vi "Omniax_mDrive_XYZR_2016.vi"() -> ()   [LabVIEW 2014]
uses:
  <vilib>/Utility/file.llb/Read From Spreadsheet File (I64).vi
  <vilib>/Utility/file.llb/Read From Spreadsheet File (string).vi
  <vilib>/Instr/_visa.llb/VISA Configure Serial Port (Instr).vi
  <vilib>/Utility/file.llb/Write To Spreadsheet File (I64).vi
  <vilib>/Utility/file.llb/Write To Spreadsheet File (string).vi
panel:
  in  "Submit":bool
  in  "ELOG":string
  out "Z max step":i32
  in  "V5 position 15360000":i32
  out "R Velocity MVdeg/sec":dbl format="%.3f"
  out "R Position MV deg":dbl
  out "Z Velocity MV mm/sec":dbl format="%.3f"
  out "Z Position MV mm":dbl
  out "Y Velocity MV mm/sec":dbl format="%.3f"
  out "Y Position MV mm":dbl
  out "X Velocity MV mm/sec":dbl format="%.3f"
  out "X Position MV mm":dbl
  out "Presets":i32[][](array[numeric])
  in  "stop":bool
  in  "Tab Control 3":enum32{"Status", "Reset"}(tab)
  out "Y in Range":bool
  out "Y Scan":bool
  out "Y in Motion":bool
  out "Y Backlash corr":bool
  out "X  in Range":bool
  out "X Scan":bool
  out "X  in Motion":bool
  out "X Backlash corr":bool
  out "Z in Range":bool
  out "Z Scan":bool
  out "Z in Motion":bool
  out "Z Backlash corr":bool
  out "R in Range":bool
  out "R Scan":bool
  out "R in Motion":bool
  out "R Backlash corr":bool
  out "X Ready":bool
  out "Y Ready":bool
  out "Z Ready":bool
  out "R Ready":bool
  in  "Reset Y Position mm":dbl
  out "Reset Y Motor Steps":i32
  in  "Reset X Position mm":dbl
  out "Reset X Motor Steps":i32
  in  "Reset Z Position mm":dbl
  out "Reset Z Motor Steps":i32
  in  "Reset R Position deg":dbl
  out "Reset R Motor Steps":i32
  in  "Reset":bool
  in  "Tab Control 2":enum32{"mm", "step"}(tab)
  in  "X Scan Length SP mm":dbl
  in  "X Scan Velocity SP mm/sec":dbl
  in  "X Scan set":bool
  in  "Y Scan Length SP mm":dbl
  in  "Y Scan Velocity SP mm/sec":dbl
  in  "Y Scan set":bool
  in  "Z Scan Length SP mm":dbl
  in  "Z Scan Velocity SP mm/sec":dbl
  in  "Z Scan set":bool
  in  "R Scan Length SP deg":dbl
  in  "R Scan Velocity SP deg/sec":dbl
  in  "R Scan set":bool
  in  "X Scan Velocity SP steps/sec":i32=1 min=1 max=102400 step=1
  in  "X Scan Length SP steps":i32 min=-2816000 max=1792000 step=100
  out "X Scan length MV mm":dbl
  out "X Scan velocity MV mm/sec":dbl format="%#_6f"
  in  "Y Scan Velocity SP steps/sec":i32=1 min=1 max=102400 step=1
  in  "Y Scan Length SP steps":i32 min=-1930240 max=2677760 step=100
  out "Y Scan length MV mm":dbl
  out "Y Scan velocity MV mm/sec":dbl format="%#_6f"
  in  "Z Scan Velocity SP steps/sec":i32=1 min=1 max=102400 step=1
  in  "Z Scan Length SP steps":i32 min=-91980800 max=10419200 step=100
  out "Z Scan length MV mm":dbl
  out "Z Scan velocity MV mm/sec":dbl format="%#_6f"
  in  "R Scan Velocity SP steps/sec":i32=1 min=1 max=102400 step=1
  in  "R Scan Length SP steps":i32 min=-1501867 max=10786133 step=100
  out "R Scan length MV deg":dbl
  out "R Scan velocity MV deg/sec":dbl format="%#_6f"
  out "atan Y/Z":dbl
  in  "Tab Control":enum32{"mm", "preset", "step"}(tab)
  in  "X Position SP mm":dbl
  in  "X Velocity SP mm/sec":dbl
  in  "X Move Set":bool
  in  "Y Move Set":bool
  in  "Y Position SP mm":dbl
  in  "Y Velocity SP mm/sec":dbl
  in  "Z Position SP mm":dbl
  in  "Z Velocity SP mm/sec":dbl
  in  "Z Move Set":bool
  in  "R Position SP deg":dbl
  in  "R Velocity SP deg/sec":dbl
  in  "R Move Set":bool
  in  "Add Button":bool
  in  "String":string
  in  "Delete Button":bool
  in  "Preset positions":i32(ring) items=["ZERO", "Default", "CDOSE", "QMS", "test", "test2", "test3", "yag position", "Sample Long Edge  ", "SPUTTER POS"]
  in  "Set Button":bool
  in  "X Velocity SP step/sec":i32 min=1 max=128000
  in  "Y Velocity SP step/sec":i32 min=1 max=128000
  in  "Z Velocity SP step/sec":i32 min=1 max=204800
  in  "R Velocity SP step/sec":i32 min=1 max=10000
  in  "Y Step SP":i32=-20000 min=-2304000 max=2304000 step=500
  in  "X Step SP":i32=-20000 min=-2304000 max=2304000 step=500
  in  "Z Step SP":i32=-20000 min=0 max=102400000 step=500
  in  "R Step SP":i32=-20000 min=-6144000 max=6144000 step=500
  out "X Step PV":i32 max=2000
  out "Y Step PV":i32 max=2000
  out "Z Step PV":i32 max=2000
  out "R Step PV":i32 max=2000
  in  "Clear ZY":bool
  out "ZY Graph":cluster{"Y":dbl[], "Y":dbl[]}[](graph)
  out "ZR Graph":cluster{"Y":dbl[], "Y":dbl[]}[](graph)
  out "XY Graph":cluster{"Y":dbl[], "Y":dbl[]}[](graph)
  out "X Scan Duration":dbl
  out "Y Scan Duration":dbl
  out "Z Scan Duration":dbl
  out "R Scan Duration":dbl
  out "R Backlash steps/sec":i32
  out "R Backlash":i32
  out "R Holding Current %":i32
  out "R Run Current %":i32
  out "R offset deg":dbl
  out "R deg/rev":dbl
  out "R steps/rev":u32
  out "R velocity PV step/sec":i32
  out "R MINPOS":i32=-94296
  out "R MAXPOS":i32=-34296
  out "R COM PORT":refnum<visa-resource-name>="COM5"
  in  "R Scan OK":bool
  in  "R Go":bool
  out "R Position deg PV":dbl
  out "Z COM PORT":refnum<visa-resource-name>="COM5"
  out "Z Backlash steps/sec":i32
  out "Z Backlash":i32
  out "Z Holding Current %":i32
  out "Z Run Current %":i32
  out "Z offset mm":dbl
  out "Z mm/rev":dbl
  out "Z steps/rev":u32
  out "Z  velocity PV step/sec":i32
  out "Z MINPOS":i32=-94296
  out "Z MAXPOS":i32=-34296
  in  "Z Scan OK":bool
  in  "Z Go":bool
  out "Z Position mm PV":dbl
  out "X Position mm PV":dbl
  out "X velocity PV step/sec":i32
  in  "X Scan OK":bool
  in  "X Go":bool
  out "X Backlash steps/sec":i32
  out "X Backlash":i32
  out "X Holding Current %":i32
  out "X Run Current %":i32
  out "X offset mm":dbl
  out "X mm/rev":dbl
  out "X steps/rev":u32
  out "X MAXPOS":i32=-34296
  out "X MINPOS":i32=-94296
  out "X COM PORT":refnum<visa-resource-name>="COM5"
  out "Y Backlash steps/sec":i32
  out "Y Backlash":i32
  out "Y Holding Current %":i32
  out "Y Run Current %":i32
  in  "Scan Cancel":bool
  out "Y Position mm PV":dbl
  out "Y offset mm":dbl
  out "Y mm/rev":dbl
  out "Y steps/rev":u32
  out "Y velocity PV step/sec":i32
  in  "Y Scan OK":bool
  in  "Scan Go":bool
  in  "Stop":bool
  in  "Y Go":bool
  out "Y MINPOS":i32=-94296
  out "Y MAXPOS":i32=-34296
  out "Y COM PORT":refnum<visa-resource-name>="COM5"
  # "12-15"
  # "Current position"
  # "Goto position"
  # "MX"
  # "MY"
  # "V5"
  # "MZ"
  # "MR"
  # "L"
  # "M"
  # "B"
  # "S"
  # "R"
  # "Preset position"
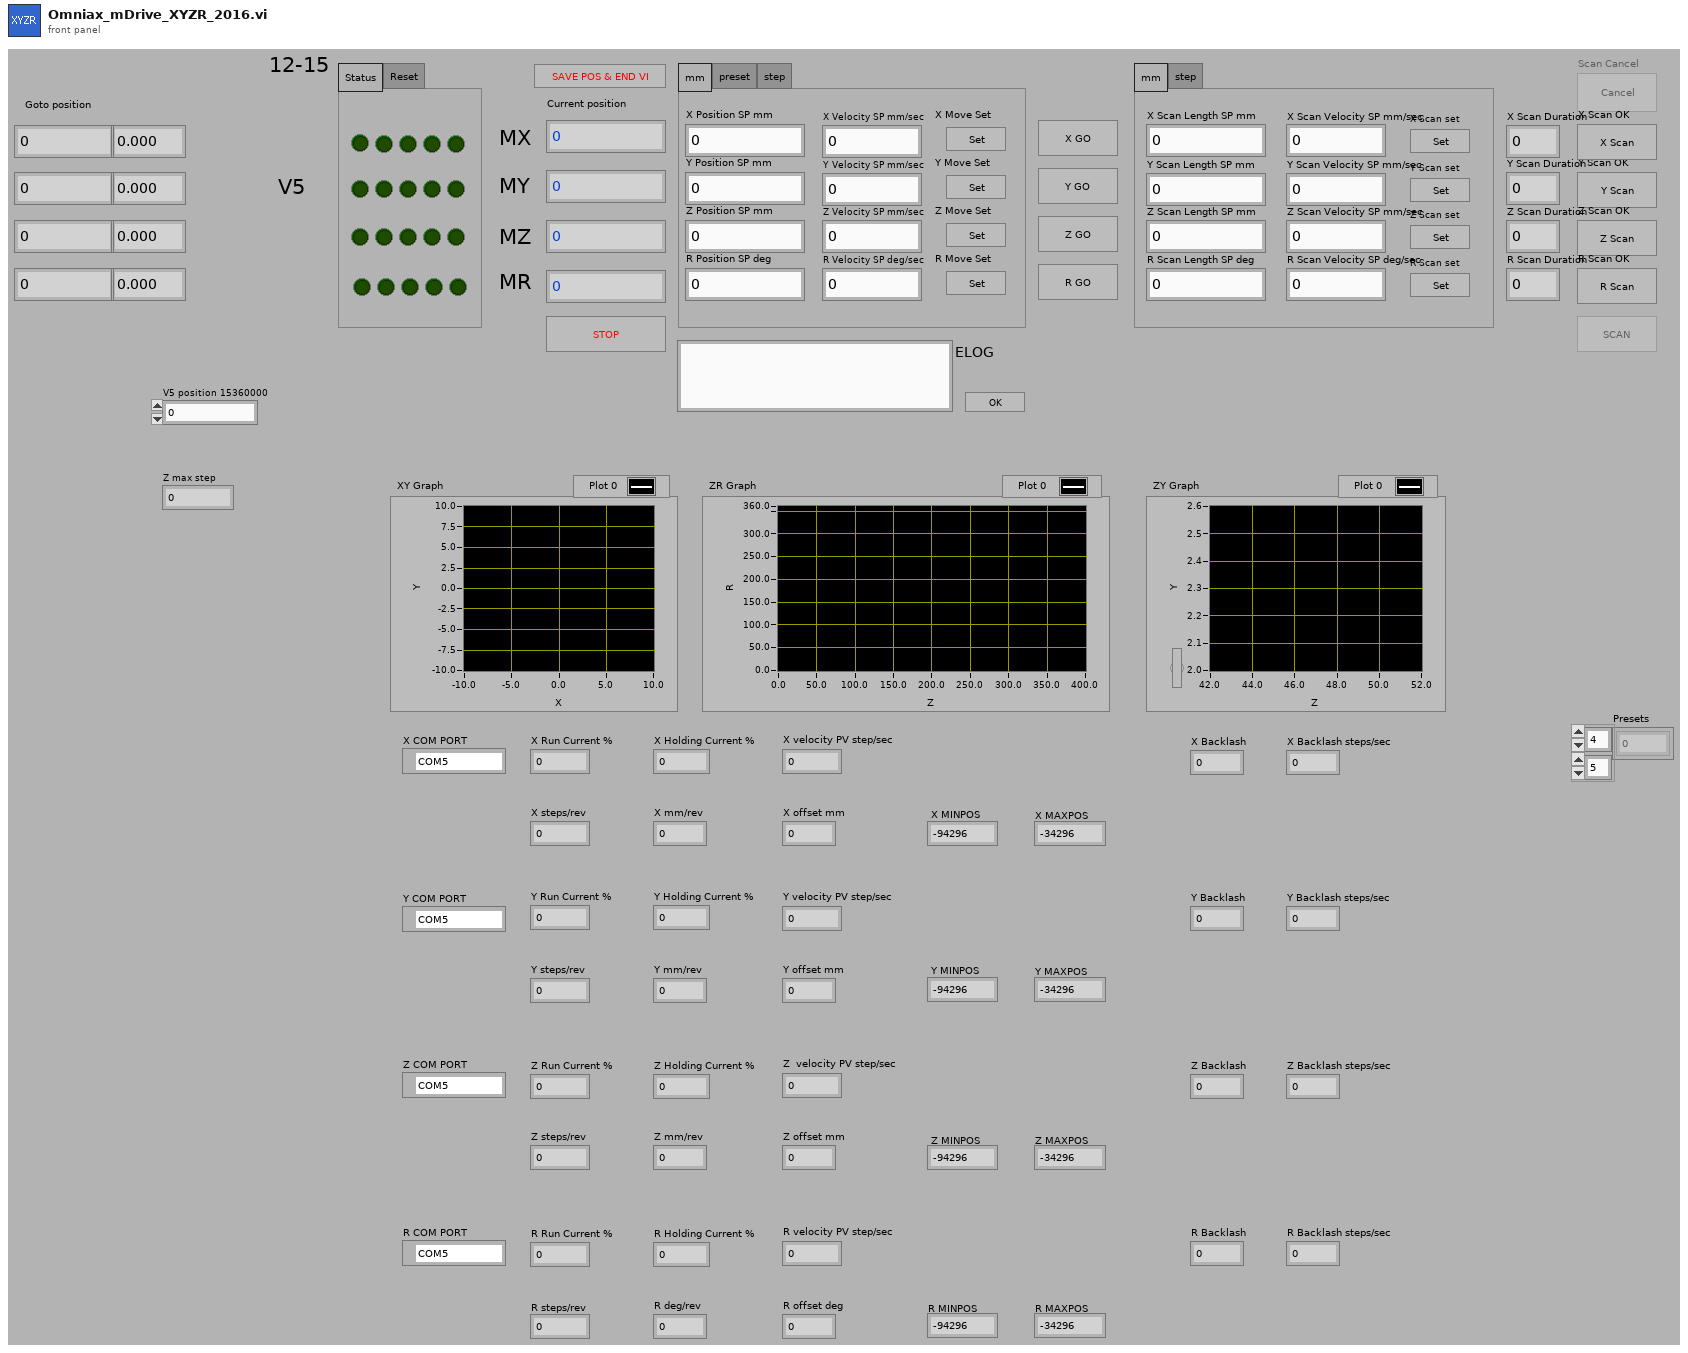
[diagram p1: front panel]
types:
  T1 = enum16{"Stop", "Reset", "Run Current", "Holding Current", "Accel Rate", "Decel Rate", "Move to Relative Position", "Move to Absolute Position", "Echo Mode", "Print Parameter", "Send String", "Microstep Resolution", "Set Current Position", "Max Velocity"}
  T2 = enum8{"Enabled", "Disabled", "Disabled and Grayed Out"}
  T3 = cluster{"first row[0]":i64, "first row[1]":i64, "first row[2]":i64, "first row[3]":i64, "first row[4]":i64, "first row[5]":i64, "first row[6]":i64, "first row[7]":i64, "first row[8]":i64}
  T4 = enum16{"open", "replace", "create", "open or create", "replace or create", "replace or create with confirmation"}
  T5 = cluster{"Value[0]":i32, "Value[1]":i32, "Value[2]":i32, "Value[3]":i32, "Value[4]":i32, "Value[5]":i32, "Value[6]":i32, "Value[7]":i32, "Value[8]":i32}
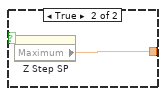
[diagram p7: hidden frame]
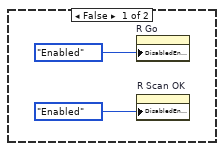
[diagram p9: hidden frame]
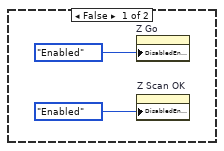
[diagram p12: hidden frame]
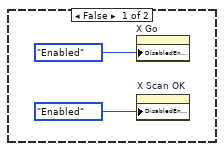
[diagram p15: hidden frame]
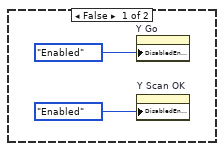
[diagram p18: hidden frame]
diagram:
  w2 = 0 ("dimension size")
  n1 = property on="R Step SP" class="DigNum (strict)"("Maximum"=6144000 ("upper limit")) -> ()  [unwired: 2 in, 2 out]
  n2 = property on="R Step SP" class="DigNum (strict)"("Minimum"=-6144000 ("lower limit")) -> ()  [unwired: 2 in, 2 out]
  n3 = call-poly <vilib>:"Read From Spreadsheet File.vi"("file path (dialog if empty)"=path "S:/SSE/IMS/PRESET.TXT") -> ("all rows"=w8:string[][])  [unwired: 6 in, 4 out]
  n4 = Transpose 2D Array(2D array=w8) -> (transposed array=w9:string[][])
  n5 = flat-sequence {
    tunnel: [w106] -> w36
    tunnel: [w105] -> w35
    tunnel: [w114] -> w54
    tunnel: [w116] -> w52
    tunnel: w36 -> [w115]
    tunnel: w35 -> [w117]
    tunnel: w54 -> [w121]
    tunnel: [w122] -> w53
    tunnel: w52 -> [w120]
    tunnel: [w123] -> w51
    tunnel: [w134] -> w71
    tunnel: [w136] -> w70
    tunnel: w53 -> [w135]
    tunnel: w51 -> [w130]
    tunnel: w71 -> [w143]
    tunnel: [w142] -> w69
    tunnel: w70 -> [w140]
    tunnel: [w141] -> w68
    tunnel: [w153] -> w67
    tunnel: [w154] -> w66
    tunnel: w69 -> [w152]
    tunnel: w68 -> [w151]
    tunnel: w67 -> [w164]
    tunnel: w66 -> [w163]
    tunnel: [w166] -> w65
    tunnel: [w165] -> w64
    tunnel: [w160] -> w63
    tunnel: [w173] -> w59
    tunnel: [w174] -> w60
    tunnel: w65 -> [w174]
    tunnel: w64 -> [w173]
    tunnel: w63 -> [w171]
    frame #0 {
      w113 = refnum<visa-resource-name> "COM13" ("COM PORT")
      w111 = u16 0 items=["None", "XON/XOFF", "RTS/CTS", "XON/XOFF & RTS/CTS", "DTR/DSR", "XON/XOFF & DTR/DSR"] ("flow control (0:none)")
      w110 = u16 10 items=["1.0"=10, "1.5"=15, "2.0"=20] ("stop bits (10: 1 bit)")
      # "Stop bits"
      n6 = call-poly "VISA Configure Serial Port"("VISA resource name"=w113, "timeout (10sec)"=u32 10000, "baud rate (9600)"=u32 9600, "data bits (8)"=u16 8, "parity (0:none)"=enum16{"None", "Odd", "Even", "Mark", "Space"}."None", "stop bits (10: 1 bit)"=w110, "flow control (0:none)"=w111) -> ("VISA resource name out"=w106:refnum<visa-resource-name>, "error out"=w105:errorcluster)  [unwired: 7 in]
      "R COM PORT" <- w113
    }
    frame #1 {
      n7 = call "mDrive Send Command.vi"("error in (no error)"=w117, "Extra"="EM=2", "Command"=T1."Send String", "VISA resource name"=w115) -> ("error out"=w116:errorcluster, "VISA resource name out"=w114:refnum<visa-resource-name>)  [unwired: 3 in, 1 out]
    }
    frame #2 {
      # "pr=1000000"
      n8 = Number To Decimal String(number=100000) -> (decimal integer string=w125:string)  [unwired: 1 in]
      n9 = call "mDrive Send Command.vi"("error in (no error)"=w120, "Extra"=w125, "Command"=T1."Accel Rate", "VISA resource name"=w121) -> ("error out"=w124:errorcluster, "VISA resource name out"=w129:refnum<visa-resource-name>)  [unwired: 3 in, 1 out]
      n10 = call "mDrive Send Command.vi"("error in (no error)"=w124, "Extra"=w125, "Command"=T1."Decel Rate", "VISA resource name"=w129) -> ("error out"=w123:errorcluster, "VISA resource name out"=w122:refnum<visa-resource-name>)  [unwired: 3 in, 1 out]
    }
    frame #3 {
      # "Run Current %"
      n11 = property on="R Run Current %" class="DigNum (strict)"() -> ("Value"=w132:i32)  [unwired: 2 in, 2 out]
      n12 = Number To Decimal String(number=w132) -> (decimal integer string=w133:string)  [unwired: 1 in]
      n13 = call "mDrive Send Command.vi"("error in (no error)"=w130, "Extra"=w133, "Command"=T1."Run Current", "VISA resource name"=w135) -> ("error out"=w136:errorcluster, "VISA resource name out"=w134:refnum<visa-resource-name>)  [unwired: 3 in, 1 out]
    }
    frame #4 {
      # "Holding Current %"
      n14 = property on="R Holding Current %" class="DigNum (strict)"() -> ("Value"=w138:i32)  [unwired: 2 in, 2 out]
      n15 = Number To Decimal String(number=w138) -> (decimal integer string=w139:string)  [unwired: 1 in]
      n16 = call "mDrive Send Command.vi"("error in (no error)"=w140, "Extra"=w139, "Command"=T1."Holding Current", "VISA resource name"=w143) -> ("error out"=w141:errorcluster, "VISA resource name out"=w142:refnum<visa-resource-name>)  [unwired: 3 in, 1 out]
    }
    frame #5 {
      # "Print Velocity Max"
      # "Velocity Max"
      n17 = property on="R Velocity SP step/sec" class="DigNum (strict)"() -> ("Value"=w150:i32)  [unwired: 2 in, 2 out]
      n18 = Number To Decimal String(number=w150) -> (decimal integer string=w149:string)  [unwired: 1 in]
      n19 = call "mDrive Send Command.vi"("error in (no error)"=w151, "Extra"=w149, "Command"=T1."Max Velocity", "VISA resource name"=w152) -> ("error out"=w147:errorcluster, "VISA resource name out"=w157:refnum<visa-resource-name>)  [unwired: 3 in, 1 out]
      n20 = call "mDrive Send Command.vi"("error in (no error)"=w147, "Extra"="VM", "Command"=T1."Print Parameter", "VISA resource name"=w157) -> ("error out"=w154:errorcluster, "read buffer"=w155:string, "VISA resource name out"=w153:refnum<visa-resource-name>)  [unwired: 3 in]
      n21 = Decimal String To Number(string=w155, offset=0) -> (number=w148:i32)  [unwired: 1 in, 1 out]
      n22 = property on="R velocity PV step/sec" class="DigNum (strict)"("Val(Sgnl)"=w148) -> ()  [unwired: 2 in, 2 out]
    }
    frame #6 {
      # "PRINT POSITION"
      n23 = call "mDrive Send Command.vi"("error in (no error)"=w163, "Extra"="P", "Command"=T1."Print Parameter", "VISA resource name"=w164) -> ("error out"=w165:errorcluster, "read buffer"=w162:string, "VISA resource name out"=w166:refnum<visa-resource-name>)  [unwired: 3 in]
      n24 = Decimal String To Number(string=w162, offset=0) -> (number=w160:i32)  [unwired: 1 in, 1 out]
    }
    frame #7 {
      n25 = property on="R Step SP" class="DigNum (strict)"("Val(Sgnl)"=w171) -> ()  [unwired: 2 in, 2 out]
      n26 = property on="R Step SP" class="DigNum (strict)"() -> ("Maximum"=w170:dbl)  [unwired: 2 in, 2 out]
      n27 = property on="R Step SP" class="DigNum (strict)"() -> ("Minimum"=w169:dbl)  [unwired: 2 in, 2 out]
      n28 = To Long Integer(number=w170) -> (32bit integer=w167:i32)
      "R MAXPOS" <- w167
      n29 = To Long Integer(number=w169) -> (32bit integer=w168:i32)
      "R MINPOS" <- w168
      n30 = In Range and Coerce(upper limit=w167, x=w171, lower limit=w168) -> (In Range?=w172:bool)  [unwired: 1 out]
      n31 = property on="R in Range" class="Bool (strict)"("Val(Sgnl)"=w172) -> ()  [unwired: 2 in, 2 out]
    }
  }
  n32 = flat-sequence {
    frame #0 {
      w180 = -3.0 ("R deg/rev")
      w178 = u32 51200 ("step/rev")
      w182 = 10000 ("Value (Signaling)")
      n33 = To Double Precision Float(number=w182) -> (double precision float=w184:dbl)
      n34 = To Double Precision Float(number=w178) -> (double precision float=w179:dbl)
      n35 = property on="R Velocity SP step/sec" class="DigNum (strict)"("Val(Sgnl)"=w182) -> ()  [unwired: 2 in, 2 out]
      n36 = property on="R Velocity SP step/sec" class="DigNum (strict)"("Minimum"=1.0 ("Data Entry Limits:Minimum")) -> ()  [unwired: 2 in, 2 out]
      n37 = Divide(x=w184, y=w179) -> (x/y=w183:dbl)
      n38 = property on="R Velocity SP step/sec" class="DigNum (strict)"("Maximum"=w184) -> ()  [unwired: 2 in, 2 out]
      n39 = Multiply(x=w183, y=w180) -> (x*y=w181:dbl)
      n40 = Absolute Value(x=w181) -> (abs(x)=w175:dbl)
      n41 = property on="R Velocity SP deg/sec" class="DigNum (strict)"("Val(Sgnl)"=w175) -> ()  [unwired: 2 in, 2 out]
      "R offset deg" <- 0.0 ("R offset deg")
      "R deg/rev" <- w180
      "R steps/rev" <- w178
    }
  }
  n42 = flat-sequence {
    frame #0 {
      w186 = 0.2 ("Z mm/rev")
      w185 = u32 51200 ("step/rev")
      w187 = 204800 ("Value (Signaling)")
      n43 = To Double Precision Float(number=w187) -> (double precision float=w191:dbl)
      n44 = To Double Precision Float(number=w185) -> (double precision float=w190:dbl)
      n45 = property on="Z Velocity SP step/sec" class="DigNum (strict)"("Val(Sgnl)"=w187) -> ()  [unwired: 2 in, 2 out]
      n46 = property on="Z Velocity SP step/sec" class="DigNum (strict)"("Minimum"=1.0 ("Data Entry Limits:Minimum")) -> ()  [unwired: 2 in, 2 out]
      n47 = Divide(x=w191, y=w190) -> (x/y=w188:dbl)
      n48 = property on="Z Velocity SP step/sec" class="DigNum (strict)"("Maximum"=w191) -> ()  [unwired: 2 in, 2 out]
      n49 = Multiply(x=w188, y=w186) -> (x*y=w189:dbl)
      n50 = property on="Z Velocity SP mm/sec" class="DigNum (strict)"("Val(Sgnl)"=w189) -> ()  [unwired: 2 in, 2 out]
      "Z offset mm" <- 0.0 ("Z offset mm")
      "Z mm/rev" <- w186
      "Z steps/rev" <- w185
    }
  }
  n51 = flat-sequence {
    frame #0 {
      n52 = property on="X Backlash corr" class="Bool (strict)"("Val(Sgnl)"=FALSE ("Value (Signaling)")) -> ()  [unwired: 2 in, 2 out]
      n53 = property on="Y Backlash corr" class="Bool (strict)"("Val(Sgnl)"=FALSE ("Value (Signaling)")) -> ()  [unwired: 2 in, 2 out]
      n54 = property on="R Backlash corr" class="Bool (strict)"("Val(Sgnl)"=FALSE ("Value (Signaling)")) -> ()  [unwired: 2 in, 2 out]
      n55 = property on="Z Backlash corr" class="Bool (strict)"("Val(Sgnl)"=FALSE ("Value (Signaling)")) -> ()  [unwired: 2 in, 2 out]
      "Z Backlash steps/sec" <- 25600 ("Z Backlash steps/sec")
      "Z Backlash" <- -51200 ("Z Backlash")
      "X Backlash steps/sec" <- 25600 ("Value (Signaling)")
      "X Backlash" <- 10240 ("Backlash2")
      "Y Backlash" <- -10240 ("Backlash2")
      "Y Backlash steps/sec" <- 25600 ("Value (Signaling)")
      "R Backlash steps/sec" <- 6400 ("R Backlash steps/sec")
      "R Backlash" <- -12800 ("R Backlash")
    }
  }
  n56 = flat-sequence {
    frame #0 {
      "Z Holding Current %" <- 20 ("Z Holding Current %")
      "Z Run Current %" <- 40 ("Z Run Current %")
      "X Run Current %" <- 40 ("Run Current %")
      "X Holding Current %" <- 20 ("Holding Current %")
      "Y Run Current %" <- 40 ("Run Current %")
      "Y Holding Current %" <- 20 ("Holding Current %")
      "R Holding Current %" <- 15 ("R Holding Current %")
      "R Run Current %" <- 80 ("R Run Current %")
    }
  }
  n57 = flat-sequence {
    frame #0 {
      n58 = property on="Y Scan" class="Bool (strict)"("Val(Sgnl)"=FALSE ("Value (Signaling)")) -> ()  [unwired: 2 in, 2 out]
      n59 = property on="X Scan Velocity SP mm/sec" class="DigNum (strict)"("Val(Sgnl)"=0.1 ("Value (Signaling)")) -> ()  [unwired: 2 in, 2 out]
      n60 = property on="Z Scan" class="Bool (strict)"("Val(Sgnl)"=FALSE ("Value (Signaling)")) -> ()  [unwired: 2 in, 2 out]
      n61 = property on="X Scan" class="Bool (strict)"("Val(Sgnl)"=FALSE ("Value (Signaling)")) -> ()  [unwired: 2 in, 2 out]
      n62 = property on="Z Scan Velocity SP mm/sec" class="DigNum (strict)"("Val(Sgnl)"=0.1 ("Value (Signaling)")) -> ()  [unwired: 2 in, 2 out]
      n63 = property on="R Velocity SP deg/sec" class="DigNum (strict)"("Val(Sgnl)"=0.1 ("Value (Signaling)")) -> ()  [unwired: 2 in, 2 out]
      n64 = property on="R Scan" class="Bool (strict)"("Val(Sgnl)"=FALSE ("Value (Signaling)")) -> ()  [unwired: 2 in, 2 out]
      n65 = property on="Y Scan Velocity SP mm/sec" class="DigNum (strict)"("Val(Sgnl)"=0.1 ("Value (Signaling)")) -> ()  [unwired: 2 in, 2 out]
      n66 = property on="Scan Go" class="Bool"("DisabledEnum"=T2."Disabled and Grayed Out" ("Disabled")) -> ()  [unwired: 2 in, 2 out]
      n67 = property on="Scan Cancel" class="Bool"("DisabledEnum"=T2."Disabled and Grayed Out" ("Disabled")) -> ()  [unwired: 2 in, 2 out]
    }
  }
  n68 = flat-sequence {
    frame #0 {
      w226 = 0.2 ("MM/rev")
      w229 = u32 51200 ("step/rev")
      w224 = 128000 ("Value (Signaling)")
      # "a=1000000"
      n69 = property on="X Velocity SP step/sec" class="DigNum (strict)"("Minimum"=1.0 ("Data Entry Limits:Minimum")) -> ()  [unwired: 2 in, 2 out]
      n70 = To Double Precision Float(number=w224) -> (double precision float=w230:dbl)
      n71 = To Double Precision Float(number=w229) -> (double precision float=w228:dbl)
      n72 = property on="X Velocity SP step/sec" class="DigNum (strict)"("Val(Sgnl)"=w224) -> ()  [unwired: 2 in, 2 out]
      n73 = Divide(x=w230, y=w228) -> (x/y=w225:dbl)
      n74 = property on="X Velocity SP step/sec" class="DigNum (strict)"("Maximum"=w230) -> ()  [unwired: 2 in, 2 out]
      n75 = Multiply(x=w225, y=w226) -> (x*y=w227:dbl)
      n76 = property on="X Velocity SP mm/sec" class="DigNum (strict)"("Val(Sgnl)"=w227) -> ()  [unwired: 2 in, 2 out]
      "X offset mm" <- 0.0 ("offset")
      "X steps/rev" <- w229
      "X mm/rev" <- w226
    }
  }
  n77 = flat-sequence {
    frame #0 {
      w235 = 0.2 ("MM/rev")
      w238 = u32 51200 ("step/rev")
      w233 = 128000 ("Value (Signaling)")
      n78 = To Double Precision Float(number=w233) -> (double precision float=w239:dbl)
      n79 = To Double Precision Float(number=w238) -> (double precision float=w237:dbl)
      n80 = property on="Y Velocity SP step/sec" class="DigNum (strict)"("Minimum"=1.0 ("Data Entry Limits:Minimum")) -> ()  [unwired: 2 in, 2 out]
      n81 = property on="Y Velocity SP step/sec" class="DigNum (strict)"("Val(Sgnl)"=w233) -> ()  [unwired: 2 in, 2 out]
      n82 = Divide(x=w239, y=w237) -> (x/y=w234:dbl)
      n83 = property on="Y Velocity SP step/sec" class="DigNum (strict)"("Maximum"=w239) -> ()  [unwired: 2 in, 2 out]
      n84 = Multiply(x=w234, y=w235) -> (x*y=w236:dbl)
      n85 = property on="Y Velocity SP mm/sec" class="DigNum (strict)"("Val(Sgnl)"=w236) -> ()  [unwired: 2 in, 2 out]
      "Y offset mm" <- 0.0 ("offset")
      "Y steps/rev" <- w238
      "Y mm/rev" <- w235
    }
  }
  n86 = flat-sequence {
    tunnel: [w242] -> w40
    tunnel: [w243] -> w39
    tunnel: [w253] -> w46
    tunnel: [w252] -> w44
    tunnel: w40 -> [w254]
    tunnel: w39 -> [w251]
    tunnel: w46 -> [w264]
    tunnel: [w259] -> w45
    tunnel: w44 -> [w263]
    tunnel: [w263] -> w43
    tunnel: [w268] -> w80
    tunnel: [w270] -> w79
    tunnel: w45 -> [w269]
    tunnel: w43 -> [w271]
    tunnel: w80 -> [w278]
    tunnel: [w277] -> w78
    tunnel: w79 -> [w275]
    tunnel: [w276] -> w77
    tunnel: [w288] -> w76
    tunnel: [w289] -> w75
    tunnel: w78 -> [w287]
    tunnel: w77 -> [w286]
    tunnel: w76 -> [w299]
    tunnel: w75 -> [w298]
    tunnel: [w301] -> w74
    tunnel: [w300] -> w73
    tunnel: [w295] -> w72
    tunnel: [w308] -> w61
    tunnel: [w309] -> w62
    tunnel: w74 -> [w309]
    tunnel: w73 -> [w308]
    tunnel: w72 -> [w306]
    frame #0 {
      w250 = refnum<visa-resource-name> "COM14" ("COM PORT")
      w248 = u16 0 items=["None", "XON/XOFF", "RTS/CTS", "XON/XOFF & RTS/CTS", "DTR/DSR", "XON/XOFF & DTR/DSR"] ("flow control (0:none)")
      w247 = u16 10 items=["1.0"=10, "1.5"=15, "2.0"=20] ("stop bits (10: 1 bit)")
      # "Stop bits"
      n87 = call-poly "VISA Configure Serial Port"("VISA resource name"=w250, "timeout (10sec)"=u32 10000, "baud rate (9600)"=u32 9600, "data bits (8)"=u16 8, "parity (0:none)"=enum16{"None", "Odd", "Even", "Mark", "Space"}."None", "stop bits (10: 1 bit)"=w247, "flow control (0:none)"=w248) -> ("VISA resource name out"=w242:refnum<visa-resource-name>, "error out"=w243:errorcluster)  [unwired: 7 in]
      "Z COM PORT" <- w250
    }
    frame #1 {
      n88 = call "mDrive Send Command.vi"("error in (no error)"=w251, "Extra"="EM=2", "Command"=T1."Send String", "VISA resource name"=w254) -> ("error out"=w252:errorcluster, "VISA resource name out"=w253:refnum<visa-resource-name>)  [unwired: 3 in, 1 out]
    }
    frame #2 {
      n89 = Number To Decimal String(number=1000000) -> (decimal integer string=w257:string)  [unwired: 1 in]
      n90 = call "mDrive Send Command.vi"("Extra"=w257, "Command"=T1."Accel Rate", "VISA resource name"=w264) -> ("VISA resource name out"=w262:refnum<visa-resource-name>)  [unwired: 4 in, 2 out]
      n91 = call "mDrive Send Command.vi"("Extra"=w257, "Command"=T1."Decel Rate", "VISA resource name"=w262) -> ("VISA resource name out"=w259:refnum<visa-resource-name>)  [unwired: 4 in, 2 out]
    }
    frame #3 {
      # "Run Current %"
      n92 = property on="Z Run Current %" class="DigNum (strict)"() -> ("Value"=w266:i32)  [unwired: 2 in, 2 out]
      n93 = Number To Decimal String(number=w266) -> (decimal integer string=w267:string)  [unwired: 1 in]
      n94 = call "mDrive Send Command.vi"("error in (no error)"=w271, "Extra"=w267, "Command"=T1."Run Current", "VISA resource name"=w269) -> ("error out"=w270:errorcluster, "VISA resource name out"=w268:refnum<visa-resource-name>)  [unwired: 3 in, 1 out]
    }
    frame #4 {
      # "Holding Current %"
      n95 = property on="Z Run Current %" class="DigNum (strict)"() -> ("Value"=w273:i32)  [unwired: 2 in, 2 out]
      n96 = Number To Decimal String(number=w273) -> (decimal integer string=w274:string)  [unwired: 1 in]
      n97 = call "mDrive Send Command.vi"("error in (no error)"=w275, "Extra"=w274, "Command"=T1."Holding Current", "VISA resource name"=w278) -> ("error out"=w276:errorcluster, "VISA resource name out"=w277:refnum<visa-resource-name>)  [unwired: 3 in, 1 out]
    }
    frame #5 {
      # "Velocity Max"
      n98 = property on="Z Velocity SP step/sec" class="DigNum (strict)"() -> ("Value"=w285:i32)  [unwired: 2 in, 2 out]
      n99 = Number To Decimal String(number=w285) -> (decimal integer string=w284:string)  [unwired: 1 in]
      n100 = call "mDrive Send Command.vi"("error in (no error)"=w286, "Extra"=w284, "Command"=T1."Max Velocity", "VISA resource name"=w287) -> ("error out"=w282:errorcluster, "VISA resource name out"=w292:refnum<visa-resource-name>)  [unwired: 3 in, 1 out]
      n101 = call "mDrive Send Command.vi"("error in (no error)"=w282, "Extra"="VM", "Command"=T1."Print Parameter", "VISA resource name"=w292) -> ("error out"=w289:errorcluster, "read buffer"=w290:string, "VISA resource name out"=w288:refnum<visa-resource-name>)  [unwired: 3 in]
      n102 = Decimal String To Number(string=w290, offset=0) -> (number=w283:i32)  [unwired: 1 in, 1 out]
      n103 = property on="Z  velocity PV step/sec" class="DigNum (strict)"("Val(Sgnl)"=w283) -> ()  [unwired: 2 in, 2 out]
    }
    frame #6 {
      # "PRINT POSITION"
      n104 = call "mDrive Send Command.vi"("error in (no error)"=w298, "Extra"="P", "Command"=T1."Print Parameter", "VISA resource name"=w299) -> ("error out"=w300:errorcluster, "read buffer"=w297:string, "VISA resource name out"=w301:refnum<visa-resource-name>)  [unwired: 3 in]
      n105 = Decimal String To Number(string=w297, offset=0) -> (number=w295:i32)  [unwired: 1 in, 1 out]
    }
    frame #7 {
      n106 = property on="Z Step SP" class="DigNum (strict)"("Val(Sgnl)"=w306) -> ()  [unwired: 2 in, 2 out]
      n107 = property on="Z Step SP" class="DigNum (strict)"() -> ("Maximum"=w303:dbl)  [unwired: 2 in, 2 out]
      n108 = property on="Z Step SP" class="DigNum (strict)"() -> ("Minimum"=w305:dbl)  [unwired: 2 in, 2 out]
      n109 = To Long Integer(number=w303) -> (32bit integer=w304:i32)
      "Z MAXPOS" <- w304
      n110 = To Long Integer(number=w305) -> (32bit integer=w302:i32)
      "Z MINPOS" <- w302
      n111 = In Range and Coerce(upper limit=w304, x=w306, lower limit=w302) -> (In Range?=w307:bool)  [unwired: 1 out]
      n112 = property on="Z in Range" class="Bool (strict)"("Val(Sgnl)"=w307) -> ()  [unwired: 2 in, 2 out]
    }
  }
  n113 = flat-sequence {
    tunnel: [w311] -> w34
    tunnel: [w310] -> w33
    tunnel: [w321] -> w50
    tunnel: [w319] -> w48
    tunnel: w34 -> [w322]
    tunnel: w33 -> [w320]
    tunnel: w50 -> [w328]
    tunnel: [w329] -> w49
    tunnel: w48 -> [w325]
    tunnel: [w327] -> w47
    tunnel: [w338] -> w100
    tunnel: [w340] -> w98
    tunnel: w49 -> [w339]
    tunnel: w47 -> [w341]
    tunnel: w100 -> [w348]
    tunnel: [w347] -> w99
    tunnel: w98 -> [w345]
    tunnel: [w346] -> w97
    tunnel: [w358] -> w102
    tunnel: [w359] -> w101
    tunnel: w99 -> [w357]
    tunnel: w97 -> [w356]
    tunnel: w102 -> [w369]
    tunnel: w101 -> [w368]
    tunnel: [w371] -> w86
    tunnel: [w370] -> w85
    tunnel: [w365] -> w84
    tunnel: [w376] -> w103
    tunnel: [w377] -> w104
    tunnel: w86 -> [w377]
    tunnel: w85 -> [w376]
    tunnel: w84 -> [w372]
    frame #0 {
      w318 = refnum<visa-resource-name> "COM13" ("COM PORT")
      w316 = u16 0 items=["None", "XON/XOFF", "RTS/CTS", "XON/XOFF & RTS/CTS", "DTR/DSR", "XON/XOFF & DTR/DSR"] ("flow control (0:none)")
      w315 = u16 10 items=["1.0"=10, "1.5"=15, "2.0"=20] ("stop bits (10: 1 bit)")
      # "Stop bits"
      n114 = call-poly "VISA Configure Serial Port"("VISA resource name"=w318, "timeout (10sec)"=u32 10000, "baud rate (9600)"=u32 9600, "data bits (8)"=u16 8, "parity (0:none)"=enum16{"None", "Odd", "Even", "Mark", "Space"}."None", "stop bits (10: 1 bit)"=w315, "flow control (0:none)"=w316) -> ("VISA resource name out"=w311:refnum<visa-resource-name>, "error out"=w310:errorcluster)  [unwired: 7 in]
      "Y COM PORT" <- w318
    }
    frame #1 {
      n115 = call "mDrive Send Command.vi"("error in (no error)"=w320, "Extra"="EM=2", "Command"=T1."Send String", "VISA resource name"=w322) -> ("error out"=w319:errorcluster, "VISA resource name out"=w321:refnum<visa-resource-name>)  [unwired: 3 in, 1 out]
    }
    frame #2 {
      n116 = Number To Decimal String(number=1000000) -> (decimal integer string=w330:string)  [unwired: 1 in]
      n117 = call "mDrive Send Command.vi"("error in (no error)"=w325, "Extra"=w330, "Command"=T1."Accel Rate", "VISA resource name"=w328) -> ("error out"=w326:errorcluster, "VISA resource name out"=w334:refnum<visa-resource-name>)  [unwired: 3 in, 1 out]
      n118 = call "mDrive Send Command.vi"("error in (no error)"=w326, "Extra"=w330, "Command"=T1."Decel Rate", "VISA resource name"=w334) -> ("error out"=w327:errorcluster, "VISA resource name out"=w329:refnum<visa-resource-name>)  [unwired: 3 in, 1 out]
    }
    frame #3 {
      # "Run Current %"
      n119 = property on="Y Run Current %" class="DigNum (strict)"() -> ("Value"=w336:i32)  [unwired: 2 in, 2 out]
      n120 = Number To Decimal String(number=w336) -> (decimal integer string=w337:string)  [unwired: 1 in]
      n121 = call "mDrive Send Command.vi"("error in (no error)"=w341, "Extra"=w337, "Command"=T1."Run Current", "VISA resource name"=w339) -> ("error out"=w340:errorcluster, "VISA resource name out"=w338:refnum<visa-resource-name>)  [unwired: 3 in, 1 out]
    }
    frame #4 {
      # "Holding Current %"
      n122 = property on="Y Holding Current %" class="DigNum (strict)"() -> ("Value"=w343:i32)  [unwired: 2 in, 2 out]
      n123 = Number To Decimal String(number=w343) -> (decimal integer string=w344:string)  [unwired: 1 in]
      n124 = call "mDrive Send Command.vi"("error in (no error)"=w345, "Extra"=w344, "Command"=T1."Holding Current", "VISA resource name"=w348) -> ("error out"=w346:errorcluster, "VISA resource name out"=w347:refnum<visa-resource-name>)  [unwired: 3 in, 1 out]
    }
    frame #5 {
      # "Velocity Max"
      n125 = property on="Y Velocity SP step/sec" class="DigNum (strict)"() -> ("Value"=w355:i32)  [unwired: 2 in, 2 out]
      n126 = Number To Decimal String(number=w355) -> (decimal integer string=w354:string)  [unwired: 1 in]
      n127 = call "mDrive Send Command.vi"("error in (no error)"=w356, "Extra"=w354, "Command"=T1."Max Velocity", "VISA resource name"=w357) -> ("error out"=w352:errorcluster, "VISA resource name out"=w362:refnum<visa-resource-name>)  [unwired: 3 in, 1 out]
      n128 = call "mDrive Send Command.vi"("error in (no error)"=w352, "Extra"="VM", "Command"=T1."Print Parameter", "VISA resource name"=w362) -> ("error out"=w359:errorcluster, "read buffer"=w360:string, "VISA resource name out"=w358:refnum<visa-resource-name>)  [unwired: 3 in]
      n129 = Decimal String To Number(string=w360, offset=0) -> (number=w353:i32)  [unwired: 1 in, 1 out]
      n130 = property on="Y scan velocity MV step/sec" class="DigNum (strict)"("Val(Sgnl)"=w353) -> ()  [unwired: 2 in, 2 out]
    }
    frame #6 {
      # "PRINT POSITION"
      n131 = call "mDrive Send Command.vi"("error in (no error)"=w368, "Extra"="P", "Command"=T1."Print Parameter", "VISA resource name"=w369) -> ("error out"=w370:errorcluster, "read buffer"=w367:string, "VISA resource name out"=w371:refnum<visa-resource-name>)  [unwired: 3 in]
      n132 = Decimal String To Number(string=w367, offset=0) -> (number=w365:i32)  [unwired: 1 in, 1 out]
    }
    frame #7 {
      w374 = -2304000 ("lower limit")
      w375 = 2304000 ("upper limit")
      n133 = property on="Y Step SP" class="DigNum (strict)"("Val(Sgnl)"=w372) -> ()  [unwired: 2 in, 2 out]
      n134 = property on="Y Step SP" class="DigNum (strict)"("Maximum"=w375) -> ()  [unwired: 2 in, 2 out]
      n135 = property on="Y Step SP" class="DigNum (strict)"("Minimum"=w374) -> ()  [unwired: 2 in, 2 out]
      n136 = In Range and Coerce(upper limit=w375, x=w372, lower limit=w374) -> (In Range?=w373:bool)  [unwired: 1 out]
      n137 = property on="Y in Range" class="Bool (strict)"("Val(Sgnl)"=w373) -> ()  [unwired: 2 in, 2 out]
      "Y MINPOS" <- w374
      "Y MAXPOS" <- w375
    }
  }
  n138 = property on="Z Step SP" class="DigNum (strict)"("Minimum"=0 ("lower limit")) -> ()  [unwired: 2 in, 2 out]
  n139 = Delete From Array(array=w9, index (row)=0) -> (deleted portion=w10:string[], array with subset deleted=w12:string[][])  [unwired: 2 in]
  n140 = flat-sequence {
    tunnel: [w379] -> w38
    tunnel: [w378] -> w37
    tunnel: [w389] -> w58
    tunnel: [w387] -> w56
    tunnel: w38 -> [w390]
    tunnel: w37 -> [w388]
    tunnel: w58 -> [w394]
    tunnel: [w393] -> w57
    tunnel: w56 -> [w395]
    tunnel: [w397] -> w55
    tunnel: [w406] -> w96
    tunnel: [w408] -> w95
    tunnel: w57 -> [w407]
    tunnel: w55 -> [w409]
    tunnel: w96 -> [w416]
    tunnel: [w415] -> w94
    tunnel: w95 -> [w413]
    tunnel: [w414] -> w93
    tunnel: [w426] -> w92
    tunnel: [w427] -> w91
    tunnel: w94 -> [w425]
    tunnel: w93 -> [w424]
    tunnel: w92 -> [w437]
    tunnel: w91 -> [w436]
    tunnel: [w439] -> w83
    tunnel: [w438] -> w82
    tunnel: [w433] -> w81
    tunnel: [w444] -> w89
    tunnel: [w445] -> w90
    tunnel: w83 -> [w445]
    tunnel: w82 -> [w444]
    tunnel: w81 -> [w440]
    frame #0 {
      w386 = refnum<visa-resource-name> "COM12" ("COM PORT")
      w384 = u16 0 items=["None", "XON/XOFF", "RTS/CTS", "XON/XOFF & RTS/CTS", "DTR/DSR", "XON/XOFF & DTR/DSR"] ("flow control (0:none)")
      w383 = u16 10 items=["1.0"=10, "1.5"=15, "2.0"=20] ("stop bits (10: 1 bit)")
      # "Stop bits"
      n141 = call-poly "VISA Configure Serial Port"("VISA resource name"=w386, "timeout (10sec)"=u32 10000, "baud rate (9600)"=u32 9600, "data bits (8)"=u16 8, "parity (0:none)"=enum16{"None", "Odd", "Even", "Mark", "Space"}."None", "stop bits (10: 1 bit)"=w383, "flow control (0:none)"=w384) -> ("VISA resource name out"=w379:refnum<visa-resource-name>, "error out"=w378:errorcluster)  [unwired: 7 in]
      "X COM PORT" <- w386
    }
    frame #1 {
      n142 = call "mDrive Send Command.vi"("error in (no error)"=w388, "Extra"="EM=2", "Command"=T1."Send String", "VISA resource name"=w390) -> ("error out"=w387:errorcluster, "VISA resource name out"=w389:refnum<visa-resource-name>)  [unwired: 3 in, 1 out]
    }
    frame #2 {
      n143 = Number To Decimal String(number=1000000) -> (decimal integer string=w398:string)  [unwired: 1 in]
      n144 = call "mDrive Send Command.vi"("error in (no error)"=w395, "Extra"=w398, "Command"=T1."Accel Rate", "VISA resource name"=w394) -> ("error out"=w396:errorcluster, "VISA resource name out"=w402:refnum<visa-resource-name>)  [unwired: 3 in, 1 out]
      n145 = call "mDrive Send Command.vi"("error in (no error)"=w396, "Extra"=w398, "Command"=T1."Decel Rate", "VISA resource name"=w402) -> ("error out"=w397:errorcluster, "VISA resource name out"=w393:refnum<visa-resource-name>)  [unwired: 3 in, 1 out]
    }
    frame #3 {
      # "Run Current %"
      n146 = property on="X Run Current %" class="DigNum (strict)"() -> ("Value"=w404:i32)  [unwired: 2 in, 2 out]
      n147 = Number To Decimal String(number=w404) -> (decimal integer string=w405:string)  [unwired: 1 in]
      n148 = call "mDrive Send Command.vi"("error in (no error)"=w409, "Extra"=w405, "Command"=T1."Run Current", "VISA resource name"=w407) -> ("error out"=w408:errorcluster, "VISA resource name out"=w406:refnum<visa-resource-name>)  [unwired: 3 in, 1 out]
    }
    frame #4 {
      # "Holding Current %"
      n149 = property on="X Holding Current %" class="DigNum (strict)"() -> ("Value"=w411:i32)  [unwired: 2 in, 2 out]
      n150 = Number To Decimal String(number=w411) -> (decimal integer string=w412:string)  [unwired: 1 in]
      n151 = call "mDrive Send Command.vi"("error in (no error)"=w413, "Extra"=w412, "Command"=T1."Holding Current", "VISA resource name"=w416) -> ("error out"=w414:errorcluster, "VISA resource name out"=w415:refnum<visa-resource-name>)  [unwired: 3 in, 1 out]
    }
    frame #5 {
      # "Velocity Max"
      n152 = property on="X Velocity SP step/sec" class="DigNum (strict)"() -> ("Value"=w423:i32)  [unwired: 2 in, 2 out]
      n153 = Number To Decimal String(number=w423) -> (decimal integer string=w422:string)  [unwired: 1 in]
      n154 = call "mDrive Send Command.vi"("error in (no error)"=w424, "Extra"=w422, "Command"=T1."Max Velocity", "VISA resource name"=w425) -> ("error out"=w420:errorcluster, "VISA resource name out"=w430:refnum<visa-resource-name>)  [unwired: 3 in, 1 out]
      n155 = call "mDrive Send Command.vi"("error in (no error)"=w420, "Extra"="VM", "Command"=T1."Print Parameter", "VISA resource name"=w430) -> ("error out"=w427:errorcluster, "read buffer"=w428:string, "VISA resource name out"=w426:refnum<visa-resource-name>)  [unwired: 3 in]
      n156 = Decimal String To Number(string=w428, offset=0) -> (number=w421:i32)  [unwired: 1 in, 1 out]
      n157 = property on="X velocity PV step/sec" class="DigNum (strict)"("Val(Sgnl)"=w421) -> ()  [unwired: 2 in, 2 out]
    }
    frame #6 {
      # "PRINT POSITION"
      n158 = call "mDrive Send Command.vi"("error in (no error)"=w436, "Extra"="P", "Command"=T1."Print Parameter", "VISA resource name"=w437) -> ("error out"=w438:errorcluster, "read buffer"=w435:string, "VISA resource name out"=w439:refnum<visa-resource-name>)  [unwired: 3 in]
      n159 = Decimal String To Number(string=w435, offset=0) -> (number=w433:i32)  [unwired: 1 in, 1 out]
    }
    frame #7 {
      w442 = -2304000 ("lower limit")
      w443 = 2304000 ("upper limit")
      n160 = property on="X Step SP" class="DigNum (strict)"("Val(Sgnl)"=w440) -> ()  [unwired: 2 in, 2 out]
      n161 = property on="X Step SP" class="DigNum (strict)"("Maximum"=w443) -> ()  [unwired: 2 in, 2 out]
      n162 = In Range and Coerce(upper limit=w443, x=w440, lower limit=w442) -> (In Range?=w441:bool)  [unwired: 1 out]
      n163 = property on="X Step SP" class="DigNum (strict)"("Minimum"=w442) -> ()  [unwired: 2 in, 2 out]
      n164 = property on="X  in Range" class="Bool (strict)"("Val(Sgnl)"=w441) -> ()  [unwired: 2 in, 2 out]
      "X MINPOS" <- w442
      "X MAXPOS" <- w443
    }
  }
  n165 = property on="Z Step SP" class="DigNum (strict)"("Maximum"=102400000 ("upper limit")) -> ()  [unwired: 2 in, 2 out]
  n166 = Transpose 2D Array(2D array=w12) -> (transposed array=w13:string[][])
  n167 = property on="Preset positions" class="Ring (strict)"("Strings []"=w10) -> ()  [unwired: 2 in, 2 out]
  n168 = Decimal String To Number(string=w13) -> (number=w11:i32[][])  [unwired: 2 in, 1 out]
  n169 = Initialize Array(w2, w2, 4 ("dimension size")) -> (w5:i32[][])
  n170 = call-poly <vilib>:"Read From Spreadsheet File.vi"("file path (dialog if empty)"=path "S:/SSE/IMS/POS.TXT") -> ("first row"=w20:i64[])  [unwired: 6 in, 4 out]
  n171 = Build Array (concatenate)(w5, w11) -> (→"Presets":i32[][])
  n172 = Array To Cluster(array=w20) -> (cluster=w19:T3)
  n173 = Unbundle(w19) -> ("first row[0]"=w17:i64, "first row[1]"=w16:i64, "first row[2]"=w15:i64, "first row[3]"=w14:i64)  [unwired: 5 out]
  n174 = property on="Reset X Motor Steps" class="DigNum (strict)"("Val(Sgnl)"=w17) -> ()  [unwired: 2 in, 2 out]
  n175 = property on="Reset Y Motor Steps" class="DigNum (strict)"("Val(Sgnl)"=w16) -> ()  [unwired: 2 in, 2 out]
  n176 = property on="Reset Z Motor Steps" class="DigNum (strict)"("Val(Sgnl)"=w15) -> ()  [unwired: 2 in, 2 out]
  n177 = property on="Reset R Motor Steps" class="DigNum (strict)"("Val(Sgnl)"=w14) -> ()  [unwired: 2 in, 2 out]
  n178 = property on="V5 position 15360000" class="DigNum (strict)"("Value"=15360000 ("V5 position 15360000")) -> ()  [unwired: 2 in, 2 out]
  n179 = while {
    tunnel: w104 -> [w466]
    tunnel: w103 -> [w469]
    tunnel: [w470] -> w27
    tunnel: [w468] -> w28
    tunnel: w90 -> [w465]
    tunnel: w89 -> [w464]
    tunnel: [w463] -> w88
    tunnel: [w462] -> w87
    tunnel: w62 -> [w461]
    tunnel: w61 -> [w460]
    tunnel: [w459] -> w30
    tunnel: [w458] -> w29
    tunnel: w60 -> [w457]
    tunnel: w59 -> [w456]
    tunnel: [w455] -> w26
    tunnel: [w454] -> w25
    stop <- "stop" stop-if-true
    n180 = property on="Preset positions" class="Ring (strict)"() -> ("Strings []"=w450:string[])  [unwired: 2 in, 2 out]
    n181 = case shown="True" "Submit" {
      tunnel: "ELOG" -> [_ w474]
      frame False {
      }
      frame True {
        n182 = Open/Create/Replace File(file path (use dialog)=path "S:/ELOG/SSE.LOG", operation (0:open)=T4."replace or create") -> (refnum out=w471:refnum<file>)  [unwired: 4 in, 2 out]
        n183 = flat-sequence {
          tunnel: w471 -> [w491]
          tunnel: w474 -> [w478]
          frame #0 {
            n184 = property on="R Position deg PV" class="DigNum (strict)"() -> ("Value"=w476:dbl)  [unwired: 2 in, 2 out]
            n185 = Number To Fractional String(number=w476) -> (F-format string=w475:string)  [unwired: 3 in]
            n186 = property on="X Position mm PV" class="DigNum (strict)"() -> ("Value"=w488:dbl)  [unwired: 2 in, 2 out]
            n187 = property on="Y Position mm PV" class="DigNum (strict)"() -> ("Value"=w487:dbl)  [unwired: 2 in, 2 out]
            n188 = property on="Z Position mm PV" class="DigNum (strict)"() -> ("Value"=w486:dbl)  [unwired: 2 in, 2 out]
            n189 = Number To Fractional String(number=w488) -> (F-format string=w484:string)  [unwired: 3 in]
            n190 = Number To Fractional String(number=w487) -> (F-format string=w482:string)  [unwired: 3 in]
            n191 = Number To Fractional String(number=w486) -> (F-format string=w480:string)  [unwired: 3 in]
            n192 = Concatenate Strings("MX=" ("string"), w484, " MY=" ("string"), w482, " MZ=" ("string"), w480, " MR= " ("string"), w475, " > " ("string"), w478) -> (w490:string)
            n193 = Write to Text File(file (use dialog)=w491, text=w490) -> (refnum out=w489:refnum<file>)  [unwired: 2 in, 2 out]
            n194 = Close File(refnum=w489) -> ()  [unwired: 1 in, 2 out]
          }
          frame #1 {
            n195 = disable-structure shown="Disabled" {
              frame Disabled {
                n196 = call <vilib>:"System Exec.vi"("working directory"=path "S:/ELOG", "command line"="S:\\elog\\elog.exe -h bl132pc -p 8080 -l \"BL13-2 SSE\" -w beam$2012 -s -a Type=\"Log ES setting\" -a Author=\"Omniax L\" -a Subject=\"Note\" -m SSE.LOG") -> ()  [unwired: 6 in, 4 out]
              }
              frame Enabled {
              }
            }
          }
        }
      }
    }
    n197 = event shown="[0] Timeout" {
      selector: _ -> [_ _ _ _ _ _ _ _ _ _ _ _ _ _ _ _ _ _ _ _ _ _ _ _ _]
      dyn-events: _ -> [_ _ _ _ _ _ _ _ _ _ _ _ _ _ _ _ _ _ _ _ _ _ _ _ _]
      timeout: 100 -> [_ _ _ _ _ _ _ _ _ _ _ _ _ _ _ _ _ _ _ _ _ _ _ _ _]
      tunnel: w469 -> [w594 _ _ _ _ _ _ _ _ _ _ _ w1438 _ _ _ _ w1687 _ _ w1782 w1798 w1842 w1919 w2163]
      tunnel: [w593 _ _ _ _ _ _ _ _ _ _ _ w1444 _ _ _ _ w1685 _ _ w1782 w1796 w1844 w1908 w2161] -> w470
      tunnel: w466 -> [w532 _ _ _ _ _ _ _ _ _ _ _ w1439 _ _ _ _ w1686 _ _ w1783 w1799 w1843 w1921 w2164]
      tunnel: [w592 _ _ _ _ _ _ _ _ _ _ _ w1445 _ _ _ _ w1682 _ _ w1783 w1797 w1845 w1909 w2162] -> w468
      tunnel: w465 -> [w531 _ _ _ _ _ _ _ _ _ _ _ _ _ _ w1596 w1651 _ _ _ _ w1793 w1835 w1925 w2160]
      tunnel: w464 -> [w569 _ _ _ _ _ _ _ _ _ _ _ _ _ _ w1595 w1650 _ _ _ _ w1792 w1834 w1923 w2159]
      tunnel: [w568 _ _ _ _ _ _ _ _ _ _ _ _ _ _ w1594 w1649 _ _ _ _ w1795 w1833 w1901 w2158] -> w463
      tunnel: [w567 _ _ _ _ _ _ _ _ _ _ _ _ _ _ w1593 w1648 _ _ _ _ w1794 w1832 w1899 w2157] -> w462
      tunnel: w461 -> [w541 _ _ _ _ _ _ _ _ _ _ _ _ w1490 _ _ _ _ w1717 _ _ w1791 w1829 w1917 w2156]
      tunnel: w460 -> [w544 _ _ _ _ _ _ _ _ _ _ _ _ w1489 _ _ _ _ w1716 _ _ w1790 w1828 w1915 w2155]
      tunnel: [w543 _ _ _ _ _ _ _ _ _ _ _ _ w1487 _ _ _ _ w1714 _ _ w1789 w1827 w1907 w2152] -> w459
      tunnel: [w542 _ _ _ _ _ _ _ _ _ _ _ _ w1488 _ _ _ _ w1715 _ _ w1788 w1826 w1906 w2151] -> w458
      tunnel: w457 -> [w540 _ _ _ _ _ _ _ _ _ _ _ _ _ w1543 _ _ _ _ w1751 _ w1787 w1823 w1912 w2154]
      tunnel: w456 -> [w539 _ _ _ _ _ _ _ _ _ _ _ _ _ w1542 _ _ _ _ w1750 _ w1786 w1822 w1910 w2153]
      tunnel: [w538 _ _ _ _ _ _ _ _ _ _ _ _ _ w1540 _ _ _ _ w1749 _ w1785 w1821 w1904 w2150] -> w455
      tunnel: [w537 _ _ _ _ _ _ _ _ _ _ _ _ _ w1541 _ _ _ _ w1748 _ w1784 w1820 w1903 w2149] -> w454
      event Timeout {
        n198 = event-data() -> ()  [unwired: 1 in, 2 out]
        n199 = flat-sequence {
          tunnel: [w893] -> w580
          tunnel: [w871] -> w579
          tunnel: [w882] -> w578
          tunnel: [w862] -> w577
          tunnel: w531 -> [w861]
          tunnel: w569 -> [w860]
          tunnel: w580 -> [w899]
          tunnel: [w899] -> w576
          tunnel: w579 -> [w898]
          tunnel: [w898] -> w575
          tunnel: w578 -> [w897]
          tunnel: [w897] -> w574
          tunnel: w577 -> [w894]
          tunnel: [w894] -> w573
          tunnel: w576 -> [w906]
          tunnel: [w907] -> w572
          tunnel: w575 -> [w909]
          tunnel: [w908] -> w571
          tunnel: w574 -> [w905]
          tunnel: [w904] -> w570
          tunnel: w573 -> [w904]
          tunnel: w572 -> [w919]
          tunnel: w571 -> [w920]
          tunnel: w570 -> [w922]
          tunnel: [w918] -> w567
          tunnel: [w917] -> w568
          frame #0 {
            w866 = 0.1 ("Delay Time (s)")
            n200 = property on="X Step SP" class="DigNum (strict)"() -> ("Maximum"=w884:dbl)  [unwired: 2 in, 2 out]
            n201 = property on="X Step SP" class="DigNum (strict)"() -> ("Minimum"=w886:dbl)  [unwired: 2 in, 2 out]
            n202 = property on="X steps/rev" class="DigNum (strict)"() -> ("Value"=w880:u32)  [unwired: 2 in, 2 out]
            n203 = property on="X offset mm" class="DigNum (strict)"() -> ("Value"=w876:dbl)  [unwired: 2 in, 2 out]
            n204 = To Long Integer(number=w884) -> (32bit integer=w883:i32)
            n205 = To Long Integer(number=w886) -> (32bit integer=w885:i32)
            n206 = To Double Precision Float(number=w880) -> (double precision float=w881:dbl)
            n207 = call "mDrive Send Command.vi"("error in (no error)"=w860, "Extra"="P", "Command"=T1."Print Parameter", "VISA resource name"=w861) -> ("error out"=w888:errorcluster, "read buffer"=w892:string, "VISA resource name out"=w890:refnum<visa-resource-name>)  [unwired: 3 in]
            n208 = call "Time Delay12"("error in (no error)"=w888, "Delay Time (s)"=w866) -> ("error out"=w887:errorcluster)  [unwired: 9 in]
            n209 = Decimal String To Number(string=w892, offset=0) -> (number=w873:i32)  [unwired: 1 in, 1 out]
            n210 = To Long Integer(number=w873) -> (32bit integer=w874:i32)
            n211 = property on="X Step PV" class="DigNum (strict)"("Val(Sgnl)"=w874) -> ()  [unwired: 2 in, 2 out]
            n212 = call "mDrive Send Command.vi"("error in (no error)"=w887, "Extra"="MV", "Command"=T1."Print Parameter", "VISA resource name"=w890) -> ("error out"=w889:errorcluster, "read buffer"=w859:string, "VISA resource name out"=w893:refnum<visa-resource-name>)  [unwired: 3 in]
            n213 = call "Time Delay11"("error in (no error)"=w889, "Delay Time (s)"=w866) -> ("error out"=w871:errorcluster)  [unwired: 9 in]
            n214 = In Range and Coerce(upper limit=w883, x=w874, lower limit=w885) -> (In Range?=w882:bool)  [unwired: 1 out]
            n215 = To Double Precision Float(number=w874) -> (double precision float=w875:dbl)
            n216 = Decimal String To Number(string=w859, offset=0 ("offset (0)")) -> (number=w865:i32)  [unwired: 1 in, 1 out]
            n217 = Not Equal?(x=w859, y="") -> (x != y?=w857:bool)
            n218 = property on="X  in Range" class="Bool (strict)"("Val(Sgnl)"=w882) -> ()  [unwired: 2 in, 2 out]
            n219 = property on="X Ready" class="Bool (strict)"("Val(Sgnl)"=w857) -> ()  [unwired: 2 in, 2 out]
            n220 = Divide(x=w875, y=w881) -> (x/y=w879:dbl)
            n221 = Number To Boolean Array(number=w865) -> (Boolean array=w864:bool[])
            n222 = property on="X mm/rev" class="DigNum (strict)"() -> ("Value"=w878:dbl)  [unwired: 2 in, 2 out]
            n223 = Index Array(array=w864, index=0) -> (element=w862:bool)
            n224 = Multiply(x=w879, y=w878) -> (x*y=w877:dbl)
            n225 = property on="X  in Motion" class="Bool (strict)"("Val(Sgnl)"=w862) -> ()  [unwired: 2 in, 2 out]
            n226 = Add(x=w877, y=w876) -> (x+y=w856:dbl)
            n227 = property on="X Position mm PV" class="DigNum (strict)"("Val(Sgnl)"=w856) -> ()  [unwired: 2 in, 2 out]
            n228 = shared-variable "My Computer\\S132PC1_PV.lvlib\\MX"(w856) -> ()  [unwired: 1 in, 1 out]
          }
          frame #1 {
            n229 = property on="X Scan" class="Bool (strict)"() -> ("Value"=w895:bool)  [unwired: 2 in, 2 out]
            n230 = Or(x=w894, y=w895) -> (x .or. y?=w896:bool)
            n231 = case shown="True" w896 {
              frame False {
                n232 = property on="X Go" class="Bool"("DisabledEnum"=T2."Enabled" ("Disabled")) -> ()  [unwired: 2 in, 2 out]
                n233 = property on="X Scan OK" class="Bool"("DisabledEnum"=T2."Enabled" ("Disabled")) -> ()  [unwired: 2 in, 2 out]
              }
              frame True {
                n234 = property on="X Go" class="Bool"("DisabledEnum"=T2."Disabled and Grayed Out" ("Disabled")) -> ()  [unwired: 2 in, 2 out]
                n235 = property on="X Scan OK" class="Bool"("DisabledEnum"=T2."Disabled and Grayed Out" ("Disabled")) -> ()  [unwired: 2 in, 2 out]
              }
            }
          }
          frame #2 {
            n236 = case shown="False" w905 {
              tunnel: w906 -> [w912 w916]
              tunnel: [w913 w916] -> w907
              tunnel: [w914 w915] -> w908
              tunnel: w909 -> [w911 w915]
              frame False {
                n237 = call "mDrive Send Command.vi"("error in (no error)"=w911, "Command"=T1."Stop", "VISA resource name"=w912) -> ("error out"=w914:errorcluster, "VISA resource name out"=w913:refnum<visa-resource-name>)  [unwired: 4 in, 1 out]
              }
              frame True {
              }
            }
          }
          frame #3 {
            n238 = property on="X Backlash corr" class="Bool (strict)"() -> ("Value"=w923:bool)  [unwired: 2 in, 2 out]
            n239 = Implies(1:w922, 2:w923) -> (0:w921:bool)
            n240 = case shown="False" w921 {
              tunnel: w920 -> [w930 w983]
              tunnel: w919 -> [w929 w984]
              tunnel: [w928 w983] -> w918
              tunnel: [w927 w984] -> w917
              frame False {
                # "Backlash"
                n241 = flat-sequence {
                  tunnel: [w945] -> w942
                  tunnel: [w947] -> w941
                  tunnel: [w946] -> w940
                  tunnel: w930 -> [w944]
                  tunnel: w929 -> [w943]
                  tunnel: w942 -> [w955]
                  tunnel: [w955] -> w939
                  tunnel: w941 -> [w954]
                  tunnel: w940 -> [w953]
                  tunnel: [w952] -> w938
                  tunnel: [w951] -> w937
                  tunnel: [w950] -> w926
                  tunnel: w939 -> [w965]
                  tunnel: w938 -> [w964]
                  tunnel: w937 -> [w962]
                  tunnel: [w963] -> w936
                  tunnel: [w962] -> w935
                  tunnel: [w961] -> w932
                  tunnel: [w960] -> w931
                  tunnel: w926 -> [w960]
                  tunnel: w936 -> [w976]
                  tunnel: w935 -> [w969]
                  tunnel: [w976] -> w934
                  tunnel: [w975] -> w933
                  tunnel: w932 -> [w975]
                  tunnel: w931 -> [w971]
                  tunnel: [w970] -> w924
                  tunnel: w934 -> [w980]
                  tunnel: w933 -> [w979]
                  tunnel: [w978] -> w928
                  tunnel: [w977] -> w925
                  tunnel: w924 -> [w977]
                  tunnel: [w982] -> w927
                  tunnel: w925 -> [w982]
                  frame #0 {
                    n242 = property on="X Backlash steps/sec" class="DigNum (strict)"() -> ("Value"=w945:i32)  [unwired: 2 in, 2 out]
                    n243 = Number To Decimal String(number=w945) -> (decimal integer string=w948:string)  [unwired: 1 in]
                    n244 = call "mDrive Send Command.vi"("error in (no error)"=w944, "Extra"=w948, "Command"=T1."Max Velocity", "VISA resource name"=w943) -> ("error out"=w946:errorcluster, "VISA resource name out"=w947:refnum<visa-resource-name>)  [unwired: 3 in, 1 out]
                  }
                  frame #1 {
                    n245 = property on="X Backlash" class="DigNum (strict)"() -> ("Value"=w950:i32)  [unwired: 2 in, 2 out]
                    n246 = Number To Decimal String(number=w950) -> (decimal integer string=w956:string)  [unwired: 1 in]
                    n247 = call "mDrive Send Command.vi"("error in (no error)"=w953, "Extra"=w956, "Command"=T1."Move to Relative Position", "VISA resource name"=w954) -> ("error out"=w952:errorcluster, "VISA resource name out"=w951:refnum<visa-resource-name>)  [unwired: 3 in, 1 out]
                  }
                  frame #2 {
                    n248 = To Double Precision Float(number=w960) -> (double precision float=w958:dbl)
                    n249 = To Double Precision Float(number=w965) -> (double precision float=w967:dbl)
                    n250 = Absolute Value(x=w958) -> (abs(x)=w959:dbl)
                    n251 = Divide(x=w959, y=w967) -> (x/y=w968:dbl)
                    n252 = Add(x=w968, y=0.3) -> (x+y=w961:dbl)
                    n253 = call "Time Delay13"("error in (no error)"=w964, "Delay Time (s)"=w961) -> ("error out"=w963:errorcluster)  [unwired: 9 in]
                  }
                  frame #3 {
                    n254 = Negate(x=w971) -> (-x=w972:i32)
                    n255 = Number To Decimal String(number=w972) -> (decimal integer string=w973:string)  [unwired: 1 in]
                    n256 = call "mDrive Send Command.vi"("Extra"=w973, "Command"=T1."Move to Relative Position", "VISA resource name"=w969) -> ("VISA resource name out"=w970:refnum<visa-resource-name>)  [unwired: 4 in, 2 out]
                  }
                  frame #4 {
                    n257 = call "Time Delay14"("error in (no error)"=w980, "Delay Time (s)"=w979) -> ("error out"=w978:errorcluster)  [unwired: 9 in]
                  }
                  frame #5 {
                    n258 = property on="X Backlash corr" class="Bool (strict)"("Val(Sgnl)"=FALSE ("Value (Signaling)")) -> ()  [unwired: 2 in, 2 out]
                  }
                }
              }
              frame True {
              }
            }
          }
        }
        n259 = flat-sequence {
          tunnel: w594 -> [w1017]
          tunnel: w532 -> [w1016]
          tunnel: [w1022] -> w591
          tunnel: [w998] -> w589
          tunnel: [w1009] -> w587
          tunnel: [w989] -> w585
          tunnel: w591 -> [w1028]
          tunnel: [w1028] -> w590
          tunnel: w589 -> [w1027]
          tunnel: [w1027] -> w588
          tunnel: w587 -> [w1026]
          tunnel: [w1026] -> w586
          tunnel: w585 -> [w1023]
          tunnel: [w1023] -> w581
          tunnel: w590 -> [w1035]
          tunnel: [w1036] -> w584
          tunnel: w588 -> [w1038]
          tunnel: [w1037] -> w583
          tunnel: w586 -> [w1034]
          tunnel: [w1033] -> w582
          tunnel: w581 -> [w1033]
          tunnel: w584 -> [w1048]
          tunnel: w583 -> [w1049]
          tunnel: w582 -> [w1051]
          tunnel: [w1047] -> w593
          tunnel: [w1046] -> w592
          frame #0 {
            w993 = 0.1 ("Delay Time (s)")
            n260 = property on="Y Step SP" class="DigNum (strict)"() -> ("Maximum"=w1011:dbl)  [unwired: 2 in, 2 out]
            n261 = property on="Y Step SP" class="DigNum (strict)"() -> ("Minimum"=w1013:dbl)  [unwired: 2 in, 2 out]
            n262 = property on="Y steps/rev" class="DigNum (strict)"() -> ("Value"=w1007:u32)  [unwired: 2 in, 2 out]
            n263 = property on="Y offset mm" class="DigNum (strict)"() -> ("Value"=w1003:dbl)  [unwired: 2 in, 2 out]
            n264 = To Long Integer(number=w1011) -> (32bit integer=w1010:i32)
            n265 = To Long Integer(number=w1013) -> (32bit integer=w1012:i32)
            n266 = To Double Precision Float(number=w1007) -> (double precision float=w1008:dbl)
            n267 = call "mDrive Send Command.vi"("error in (no error)"=w1017, "Extra"="P", "Command"=T1."Print Parameter", "VISA resource name"=w1016) -> ("error out"=w1015:errorcluster, "read buffer"=w1021:string, "VISA resource name out"=w1019:refnum<visa-resource-name>)  [unwired: 3 in]
            n268 = call "Time Delay4"("error in (no error)"=w1015, "Delay Time (s)"=w993) -> ("error out"=w1014:errorcluster)  [unwired: 9 in]
            n269 = Decimal String To Number(string=w1021, offset=0) -> (number=w1000:i32)  [unwired: 1 in, 1 out]
            n270 = To Long Integer(number=w1000) -> (32bit integer=w1001:i32)
            n271 = property on="Y Step PV" class="DigNum (strict)"("Val(Sgnl)"=w1001) -> ()  [unwired: 2 in, 2 out]
            n272 = call "mDrive Send Command.vi"("error in (no error)"=w1014, "Extra"="MV", "Command"=T1."Print Parameter", "VISA resource name"=w1019) -> ("error out"=w1018:errorcluster, "read buffer"=w986:string, "VISA resource name out"=w1022:refnum<visa-resource-name>)  [unwired: 3 in]
            n273 = call "Time Delay3"("error in (no error)"=w1018, "Delay Time (s)"=w993) -> ("error out"=w998:errorcluster)  [unwired: 9 in]
            n274 = In Range and Coerce(upper limit=w1010, x=w1001, lower limit=w1012) -> (In Range?=w1009:bool)  [unwired: 1 out]
            n275 = To Double Precision Float(number=w1001) -> (double precision float=w1002:dbl)
            n276 = Decimal String To Number(string=w986, offset=0 ("offset (0)")) -> (number=w992:i32)  [unwired: 1 in, 1 out]
            n277 = Not Equal?(x=w986, y="") -> (x != y?=w987:bool)
            n278 = property on="Y in Range" class="Bool (strict)"("Val(Sgnl)"=w1009) -> ()  [unwired: 2 in, 2 out]
            n279 = property on="Y Ready" class="Bool (strict)"("Val(Sgnl)"=w987) -> ()  [unwired: 2 in, 2 out]
            n280 = Divide(x=w1002, y=w1008) -> (x/y=w1006:dbl)
            n281 = Number To Boolean Array(number=w992) -> (Boolean array=w991:bool[])
            n282 = property on="Y mm/rev" class="DigNum (strict)"() -> ("Value"=w1005:dbl)  [unwired: 2 in, 2 out]
            n283 = Index Array(array=w991, index=0) -> (element=w989:bool)
            n284 = Multiply(x=w1006, y=w1005) -> (x*y=w1004:dbl)
            n285 = property on="Y in Motion" class="Bool (strict)"("Val(Sgnl)"=w989) -> ()  [unwired: 2 in, 2 out]
            n286 = Add(x=w1004, y=w1003) -> (x+y=w985:dbl)
            n287 = property on="Y Position mm PV" class="DigNum (strict)"("Val(Sgnl)"=w985) -> ()  [unwired: 2 in, 2 out]
            n288 = shared-variable "My Computer\\S132PC1_PV.lvlib\\MY"(w985) -> ()  [unwired: 1 in, 1 out]
          }
          frame #1 {
            n289 = property on="Y Scan" class="Bool (strict)"() -> ("Value"=w1024:bool)  [unwired: 2 in, 2 out]
            n290 = Or(x=w1023, y=w1024) -> (x .or. y?=w1025:bool)
            n291 = case shown="True" w1025 {
              frame False {
                n292 = property on="Y Go" class="Bool"("DisabledEnum"=T2."Enabled" ("Disabled")) -> ()  [unwired: 2 in, 2 out]
                n293 = property on="Y Scan OK" class="Bool"("DisabledEnum"=T2."Enabled" ("Disabled")) -> ()  [unwired: 2 in, 2 out]
              }
              frame True {
                n294 = property on="Y Go" class="Bool"("DisabledEnum"=T2."Disabled and Grayed Out" ("Disabled")) -> ()  [unwired: 2 in, 2 out]
                n295 = property on="Y Scan OK" class="Bool"("DisabledEnum"=T2."Disabled and Grayed Out" ("Disabled")) -> ()  [unwired: 2 in, 2 out]
              }
            }
          }
          frame #2 {
            n296 = case shown="False" w1034 {
              tunnel: w1035 -> [w1041 w1045]
              tunnel: [w1042 w1045] -> w1036
              tunnel: [w1043 w1044] -> w1037
              tunnel: w1038 -> [w1040 w1044]
              frame False {
                n297 = call "mDrive Send Command.vi"("error in (no error)"=w1040, "Command"=T1."Stop", "VISA resource name"=w1041) -> ("error out"=w1043:errorcluster, "VISA resource name out"=w1042:refnum<visa-resource-name>)  [unwired: 4 in, 1 out]
              }
              frame True {
              }
            }
          }
          frame #3 {
            n298 = property on="Y Backlash corr" class="Bool (strict)"() -> ("Value"=w1052:bool)  [unwired: 2 in, 2 out]
            n299 = Implies(1:w1051, 2:w1052) -> (0:w1050:bool)
            n300 = case shown="False" w1050 {
              tunnel: w1049 -> [w1059 w1112]
              tunnel: w1048 -> [w1058 w1113]
              tunnel: [w1057 w1112] -> w1047
              tunnel: [w1056 w1113] -> w1046
              frame False {
                # "Backlash"
                n301 = flat-sequence {
                  tunnel: [w1074] -> w1071
                  tunnel: [w1076] -> w1070
                  tunnel: [w1075] -> w1069
                  tunnel: w1059 -> [w1073]
                  tunnel: w1058 -> [w1072]
                  tunnel: w1071 -> [w1084]
                  tunnel: [w1084] -> w1068
                  tunnel: w1070 -> [w1083]
                  tunnel: w1069 -> [w1082]
                  tunnel: [w1081] -> w1067
                  tunnel: [w1080] -> w1066
                  tunnel: [w1079] -> w1055
                  tunnel: w1068 -> [w1094]
                  tunnel: w1067 -> [w1093]
                  tunnel: w1066 -> [w1091]
                  tunnel: [w1092] -> w1065
                  tunnel: [w1091] -> w1064
                  tunnel: [w1090] -> w1061
                  tunnel: [w1089] -> w1060
                  tunnel: w1055 -> [w1089]
                  tunnel: w1065 -> [w1105]
                  tunnel: w1064 -> [w1098]
                  tunnel: [w1105] -> w1063
                  tunnel: [w1104] -> w1062
                  tunnel: w1061 -> [w1104]
                  tunnel: w1060 -> [w1100]
                  tunnel: [w1099] -> w1053
                  tunnel: w1063 -> [w1109]
                  tunnel: w1062 -> [w1108]
                  tunnel: [w1107] -> w1057
                  tunnel: [w1106] -> w1054
                  tunnel: w1053 -> [w1106]
                  tunnel: [w1111] -> w1056
                  tunnel: w1054 -> [w1111]
                  frame #0 {
                    n302 = property on="Y Backlash steps/sec" class="DigNum (strict)"() -> ("Value"=w1074:i32)  [unwired: 2 in, 2 out]
                    n303 = Number To Decimal String(number=w1074) -> (decimal integer string=w1077:string)  [unwired: 1 in]
                    n304 = call "mDrive Send Command.vi"("error in (no error)"=w1073, "Extra"=w1077, "Command"=T1."Max Velocity", "VISA resource name"=w1072) -> ("error out"=w1075:errorcluster, "VISA resource name out"=w1076:refnum<visa-resource-name>)  [unwired: 3 in, 1 out]
                  }
                  frame #1 {
                    n305 = property on="Y Backlash" class="DigNum (strict)"() -> ("Value"=w1079:i32)  [unwired: 2 in, 2 out]
                    n306 = Number To Decimal String(number=w1079) -> (decimal integer string=w1085:string)  [unwired: 1 in]
                    n307 = call "mDrive Send Command.vi"("error in (no error)"=w1082, "Extra"=w1085, "Command"=T1."Move to Relative Position", "VISA resource name"=w1083) -> ("error out"=w1081:errorcluster, "VISA resource name out"=w1080:refnum<visa-resource-name>)  [unwired: 3 in, 1 out]
                  }
                  frame #2 {
                    n308 = To Double Precision Float(number=w1089) -> (double precision float=w1087:dbl)
                    n309 = To Double Precision Float(number=w1094) -> (double precision float=w1096:dbl)
                    n310 = Absolute Value(x=w1087) -> (abs(x)=w1088:dbl)
                    n311 = Divide(x=w1088, y=w1096) -> (x/y=w1097:dbl)
                    n312 = Add(x=w1097, y=0.3) -> (x+y=w1090:dbl)
                    n313 = call "Time Delay8"("error in (no error)"=w1093, "Delay Time (s)"=w1090) -> ("error out"=w1092:errorcluster)  [unwired: 9 in]
                  }
                  frame #3 {
                    n314 = Negate(x=w1100) -> (-x=w1101:i32)
                    n315 = Number To Decimal String(number=w1101) -> (decimal integer string=w1102:string)  [unwired: 1 in]
                    n316 = call "mDrive Send Command.vi"("Extra"=w1102, "Command"=T1."Move to Relative Position", "VISA resource name"=w1098) -> ("VISA resource name out"=w1099:refnum<visa-resource-name>)  [unwired: 4 in, 2 out]
                  }
                  frame #4 {
                    n317 = call "Time Delay2"("error in (no error)"=w1109, "Delay Time (s)"=w1108) -> ("error out"=w1107:errorcluster)  [unwired: 9 in]
                  }
                  frame #5 {
                    n318 = property on="Y Backlash corr" class="Bool (strict)"("Val(Sgnl)"=FALSE ("Value (Signaling)")) -> ()  [unwired: 2 in, 2 out]
                  }
                }
              }
              frame True {
              }
            }
          }
        }
        n319 = flat-sequence {
          tunnel: [w764] -> w566
          tunnel: [w743] -> w565
          tunnel: [w754] -> w564
          tunnel: [w734] -> w563
          tunnel: w541 -> [w733]
          tunnel: w544 -> [w732]
          tunnel: w566 -> [w770]
          tunnel: [w770] -> w562
          tunnel: w565 -> [w769]
          tunnel: [w769] -> w561
          tunnel: w564 -> [w768]
          tunnel: [w768] -> w560
          tunnel: w563 -> [w765]
          tunnel: [w765] -> w559
          tunnel: w562 -> [w777]
          tunnel: [w778] -> w558
          tunnel: w561 -> [w780]
          tunnel: [w779] -> w557
          tunnel: w560 -> [w776]
          tunnel: [w775] -> w556
          tunnel: w559 -> [w775]
          tunnel: w558 -> [w790]
          tunnel: w557 -> [w791]
          tunnel: w556 -> [w793]
          tunnel: [w789] -> w542
          tunnel: [w788] -> w543
          frame #0 {
            w738 = 0.1 ("Delay Time (s)")
            n320 = property on="Z max step" class="DigNum (strict)"() -> ("Value"=w728:i32)  [unwired: 2 in, 2 out]
            n321 = property on="Z Step SP" class="DigNum (strict)" props=["Maximum"]() -> ()  [unwired: 2 in, 3 out]
            n322 = property on="Z Step SP" class="DigNum (strict)"() -> ("Minimum"=w757:dbl)  [unwired: 2 in, 2 out]
            n323 = property on="Z steps/rev" class="DigNum (strict)"() -> ("Value"=w752:u32)  [unwired: 2 in, 2 out]
            n324 = property on="Z offset mm" class="DigNum (strict)"() -> ("Value"=w748:dbl)  [unwired: 2 in, 2 out]
            n325 = To Long Integer(number=w728) -> (32bit integer=w755:i32)
            n326 = To Long Integer(number=w757) -> (32bit integer=w756:i32)
            n327 = To Double Precision Float(number=w752) -> (double precision float=w753:dbl)
            n328 = call "mDrive Send Command.vi"("error in (no error)"=w732, "Extra"="P", "Command"=T1."Print Parameter", "VISA resource name"=w733) -> ("error out"=w759:errorcluster, "read buffer"=w763:string, "VISA resource name out"=w761:refnum<visa-resource-name>)  [unwired: 3 in]
            n329 = call "Time Delay17"("error in (no error)"=w759, "Delay Time (s)"=w738) -> ("error out"=w758:errorcluster)  [unwired: 9 in]
            n330 = Decimal String To Number(string=w763, offset=0) -> (number=w745:i32)  [unwired: 1 in, 1 out]
            n331 = To Long Integer(number=w745) -> (32bit integer=w746:i32)
            n332 = property on="Z Step PV" class="DigNum (strict)"("Val(Sgnl)"=w746) -> ()  [unwired: 2 in, 2 out]
            n333 = call "mDrive Send Command.vi"("error in (no error)"=w758, "Extra"="MV", "Command"=T1."Print Parameter", "VISA resource name"=w761) -> ("error out"=w760:errorcluster, "read buffer"=w729:string, "VISA resource name out"=w764:refnum<visa-resource-name>)  [unwired: 3 in]
            n334 = call "Time Delay16"("error in (no error)"=w760, "Delay Time (s)"=w738) -> ("error out"=w743:errorcluster)  [unwired: 9 in]
            n335 = In Range and Coerce(upper limit=w755, x=w746, lower limit=w756) -> (In Range?=w754:bool)  [unwired: 1 out]
            n336 = To Double Precision Float(number=w746) -> (double precision float=w747:dbl)
            n337 = Decimal String To Number(string=w729, offset=0 ("offset (0)")) -> (number=w737:i32)  [unwired: 1 in, 1 out]
            n338 = Not Equal?(x=w729, y="") -> (x != y?=w730:bool)
            n339 = property on="Z in Range" class="Bool (strict)"("Val(Sgnl)"=w754) -> ()  [unwired: 2 in, 2 out]
            n340 = property on="Z Ready" class="Bool (strict)"("Val(Sgnl)"=w730) -> ()  [unwired: 2 in, 2 out]
            n341 = Divide(x=w747, y=w753) -> (x/y=w751:dbl)
            n342 = Number To Boolean Array(number=w737) -> (Boolean array=w736:bool[])
            n343 = property on="Z mm/rev" class="DigNum (strict)"() -> ("Value"=w750:dbl)  [unwired: 2 in, 2 out]
            n344 = Index Array(array=w736, index=0) -> (element=w734:bool)
            n345 = Multiply(x=w751, y=w750) -> (x*y=w749:dbl)
            n346 = property on="Z in Motion" class="Bool (strict)"("Val(Sgnl)"=w734) -> ()  [unwired: 2 in, 2 out]
            n347 = Add(x=w749, y=w748) -> (x+y=w727:dbl)
            n348 = shared-variable "My Computer\\S132PC1_PV.lvlib\\MZ"(w727) -> ()  [unwired: 1 in, 1 out]
            n349 = property on="Z Position mm PV" class="DigNum (strict)"("Val(Sgnl)"=w727) -> ()  [unwired: 2 in, 2 out]
          }
          frame #1 {
            n350 = property on="Z Scan" class="Bool (strict)"() -> ("Value"=w766:bool)  [unwired: 2 in, 2 out]
            n351 = Or(x=w765, y=w766) -> (x .or. y?=w767:bool)
            n352 = case shown="True" w767 {
              frame False {
                n353 = property on="Z Go" class="Bool"("DisabledEnum"=T2."Enabled" ("Disabled")) -> ()  [unwired: 2 in, 2 out]
                n354 = property on="Z Scan OK" class="Bool"("DisabledEnum"=T2."Enabled" ("Disabled")) -> ()  [unwired: 2 in, 2 out]
              }
              frame True {
                n355 = property on="Z Go" class="Bool"("DisabledEnum"=T2."Disabled and Grayed Out" ("Disabled")) -> ()  [unwired: 2 in, 2 out]
                n356 = property on="Z Scan OK" class="Bool"("DisabledEnum"=T2."Disabled and Grayed Out" ("Disabled")) -> ()  [unwired: 2 in, 2 out]
              }
            }
          }
          frame #2 {
            n357 = case shown="False" w776 {
              tunnel: w777 -> [w783 w787]
              tunnel: [w784 w787] -> w778
              tunnel: [w785 w786] -> w779
              tunnel: w780 -> [w782 w786]
              frame False {
                n358 = call "mDrive Send Command.vi"("error in (no error)"=w782, "Command"=T1."Stop", "VISA resource name"=w783) -> ("error out"=w785:errorcluster, "VISA resource name out"=w784:refnum<visa-resource-name>)  [unwired: 4 in, 1 out]
              }
              frame True {
              }
            }
          }
          frame #3 {
            n359 = property on="Z Backlash corr" class="Bool (strict)"() -> ("Value"=w794:bool)  [unwired: 2 in, 2 out]
            n360 = Implies(1:w793, 2:w794) -> (0:w792:bool)
            n361 = case shown="False" w792 {
              tunnel: w791 -> [w801 w854]
              tunnel: w790 -> [w800 w855]
              tunnel: [w799 w854] -> w789
              tunnel: [w798 w855] -> w788
              frame False {
                # "Backlash"
                n362 = flat-sequence {
                  tunnel: [w816] -> w813
                  tunnel: [w818] -> w812
                  tunnel: [w817] -> w811
                  tunnel: w801 -> [w815]
                  tunnel: w800 -> [w814]
                  tunnel: w813 -> [w826]
                  tunnel: [w826] -> w810
                  tunnel: w812 -> [w825]
                  tunnel: w811 -> [w824]
                  tunnel: [w823] -> w809
                  tunnel: [w822] -> w808
                  tunnel: [w821] -> w797
                  tunnel: w810 -> [w836]
                  tunnel: w809 -> [w835]
                  tunnel: w808 -> [w833]
                  tunnel: [w834] -> w807
                  tunnel: [w833] -> w806
                  tunnel: [w832] -> w803
                  tunnel: [w831] -> w802
                  tunnel: w797 -> [w831]
                  tunnel: w807 -> [w847]
                  tunnel: w806 -> [w840]
                  tunnel: [w847] -> w805
                  tunnel: [w846] -> w804
                  tunnel: w803 -> [w846]
                  tunnel: w802 -> [w842]
                  tunnel: [w841] -> w795
                  tunnel: w805 -> [w851]
                  tunnel: w804 -> [w850]
                  tunnel: [w849] -> w799
                  tunnel: [w848] -> w796
                  tunnel: w795 -> [w848]
                  tunnel: [w853] -> w798
                  tunnel: w796 -> [w853]
                  frame #0 {
                    n363 = property on="Z Backlash steps/sec" class="DigNum (strict)"() -> ("Value"=w816:i32)  [unwired: 2 in, 2 out]
                    n364 = Number To Decimal String(number=w816) -> (decimal integer string=w819:string)  [unwired: 1 in]
                    n365 = call "mDrive Send Command.vi"("error in (no error)"=w815, "Extra"=w819, "Command"=T1."Max Velocity", "VISA resource name"=w814) -> ("error out"=w817:errorcluster, "VISA resource name out"=w818:refnum<visa-resource-name>)  [unwired: 3 in, 1 out]
                  }
                  frame #1 {
                    n366 = property on="Z Backlash" class="DigNum (strict)"() -> ("Value"=w821:i32)  [unwired: 2 in, 2 out]
                    n367 = Number To Decimal String(number=w821) -> (decimal integer string=w827:string)  [unwired: 1 in]
                    n368 = call "mDrive Send Command.vi"("error in (no error)"=w824, "Extra"=w827, "Command"=T1."Move to Relative Position", "VISA resource name"=w825) -> ("error out"=w823:errorcluster, "VISA resource name out"=w822:refnum<visa-resource-name>)  [unwired: 3 in, 1 out]
                  }
                  frame #2 {
                    n369 = To Double Precision Float(number=w831) -> (double precision float=w829:dbl)
                    n370 = To Double Precision Float(number=w836) -> (double precision float=w838:dbl)
                    n371 = Absolute Value(x=w829) -> (abs(x)=w830:dbl)
                    n372 = Divide(x=w830, y=w838) -> (x/y=w839:dbl)
                    n373 = Add(x=w839, y=0.5) -> (x+y=w832:dbl)
                    n374 = call "Time Delay18"("error in (no error)"=w835, "Delay Time (s)"=w832) -> ("error out"=w834:errorcluster)  [unwired: 9 in]
                  }
                  frame #3 {
                    n375 = Negate(x=w842) -> (-x=w843:i32)
                    n376 = Number To Decimal String(number=w843) -> (decimal integer string=w844:string)  [unwired: 1 in]
                    n377 = call "mDrive Send Command.vi"("Extra"=w844, "Command"=T1."Move to Relative Position", "VISA resource name"=w840) -> ("VISA resource name out"=w841:refnum<visa-resource-name>)  [unwired: 4 in, 2 out]
                  }
                  frame #4 {
                    n378 = call "Time Delay19"("error in (no error)"=w851, "Delay Time (s)"=w850) -> ("error out"=w849:errorcluster)  [unwired: 9 in]
                  }
                  frame #5 {
                    n379 = property on="Z Backlash corr" class="Bool (strict)"("Val(Sgnl)"=FALSE ("Value (Signaling)")) -> ()  [unwired: 2 in, 2 out]
                  }
                }
              }
              frame True {
              }
            }
          }
        }
        n380 = flat-sequence {
          tunnel: [w635] -> w555
          tunnel: [w613] -> w554
          tunnel: [w624] -> w553
          tunnel: [w604] -> w552
          tunnel: w540 -> [w603]
          tunnel: w539 -> [w602]
          tunnel: w555 -> [w641]
          tunnel: [w641] -> w551
          tunnel: w554 -> [w640]
          tunnel: [w640] -> w550
          tunnel: w553 -> [w639]
          tunnel: [w639] -> w549
          tunnel: w552 -> [w636]
          tunnel: [w636] -> w548
          tunnel: w551 -> [w648]
          tunnel: [w649] -> w547
          tunnel: w550 -> [w651]
          tunnel: [w650] -> w546
          tunnel: w549 -> [w647]
          tunnel: [w646] -> w545
          tunnel: w548 -> [w646]
          tunnel: w547 -> [w661]
          tunnel: w546 -> [w662]
          tunnel: w545 -> [w664]
          tunnel: [w660] -> w537
          tunnel: [w659] -> w538
          frame #0 {
            w608 = 0.1 ("Delay Time (s)")
            n381 = property on="R Step SP" class="DigNum (strict)"() -> ("Maximum"=w626:dbl)  [unwired: 2 in, 2 out]
            n382 = property on="R Step SP" class="DigNum (strict)"() -> ("Minimum"=w628:dbl)  [unwired: 2 in, 2 out]
            n383 = property on="R steps/rev" class="DigNum (strict)"() -> ("Value"=w622:u32)  [unwired: 2 in, 2 out]
            n384 = property on="R offset deg" class="DigNum (strict)"() -> ("Value"=w618:dbl)  [unwired: 2 in, 2 out]
            n385 = To Long Integer(number=w626) -> (32bit integer=w625:i32)
            n386 = To Long Integer(number=w628) -> (32bit integer=w627:i32)
            n387 = To Double Precision Float(number=w622) -> (double precision float=w623:dbl)
            n388 = call "mDrive Send Command.vi"("error in (no error)"=w602, "Extra"="P", "Command"=T1."Print Parameter", "VISA resource name"=w603) -> ("error out"=w630:errorcluster, "read buffer"=w634:string, "VISA resource name out"=w632:refnum<visa-resource-name>)  [unwired: 3 in]
            n389 = call "Time Delay21"("error in (no error)"=w630, "Delay Time (s)"=w608) -> ("error out"=w629:errorcluster)  [unwired: 9 in]
            n390 = Decimal String To Number(string=w634, offset=0) -> (number=w615:i32)  [unwired: 1 in, 1 out]
            n391 = To Long Integer(number=w615) -> (32bit integer=w616:i32)
            n392 = property on="R Step PV" class="DigNum (strict)"("Val(Sgnl)"=w616) -> ()  [unwired: 2 in, 2 out]
            n393 = call "mDrive Send Command.vi"("error in (no error)"=w629, "Extra"="MV", "Command"=T1."Print Parameter", "VISA resource name"=w632) -> ("error out"=w631:errorcluster, "read buffer"=w599:string, "VISA resource name out"=w635:refnum<visa-resource-name>)  [unwired: 3 in]
            n394 = call "Time Delay20"("error in (no error)"=w631, "Delay Time (s)"=w608) -> ("error out"=w613:errorcluster)  [unwired: 9 in]
            n395 = In Range and Coerce(upper limit=w625, x=w616, lower limit=w627) -> (In Range?=w624:bool)  [unwired: 1 out]
            n396 = To Double Precision Float(number=w616) -> (double precision float=w617:dbl)
            n397 = Decimal String To Number(string=w599, offset=0 ("offset (0)")) -> (number=w607:i32)  [unwired: 1 in, 1 out]
            n398 = Not Equal?(x=w599, y="") -> (x != y?=w600:bool)
            n399 = property on="R in Range" class="Bool (strict)"("Val(Sgnl)"=w624) -> ()  [unwired: 2 in, 2 out]
            n400 = property on="R Ready" class="Bool (strict)"("Val(Sgnl)"=w600) -> ()  [unwired: 2 in, 2 out]
            n401 = Divide(x=w617, y=w623) -> (x/y=w621:dbl)
            n402 = Number To Boolean Array(number=w607) -> (Boolean array=w606:bool[])
            n403 = property on="R deg/rev" class="DigNum (strict)"() -> ("Value"=w620:dbl)  [unwired: 2 in, 2 out]
            n404 = Index Array(array=w606, index=0) -> (element=w604:bool)
            n405 = Multiply(x=w621, y=w620) -> (x*y=w619:dbl)
            n406 = property on="R in Motion" class="Bool (strict)"("Val(Sgnl)"=w604) -> ()  [unwired: 2 in, 2 out]
            n407 = Add(x=w619, y=w618) -> (x+y=w598:dbl)
            n408 = property on="R Position deg PV" class="DigNum (strict)"("Val(Sgnl)"=w598) -> ()  [unwired: 2 in, 2 out]
            n409 = shared-variable "My Computer\\S132PC1_PV.lvlib\\MR"(w598) -> ()  [unwired: 1 in, 1 out]
          }
          frame #1 {
            n410 = property on="R Scan" class="Bool (strict)"() -> ("Value"=w637:bool)  [unwired: 2 in, 2 out]
            n411 = Or(x=w636, y=w637) -> (x .or. y?=w638:bool)
            n412 = case shown="True" w638 {
              frame False {
                n413 = property on="R Go" class="Bool"("DisabledEnum"=T2."Enabled" ("Disabled")) -> ()  [unwired: 2 in, 2 out]
                n414 = property on="R Scan OK" class="Bool"("DisabledEnum"=T2."Enabled" ("Disabled")) -> ()  [unwired: 2 in, 2 out]
              }
              frame True {
                n415 = property on="R Go" class="Bool"("DisabledEnum"=T2."Disabled and Grayed Out" ("Disabled")) -> ()  [unwired: 2 in, 2 out]
                n416 = property on="R Scan OK" class="Bool"("DisabledEnum"=T2."Disabled and Grayed Out" ("Disabled")) -> ()  [unwired: 2 in, 2 out]
              }
            }
          }
          frame #2 {
            n417 = case shown="False" w647 {
              tunnel: w648 -> [w654 w658]
              tunnel: [w655 w658] -> w649
              tunnel: [w656 w657] -> w650
              tunnel: w651 -> [w653 w657]
              frame False {
                n418 = call "mDrive Send Command.vi"("error in (no error)"=w653, "Command"=T1."Stop", "VISA resource name"=w654) -> ("error out"=w656:errorcluster, "VISA resource name out"=w655:refnum<visa-resource-name>)  [unwired: 4 in, 1 out]
              }
              frame True {
              }
            }
          }
          frame #3 {
            n419 = property on="R Backlash corr" class="Bool (strict)"() -> ("Value"=w665:bool)  [unwired: 2 in, 2 out]
            n420 = Implies(1:w664, 2:w665) -> (0:w663:bool)
            n421 = case shown="False" w663 {
              tunnel: w662 -> [w672 w725]
              tunnel: w661 -> [w671 w726]
              tunnel: [w670 w725] -> w660
              tunnel: [w669 w726] -> w659
              frame False {
                # "Backlash"
                n422 = flat-sequence {
                  tunnel: [w687] -> w684
                  tunnel: [w689] -> w683
                  tunnel: [w688] -> w682
                  tunnel: w672 -> [w686]
                  tunnel: w671 -> [w685]
                  tunnel: w684 -> [w697]
                  tunnel: [w697] -> w681
                  tunnel: w683 -> [w696]
                  tunnel: w682 -> [w695]
                  tunnel: [w694] -> w680
                  tunnel: [w693] -> w679
                  tunnel: [w692] -> w668
                  tunnel: w681 -> [w707]
                  tunnel: w680 -> [w706]
                  tunnel: w679 -> [w704]
                  tunnel: [w705] -> w678
                  tunnel: [w704] -> w677
                  tunnel: [w703] -> w674
                  tunnel: [w702] -> w673
                  tunnel: w668 -> [w702]
                  tunnel: w678 -> [w718]
                  tunnel: w677 -> [w711]
                  tunnel: [w718] -> w676
                  tunnel: [w717] -> w675
                  tunnel: w674 -> [w717]
                  tunnel: w673 -> [w713]
                  tunnel: [w712] -> w666
                  tunnel: w676 -> [w722]
                  tunnel: w675 -> [w721]
                  tunnel: [w720] -> w670
                  tunnel: [w719] -> w667
                  tunnel: w666 -> [w719]
                  tunnel: [w724] -> w669
                  tunnel: w667 -> [w724]
                  frame #0 {
                    n423 = property on="R Backlash steps/sec" class="DigNum (strict)"() -> ("Value"=w687:i32)  [unwired: 2 in, 2 out]
                    n424 = Number To Decimal String(number=w687) -> (decimal integer string=w690:string)  [unwired: 1 in]
                    n425 = call "mDrive Send Command.vi"("error in (no error)"=w686, "Extra"=w690, "Command"=T1."Max Velocity", "VISA resource name"=w685) -> ("error out"=w688:errorcluster, "VISA resource name out"=w689:refnum<visa-resource-name>)  [unwired: 3 in, 1 out]
                  }
                  frame #1 {
                    n426 = property on="R Backlash" class="DigNum (strict)"() -> ("Value"=w692:i32)  [unwired: 2 in, 2 out]
                    n427 = Number To Decimal String(number=w692) -> (decimal integer string=w698:string)  [unwired: 1 in]
                    n428 = call "mDrive Send Command.vi"("error in (no error)"=w695, "Extra"=w698, "Command"=T1."Move to Relative Position", "VISA resource name"=w696) -> ("error out"=w694:errorcluster, "VISA resource name out"=w693:refnum<visa-resource-name>)  [unwired: 3 in, 1 out]
                  }
                  frame #2 {
                    n429 = To Double Precision Float(number=w702) -> (double precision float=w700:dbl)
                    n430 = To Double Precision Float(number=w707) -> (double precision float=w709:dbl)
                    n431 = Absolute Value(x=w700) -> (abs(x)=w701:dbl)
                    n432 = Divide(x=w701, y=w709) -> (x/y=w710:dbl)
                    n433 = Add(x=w710, y=0.3) -> (x+y=w703:dbl)
                    n434 = call "Time Delay22"("error in (no error)"=w706, "Delay Time (s)"=w703) -> ("error out"=w705:errorcluster)  [unwired: 9 in]
                  }
                  frame #3 {
                    n435 = Negate(x=w713) -> (-x=w714:i32)
                    n436 = Number To Decimal String(number=w714) -> (decimal integer string=w715:string)  [unwired: 1 in]
                    n437 = call "mDrive Send Command.vi"("Extra"=w715, "Command"=T1."Move to Relative Position", "VISA resource name"=w711) -> ("VISA resource name out"=w712:refnum<visa-resource-name>)  [unwired: 4 in, 2 out]
                  }
                  frame #4 {
                    n438 = call "Time Delay23"("error in (no error)"=w722, "Delay Time (s)"=w721) -> ("error out"=w720:errorcluster)  [unwired: 9 in]
                  }
                  frame #5 {
                    n439 = property on="R Backlash corr" class="Bool (strict)"("Val(Sgnl)"=FALSE ("Value (Signaling)")) -> ()  [unwired: 2 in, 2 out]
                  }
                }
              }
              frame True {
              }
            }
          }
        }
        n440 = disable-structure shown="Disabled" {
          frame Disabled {
            n441 = case shown="False" {
              selector: _ -> [_ _]
              tunnel: [w596 w597] -> w595
              frame False {
                n442 = property on="V5 position 15360000" class="DigNum (strict)"() -> ("Value"=w596:i32)  [unwired: 2 in, 2 out]
              }
              frame True {
                n443 = property on="Z Step SP" class="DigNum (strict)"() -> ("Maximum"=w597:dbl)  [unwired: 2 in, 2 out]
              }
            }
            "Z max step" <- w595
          }
          frame Enabled {
          }
        }
        n444 = property on="X Position mm PV" class="DigNum (strict)"() -> ("Value"=w533:dbl)  [unwired: 2 in, 2 out]
        n445 = property on="Y Position mm PV" class="DigNum (strict)"() -> ("Value"=w526:dbl)  [unwired: 2 in, 2 out]
        n446 = property on="Z Position mm PV" class="DigNum (strict)"() -> ("Value"=w527:dbl)  [unwired: 2 in, 2 out]
        n447 = property on="R Position deg PV" class="DigNum (strict)"() -> ("Value"=w534:dbl)  [unwired: 2 in, 2 out]
        n448 = property on="Y Scan Length SP steps" class="DigNum (strict)"() -> ("Value"=w518:i32)  [unwired: 2 in, 2 out]
        n449 = property on="Z Scan Length SP steps" class="DigNum (strict)"() -> ("Value"=w519:i32)  [unwired: 2 in, 2 out]
        n450 = Divide(x=w518, y=w519) -> (x/y=w520:dbl)
        n451 = call "Build XY Graph"("Reset"=TRUE, "Y Input"=w526, "X Input"=w533) -> ("XY Graph"=→"XY Graph":cluster{"Y":dbl[], "Y":dbl[]}[])  [unwired: 7 in, 1 out]
        n452 = call "Build XY Graph2"("Reset"=TRUE, "Y Input"=w534, "X Input"=w527) -> ("XY Graph"=→"ZR Graph":cluster{"Y":dbl[], "Y":dbl[]}[])  [unwired: 7 in, 1 out]
        n453 = property on="Clear ZY" class="Bool (strict)"() -> ("Value"=w517:bool)  [unwired: 2 in, 2 out]
        n454 = call "Build XY Graph3"("Reset"=w517, "Y Input"=w526, "X Input"=w527) -> ("XY Graph"=→"ZY Graph":cluster{"Y":dbl[], "Y":dbl[]}[])  [unwired: 7 in, 1 out]
        n455 = Inverse Tangent(1:w520) -> (0:w521:dbl)
        n456 = Divide(x=w521, y=6.283185307179586) -> (x/y=w522:dbl)
        n457 = Multiply(x=360.0, y=w522) -> (x*y=w525:dbl)
        n458 = property on="atan Y/Z" class="DigNum (strict)"("Val(Sgnl)"=w525) -> ()  [unwired: 2 in, 2 out]
      }
      event "Reset Y Position mm", "Reset X Position mm", "Reset Z Position mm", "Reset R Position deg": Value Change {
        n459 = event-data() -> ()  [unwired: 1 in, 5 out]
        n460 = property on="Z steps/rev" class="DigNum (strict)"() -> ("Value"=w1125:u32)  [unwired: 2 in, 2 out]
        n461 = property on="R steps/rev" class="DigNum (strict)"() -> ("Value"=w1116:u32)  [unwired: 2 in, 2 out]
        n462 = property on="X steps/rev" class="DigNum (strict)"() -> ("Value"=w1134:u32)  [unwired: 2 in, 2 out]
        n463 = property on="Y steps/rev" class="DigNum (strict)"() -> ("Value"=w1143:u32)  [unwired: 2 in, 2 out]
        n464 = property on="Z offset mm" class="DigNum (strict)"() -> ("Value"=w1123:dbl)  [unwired: 2 in, 2 out]
        n465 = property on="R offset deg" class="DigNum (strict)"() -> ("Value"=w1114:dbl)  [unwired: 2 in, 2 out]
        n466 = property on="X offset mm" class="DigNum (strict)"() -> ("Value"=w1132:dbl)  [unwired: 2 in, 2 out]
        n467 = property on="Y offset mm" class="DigNum (strict)"() -> ("Value"=w1141:dbl)  [unwired: 2 in, 2 out]
        n468 = property on="Reset R Position deg" class="DigNum (strict)"() -> ("Value"=w1122:dbl)  [unwired: 2 in, 2 out]
        n469 = property on="Reset Z Position mm" class="DigNum (strict)"() -> ("Value"=w1131:dbl)  [unwired: 2 in, 2 out]
        n470 = property on="Reset X Position mm" class="DigNum (strict)"() -> ("Value"=w1140:dbl)  [unwired: 2 in, 2 out]
        n471 = property on="Reset Y Position mm" class="DigNum (strict)"() -> ("Value"=w1149:dbl)  [unwired: 2 in, 2 out]
        n472 = To Double Precision Float(number=w1116) -> (double precision float=w1119:dbl)
        n473 = To Double Precision Float(number=w1134) -> (double precision float=w1137:dbl)
        n474 = To Double Precision Float(number=w1143) -> (double precision float=w1146:dbl)
        n475 = Subtract(x=w1131, y=w1123) -> (x-y=w1130:dbl)
        n476 = Subtract(x=w1122, y=w1114) -> (x-y=w1121:dbl)
        n477 = Subtract(x=w1140, y=w1132) -> (x-y=w1139:dbl)
        n478 = Subtract(x=w1149, y=w1141) -> (x-y=w1148:dbl)
        n479 = property on="R deg/rev" class="DigNum (strict)"() -> ("Value"=w1115:dbl)  [unwired: 2 in, 2 out]
        n480 = property on="Z mm/rev" class="DigNum (strict)"() -> ("Value"=w1124:dbl)  [unwired: 2 in, 2 out]
        n481 = property on="X mm/rev" class="DigNum (strict)"() -> ("Value"=w1133:dbl)  [unwired: 2 in, 2 out]
        n482 = property on="Y mm/rev" class="DigNum (strict)"() -> ("Value"=w1142:dbl)  [unwired: 2 in, 2 out]
        n483 = Divide(x=w1121, y=w1115) -> (x/y=w1120:dbl)
        n484 = Divide(x=w1139, y=w1133) -> (x/y=w1138:dbl)
        n485 = Divide(x=w1148, y=w1142) -> (x/y=w1147:dbl)
        n486 = Divide(x=w1130, y=w1124) -> (x/y=w1129:dbl)
        n487 = To Double Precision Float(number=w1125) -> (double precision float=w1128:dbl)
        n488 = Multiply(x=w1129, y=w1128) -> (x*y=w1127:dbl)
        n489 = Multiply(x=w1120, y=w1119) -> (x*y=w1118:dbl)
        n490 = Multiply(x=w1138, y=w1137) -> (x*y=w1136:dbl)
        n491 = Multiply(x=w1147, y=w1146) -> (x*y=w1145:dbl)
        n492 = To Long Integer(number=w1127) -> (32bit integer=w1126:i32)
        n493 = To Long Integer(number=w1118) -> (32bit integer=w1117:i32)
        n494 = To Long Integer(number=w1136) -> (32bit integer=w1135:i32)
        n495 = To Long Integer(number=w1145) -> (32bit integer=w1144:i32)
        n496 = property on="Reset Z Motor Steps" class="DigNum (strict)"("Val(Sgnl)"=w1126) -> ()  [unwired: 2 in, 2 out]
        n497 = property on="Reset R Motor Steps" class="DigNum (strict)"("Val(Sgnl)"=w1117) -> ()  [unwired: 2 in, 2 out]
        n498 = property on="Reset X Motor Steps" class="DigNum (strict)"("Val(Sgnl)"=w1135) -> ()  [unwired: 2 in, 2 out]
        n499 = property on="Reset Y Motor Steps" class="DigNum (strict)"("Val(Sgnl)"=w1144) -> ()  [unwired: 2 in, 2 out]
      }
      event "Y Velocity SP step/sec", "X Velocity SP step/sec", "R Velocity SP step/sec", "Z Velocity SP step/sec", "Y Step SP", "X Step SP", "Z Step SP", "R Step SP": Value Change {
        n500 = event-data() -> ()  [unwired: 1 in, 5 out]
        n501 = property on="Y Step SP" class="DigNum (strict)"() -> ("Value"=w1182:i32)  [unwired: 2 in, 2 out]
        n502 = property on="X Step SP" class="DigNum (strict)"() -> ("Value"=w1174:i32)  [unwired: 2 in, 2 out]
        n503 = property on="Z Step SP" class="DigNum (strict)"() -> ("Value"=w1166:i32)  [unwired: 2 in, 2 out]
        n504 = property on="R Step SP" class="DigNum (strict)"() -> ("Value"=w1158:i32)  [unwired: 2 in, 2 out]
        n505 = property on="Y steps/rev" class="DigNum (strict)"() -> ("Value"=w1205:u32)  [unwired: 2 in, 2 out]
        n506 = property on="Y steps/rev" class="DigNum (strict)"() -> ("Value"=w1180:u32)  [unwired: 2 in, 2 out]
        n507 = property on="X steps/rev" class="DigNum (strict)"() -> ("Value"=w1199:u32)  [unwired: 2 in, 2 out]
        n508 = property on="X steps/rev" class="DigNum (strict)"() -> ("Value"=w1172:u32)  [unwired: 2 in, 2 out]
        n509 = property on="Z steps/rev" class="DigNum (strict)"() -> ("Value"=w1193:u32)  [unwired: 2 in, 2 out]
        n510 = property on="Z steps/rev" class="DigNum (strict)"() -> ("Value"=w1164:u32)  [unwired: 2 in, 2 out]
        n511 = property on="R steps/rev" class="DigNum (strict)"() -> ("Value"=w1187:u32)  [unwired: 2 in, 2 out]
        n512 = property on="R steps/rev" class="DigNum (strict)"() -> ("Value"=w1156:u32)  [unwired: 2 in, 2 out]
        n513 = property on="Y offset mm" class="DigNum (strict)"() -> ("Value"=w1179:dbl)  [unwired: 2 in, 2 out]
        n514 = property on="X offset mm" class="DigNum (strict)"() -> ("Value"=w1171:dbl)  [unwired: 2 in, 2 out]
        n515 = property on="Z offset mm" class="DigNum (strict)"() -> ("Value"=w1163:dbl)  [unwired: 2 in, 2 out]
        n516 = property on="R offset deg" class="DigNum (strict)"() -> ("Value"=w1155:dbl)  [unwired: 2 in, 2 out]
        n517 = property on="Y Velocity SP step/sec" class="DigNum (strict)"() -> ("Value"=w1207:i32)  [unwired: 2 in, 2 out]
        n518 = property on="X Velocity SP step/sec" class="DigNum (strict)"() -> ("Value"=w1201:i32)  [unwired: 2 in, 2 out]
        n519 = property on="Z Velocity SP step/sec" class="DigNum (strict)"() -> ("Value"=w1195:i32)  [unwired: 2 in, 2 out]
        n520 = property on="R Velocity SP step/sec" class="DigNum (strict)"() -> ("Value"=w1189:i32)  [unwired: 2 in, 2 out]
        n521 = To Double Precision Float(number=w1182) -> (double precision float=w1183:dbl)
        n522 = To Double Precision Float(number=w1180) -> (double precision float=w1186:dbl)
        n523 = To Double Precision Float(number=w1199) -> (double precision float=w1204:dbl)
        n524 = To Double Precision Float(number=w1174) -> (double precision float=w1175:dbl)
        n525 = To Double Precision Float(number=w1172) -> (double precision float=w1178:dbl)
        n526 = To Double Precision Float(number=w1193) -> (double precision float=w1198:dbl)
        n527 = To Double Precision Float(number=w1166) -> (double precision float=w1167:dbl)
        n528 = To Double Precision Float(number=w1164) -> (double precision float=w1170:dbl)
        n529 = To Double Precision Float(number=w1187) -> (double precision float=w1192:dbl)
        n530 = To Double Precision Float(number=w1158) -> (double precision float=w1159:dbl)
        n531 = To Double Precision Float(number=w1156) -> (double precision float=w1162:dbl)
        n532 = Divide(x=w1159, y=w1162) -> (x/y=w1161:dbl)
        n533 = Divide(x=w1183, y=w1186) -> (x/y=w1185:dbl)
        n534 = Divide(x=w1175, y=w1178) -> (x/y=w1177:dbl)
        n535 = Divide(x=w1167, y=w1170) -> (x/y=w1169:dbl)
        n536 = To Double Precision Float(number=w1189) -> (double precision float=w1190:dbl)
        n537 = To Double Precision Float(number=w1207) -> (double precision float=w1208:dbl)
        n538 = To Double Precision Float(number=w1205) -> (double precision float=w1210:dbl)
        n539 = To Double Precision Float(number=w1201) -> (double precision float=w1202:dbl)
        n540 = To Double Precision Float(number=w1195) -> (double precision float=w1196:dbl)
        n541 = property on="R deg/rev" class="DigNum (strict)"() -> ("Value"=w1154:dbl)  [unwired: 2 in, 2 out]
        n542 = property on="Y mm/rev" class="DigNum (strict)"() -> ("Value"=w1151:dbl)  [unwired: 2 in, 2 out]
        n543 = property on="X mm/rev" class="DigNum (strict)"() -> ("Value"=w1152:dbl)  [unwired: 2 in, 2 out]
        n544 = property on="Z mm/rev" class="DigNum (strict)"() -> ("Value"=w1153:dbl)  [unwired: 2 in, 2 out]
        n545 = Divide(x=w1208, y=w1210) -> (x/y=w1209:dbl)
        n546 = Multiply(x=w1185, y=w1151) -> (x*y=w1184:dbl)
        n547 = Divide(x=w1202, y=w1204) -> (x/y=w1203:dbl)
        n548 = Multiply(x=w1177, y=w1152) -> (x*y=w1176:dbl)
        n549 = Divide(x=w1196, y=w1198) -> (x/y=w1197:dbl)
        n550 = Multiply(x=w1169, y=w1153) -> (x*y=w1168:dbl)
        n551 = Divide(x=w1190, y=w1192) -> (x/y=w1191:dbl)
        n552 = Multiply(x=w1161, y=w1154) -> (x*y=w1160:dbl)
        n553 = Multiply(x=w1209, y=w1151) -> (x*y=w1206:dbl)
        n554 = Add(x=w1184, y=w1179) -> (x+y=w1181:dbl)
        n555 = Multiply(x=w1203, y=w1152) -> (x*y=w1200:dbl)
        n556 = Add(x=w1176, y=w1171) -> (x+y=w1173:dbl)
        n557 = Multiply(x=w1197, y=w1153) -> (x*y=w1194:dbl)
        n558 = Add(x=w1168, y=w1163) -> (x+y=w1165:dbl)
        n559 = Multiply(x=w1191, y=w1154) -> (x*y=w1188:dbl)
        n560 = Add(x=w1160, y=w1155) -> (x+y=w1157:dbl)
        n561 = Absolute Value(x=w1188) -> (abs(x)=w1150:dbl)
        n562 = property on="Y Velocity MV mm/sec" class="DigNum (strict)"("Val(Sgnl)"=w1206) -> ()  [unwired: 2 in, 2 out]
        n563 = property on="Y Position MV mm" class="DigNum (strict)"("Val(Sgnl)"=w1181) -> ()  [unwired: 2 in, 2 out]
        n564 = property on="X Velocity MV mm/sec" class="DigNum (strict)"("Val(Sgnl)"=w1200) -> ()  [unwired: 2 in, 2 out]
        n565 = property on="X Position MV mm" class="DigNum (strict)"("Val(Sgnl)"=w1173) -> ()  [unwired: 2 in, 2 out]
        n566 = property on="Z Velocity MV mm/sec" class="DigNum (strict)"("Val(Sgnl)"=w1194) -> ()  [unwired: 2 in, 2 out]
        n567 = property on="Z Position MV mm" class="DigNum (strict)"("Val(Sgnl)"=w1165) -> ()  [unwired: 2 in, 2 out]
        n568 = property on="R Position MV deg" class="DigNum (strict)"("Val(Sgnl)"=w1157) -> ()  [unwired: 2 in, 2 out]
        n569 = property on="R Velocity MVdeg/sec" class="DigNum (strict)"("Val(Sgnl)"=w1150) -> ()  [unwired: 2 in, 2 out]
      }
      event "Y Scan Length SP steps", "Y Scan Velocity SP steps/sec", "X Scan Velocity SP steps/sec", "X Scan Length SP steps", "Z Scan Velocity SP steps/sec", "Z Scan Length SP steps", "R Scan Velocity SP steps/sec", "R Scan Length SP steps": Value Change {
        n570 = event-data() -> ()  [unwired: 1 in, 5 out]
        n571 = property on="X Step PV" class="DigNum (strict)"() -> ("Value"=w1279:i32)  [unwired: 2 in, 2 out]
        n572 = property on="Y Step PV" class="DigNum (strict)"() -> ("Value"=w1265:i32)  [unwired: 2 in, 2 out]
        n573 = property on="Z Step PV" class="DigNum (strict)"() -> ("Value"=w1252:i32)  [unwired: 2 in, 2 out]
        n574 = property on="R Step PV" class="DigNum (strict)"() -> ("Value"=w1238:i32)  [unwired: 2 in, 2 out]
        n575 = property on="X Step SP" class="DigNum (strict)"() -> ("Minimum"=w1286:dbl)  [unwired: 2 in, 2 out]
        n576 = property on="X Step SP" class="DigNum (strict)"() -> ("Maximum"=w1285:dbl)  [unwired: 2 in, 2 out]
        n577 = property on="Y Step SP" class="DigNum (strict)"() -> ("Minimum"=w1272:dbl)  [unwired: 2 in, 2 out]
        n578 = property on="Y Step SP" class="DigNum (strict)"() -> ("Maximum"=w1271:dbl)  [unwired: 2 in, 2 out]
        n579 = property on="Z Step SP" class="DigNum (strict)"() -> ("Minimum"=w1259:dbl)  [unwired: 2 in, 2 out]
        n580 = property on="Z Step SP" class="DigNum (strict)"() -> ("Maximum"=w1258:dbl)  [unwired: 2 in, 2 out]
        n581 = property on="R Step SP" class="DigNum (strict)"() -> ("Minimum"=w1243:dbl)  [unwired: 2 in, 2 out]
        n582 = property on="R Step SP" class="DigNum (strict)"() -> ("Maximum"=w1246:dbl)  [unwired: 2 in, 2 out]
        n583 = property on="Z steps/rev" class="DigNum (strict)"() -> ("Value"=w1254:u32)  [unwired: 2 in, 2 out]
        n584 = property on="R steps/rev" class="DigNum (strict)"() -> ("Value"=w1240:u32)  [unwired: 2 in, 2 out]
        n585 = property on="X steps/rev" class="DigNum (strict)"() -> ("Value"=w1281:u32)  [unwired: 2 in, 2 out]
        n586 = property on="Y steps/rev" class="DigNum (strict)"() -> ("Value"=w1267:u32)  [unwired: 2 in, 2 out]
        n587 = To Double Precision Float(number=w1279) -> (double precision float=w1232:dbl)
        n588 = To Double Precision Float(number=w1265) -> (double precision float=w1231:dbl)
        n589 = To Double Precision Float(number=w1252) -> (double precision float=w1230:dbl)
        n590 = To Double Precision Float(number=w1238) -> (double precision float=w1229:dbl)
        n591 = Subtract(x=w1286, y=w1232) -> (x-y=w1287:dbl)
        n592 = Subtract(x=w1285, y=w1232) -> (x-y=w1284:dbl)
        n593 = Subtract(x=w1272, y=w1231) -> (x-y=w1273:dbl)
        n594 = Subtract(x=w1271, y=w1231) -> (x-y=w1270:dbl)
        n595 = Subtract(x=w1259, y=w1230) -> (x-y=w1260:dbl)
        n596 = Subtract(x=w1258, y=w1230) -> (x-y=w1257:dbl)
        n597 = Subtract(x=w1243, y=w1229) -> (x-y=w1244:dbl)
        n598 = Subtract(x=w1246, y=w1229) -> (x-y=w1245:dbl)
        n599 = property on="Z Scan Length SP steps" class="DigNum (strict)"() -> ("Value"=w1255:i32)  [unwired: 2 in, 2 out]
        n600 = To Double Precision Float(number=w1254) -> (double precision float=w1251:dbl)
        n601 = property on="R Scan Length SP steps" class="DigNum (strict)"() -> ("Value"=w1241:i32)  [unwired: 2 in, 2 out]
        n602 = To Double Precision Float(number=w1240) -> (double precision float=w1237:dbl)
        n603 = To Double Precision Float(number=w1281) -> (double precision float=w1278:dbl)
        n604 = property on="X Scan Length SP steps" class="DigNum (strict)"() -> ("Value"=w1277:i32)  [unwired: 2 in, 2 out]
        n605 = property on="Y Scan Length SP steps" class="DigNum (strict)"() -> ("Value"=w1268:i32)  [unwired: 2 in, 2 out]
        n606 = To Double Precision Float(number=w1267) -> (double precision float=w1222:dbl)
        n607 = property on="Z Scan Velocity SP steps/sec" class="DigNum (strict)"() -> ("Value"=w1250:i32)  [unwired: 2 in, 2 out]
        n608 = property on="R Scan Velocity SP steps/sec" class="DigNum (strict)"() -> ("Value"=w1236:i32)  [unwired: 2 in, 2 out]
        n609 = property on="X Scan Velocity SP steps/sec" class="DigNum (strict)"() -> ("Value"=w1282:i32)  [unwired: 2 in, 2 out]
        n610 = property on="Y Scan Velocity SP steps/sec" class="DigNum (strict)"() -> ("Value"=w1264:i32)  [unwired: 2 in, 2 out]
        n611 = To Double Precision Float(number=w1255) -> (double precision float=w1228:dbl)
        n612 = To Double Precision Float(number=w1241) -> (double precision float=w1226:dbl)
        n613 = property on="X Scan Length SP steps" class="DigNum (strict)"("Minimum"=w1287) -> ()  [unwired: 2 in, 2 out]
        n614 = property on="X Scan Length SP steps" class="DigNum (strict)"("Maximum"=w1284) -> ()  [unwired: 2 in, 2 out]
        n615 = property on="Y Scan Length SP steps" class="DigNum (strict)"("Minimum"=w1273) -> ()  [unwired: 2 in, 2 out]
        n616 = property on="Y Scan Length SP steps" class="DigNum (strict)"("Maximum"=w1270) -> ()  [unwired: 2 in, 2 out]
        n617 = property on="Z Scan Length SP steps" class="DigNum (strict)"("Minimum"=w1260) -> ()  [unwired: 2 in, 2 out]
        n618 = property on="Z Scan Length SP steps" class="DigNum (strict)"("Maximum"=w1257) -> ()  [unwired: 2 in, 2 out]
        n619 = property on="R Scan Length SP steps" class="DigNum (strict)"("Minimum"=w1244) -> ()  [unwired: 2 in, 2 out]
        n620 = property on="R Scan Length SP steps" class="DigNum (strict)"("Maximum"=w1245) -> ()  [unwired: 2 in, 2 out]
        n621 = To Double Precision Float(number=w1277) -> (double precision float=w1217:dbl)
        n622 = To Double Precision Float(number=w1268) -> (double precision float=w1221:dbl)
        n623 = Divide(x=w1226, y=w1237) -> (x/y=w1242:dbl)
        n624 = Divide(x=w1228, y=w1251) -> (x/y=w1256:dbl)
        n625 = Divide(x=w1217, y=w1278) -> (x/y=w1276:dbl)
        n626 = Divide(x=w1221, y=w1222) -> (x/y=w1269:dbl)
        n627 = To Double Precision Float(number=w1236) -> (double precision float=w1225:dbl)
        n628 = property on="R deg/rev" class="DigNum (strict)"() -> ("Value"=w1239:dbl)  [unwired: 2 in, 2 out]
        n629 = To Double Precision Float(number=w1250) -> (double precision float=w1227:dbl)
        n630 = To Double Precision Float(number=w1282) -> (double precision float=w1216:dbl)
        n631 = To Double Precision Float(number=w1264) -> (double precision float=w1220:dbl)
        n632 = property on="Z mm/rev" class="DigNum (strict)"() -> ("Value"=w1253:dbl)  [unwired: 2 in, 2 out]
        n633 = property on="X mm/rev" class="DigNum (strict)"() -> ("Value"=w1280:dbl)  [unwired: 2 in, 2 out]
        n634 = property on="Y mm/rev" class="DigNum (strict)"() -> ("Value"=w1266:dbl)  [unwired: 2 in, 2 out]
        n635 = Multiply(x=w1256, y=w1253) -> (x*y=w1248:dbl)
        n636 = Divide(x=w1228, y=w1227) -> (x/y=w1223:dbl)
        n637 = Divide(x=w1227, y=w1251) -> (x/y=w1249:dbl)
        n638 = Multiply(x=w1242, y=w1239) -> (x*y=w1234:dbl)
        n639 = Divide(x=w1226, y=w1225) -> (x/y=w1224:dbl)
        n640 = Divide(x=w1225, y=w1237) -> (x/y=w1235:dbl)
        n641 = Divide(x=w1217, y=w1216) -> (x/y=w1218:dbl)
        n642 = Divide(x=w1216, y=w1278) -> (x/y=w1283:dbl)
        n643 = Multiply(x=w1280, y=w1276) -> (x*y=w1274:dbl)
        n644 = Multiply(x=w1269, y=w1266) -> (x*y=w1262:dbl)
        n645 = Divide(x=w1221, y=w1220) -> (x/y=w1219:dbl)
        n646 = Divide(x=w1220, y=w1222) -> (x/y=w1263:dbl)
        n647 = Multiply(x=w1253, y=w1249) -> (x*y=w1247:dbl)
        n648 = Multiply(x=w1239, y=w1235) -> (x*y=w1233:dbl)
        n649 = Multiply(x=w1283, y=w1280) -> (x*y=w1275:dbl)
        n650 = Multiply(x=w1266, y=w1263) -> (x*y=w1261:dbl)
        n651 = Absolute Value(x=w1223) -> (abs(x)=→"Z Scan Duration":dbl)
        n652 = Absolute Value(x=w1224) -> (abs(x)=→"R Scan Duration":dbl)
        n653 = Absolute Value(x=w1218) -> (abs(x)=→"X Scan Duration":dbl)
        n654 = Absolute Value(x=w1219) -> (abs(x)=→"Y Scan Duration":dbl)
        n655 = property on="Z Scan length MV mm" class="DigNum (strict)"("Value"=w1248) -> ()  [unwired: 2 in, 2 out]
        n656 = property on="R Scan length MV deg" class="DigNum (strict)"("Value"=w1234) -> ()  [unwired: 2 in, 2 out]
        n657 = property on="X Scan length MV mm" class="DigNum (strict)"("Val(Sgnl)"=w1274) -> ()  [unwired: 2 in, 2 out]
        n658 = property on="Y Scan length MV mm" class="DigNum (strict)"("Value"=w1262) -> ()  [unwired: 2 in, 2 out]
        n659 = Absolute Value(x=w1233) -> (abs(x)=w1215:dbl)
        n660 = property on="Z Scan velocity MV mm/sec" class="DigNum (strict)"("Val(Sgnl)"=w1247) -> ()  [unwired: 2 in, 2 out]
        n661 = property on="X Scan velocity MV mm/sec" class="DigNum (strict)"("Value"=w1275) -> ()  [unwired: 2 in, 2 out]
        n662 = property on="Y Scan velocity MV mm/sec" class="DigNum (strict)"("Val(Sgnl)"=w1261) -> ()  [unwired: 2 in, 2 out]
        n663 = property on="R Scan Velocity SP deg/sec" class="DigNum (strict)"("Val(Sgnl)"=w1215) -> ()  [unwired: 2 in, 2 out]
      }
      event "Y Move Set": Mouse Down {
        n664 = event-data() -> ()  [unwired: 1 in, 7 out]
        n665 = property on="Y Step SP" class="DigNum (strict)"() -> ("Maximum"=w1298:dbl)  [unwired: 2 in, 2 out]
        n666 = property on="Y Step SP" class="DigNum (strict)"() -> ("Minimum"=w1297:dbl)  [unwired: 2 in, 2 out]
        n667 = property on="Y steps/rev" class="DigNum (strict)"() -> ("Value"=w1304:u32)  [unwired: 2 in, 2 out]
        n668 = property on="Y offset mm" class="DigNum (strict)"() -> ("Value"=w1302:dbl)  [unwired: 2 in, 2 out]
        n669 = property on="Y Velocity SP step/sec" class="DigNum (strict)"() -> ("Maximum"=w1291:dbl)  [unwired: 2 in, 2 out]
        n670 = property on="Y Velocity SP step/sec" class="DigNum (strict)"() -> ("Minimum"=w1290:dbl)  [unwired: 2 in, 2 out]
        n671 = property on="Y Position SP mm" class="DigNum (strict)"() -> ("Value"=w1301:dbl)  [unwired: 2 in, 2 out]
        n672 = property on="Y mm/rev" class="DigNum (strict)"() -> ("Value"=w1288:dbl)  [unwired: 2 in, 2 out]
        n673 = property on="Y Velocity SP mm/sec" class="DigNum (strict)"() -> ("Value"=w1295:dbl)  [unwired: 2 in, 2 out]
        n674 = Subtract(x=w1301, y=w1302) -> (x-y=w1305:dbl)
        n675 = Divide(x=w1295, y=w1288) -> (x/y=w1296:dbl)
        n676 = To Double Precision Float(number=w1304) -> (double precision float=w1289:dbl)
        n677 = Divide(x=w1305, y=w1288) -> (x/y=w1306:dbl)
        n678 = Multiply(x=w1296, y=w1289) -> (x*y=w1293:dbl)
        n679 = Multiply(x=w1306, y=w1289) -> (x*y=w1300:dbl)
        n680 = In Range and Coerce(upper limit=w1291, x=w1293, lower limit=w1290) -> (coerced(x)=w1292:dbl)  [unwired: 1 out]
        n681 = To Long Integer(number=w1292) -> (32bit integer=w1294:i32)
        n682 = In Range and Coerce(upper limit=w1298, x=w1300, lower limit=w1297) -> (coerced(x)=w1299:dbl)  [unwired: 1 out]
        n683 = To Long Integer(number=w1299) -> (32bit integer=w1303:i32)
        n684 = property on="Y Velocity SP step/sec" class="DigNum (strict)"("Val(Sgnl)"=w1294) -> ()  [unwired: 2 in, 2 out]
        n685 = property on="Y Step SP" class="DigNum (strict)"("Val(Sgnl)"=w1303) -> ()  [unwired: 2 in, 2 out]
      }
      event "X Move Set": Mouse Down {
        n686 = event-data() -> ()  [unwired: 1 in, 7 out]
        n687 = property on="X Step SP" class="DigNum (strict)"() -> ("Maximum"=w1317:dbl)  [unwired: 2 in, 2 out]
        n688 = property on="X Step SP" class="DigNum (strict)"() -> ("Minimum"=w1316:dbl)  [unwired: 2 in, 2 out]
        n689 = property on="X steps/rev" class="DigNum (strict)"() -> ("Value"=w1323:u32)  [unwired: 2 in, 2 out]
        n690 = property on="X offset mm" class="DigNum (strict)"() -> ("Value"=w1321:dbl)  [unwired: 2 in, 2 out]
        n691 = property on="X Velocity SP step/sec" class="DigNum (strict)"() -> ("Maximum"=w1310:dbl)  [unwired: 2 in, 2 out]
        n692 = property on="X Velocity SP step/sec" class="DigNum (strict)"() -> ("Minimum"=w1309:dbl)  [unwired: 2 in, 2 out]
        n693 = property on="X Position SP mm" class="DigNum (strict)"() -> ("Value"=w1320:dbl)  [unwired: 2 in, 2 out]
        n694 = property on="X mm/rev" class="DigNum (strict)"() -> ("Value"=w1307:dbl)  [unwired: 2 in, 2 out]
        n695 = property on="X Velocity SP mm/sec" class="DigNum (strict)"() -> ("Value"=w1314:dbl)  [unwired: 2 in, 2 out]
        n696 = Subtract(x=w1320, y=w1321) -> (x-y=w1324:dbl)
        n697 = Divide(x=w1314, y=w1307) -> (x/y=w1315:dbl)
        n698 = To Double Precision Float(number=w1323) -> (double precision float=w1308:dbl)
        n699 = Divide(x=w1324, y=w1307) -> (x/y=w1325:dbl)
        n700 = Multiply(x=w1315, y=w1308) -> (x*y=w1312:dbl)
        n701 = Multiply(x=w1325, y=w1308) -> (x*y=w1319:dbl)
        n702 = In Range and Coerce(upper limit=w1310, x=w1312, lower limit=w1309) -> (coerced(x)=w1311:dbl)  [unwired: 1 out]
        n703 = To Long Integer(number=w1311) -> (32bit integer=w1313:i32)
        n704 = In Range and Coerce(upper limit=w1317, x=w1319, lower limit=w1316) -> (coerced(x)=w1318:dbl)  [unwired: 1 out]
        n705 = To Long Integer(number=w1318) -> (32bit integer=w1322:i32)
        n706 = property on="X Velocity SP step/sec" class="DigNum (strict)"("Val(Sgnl)"=w1313) -> ()  [unwired: 2 in, 2 out]
        n707 = property on="X Step SP" class="DigNum (strict)"("Val(Sgnl)"=w1322) -> ()  [unwired: 2 in, 2 out]
      }
      event "Z Move Set": Mouse Down {
        n708 = event-data() -> ()  [unwired: 1 in, 7 out]
        n709 = property on="Z Step SP" class="DigNum (strict)"() -> ("Maximum"=w1334:dbl)  [unwired: 2 in, 2 out]
        n710 = property on="Z Step SP" class="DigNum (strict)"() -> ("Minimum"=w1333:dbl)  [unwired: 2 in, 2 out]
        n711 = property on="Z steps/rev" class="DigNum (strict)"() -> ("Value"=w1340:u32)  [unwired: 2 in, 2 out]
        n712 = property on="Z offset mm" class="DigNum (strict)"() -> ("Value"=w1338:dbl)  [unwired: 2 in, 2 out]
        n713 = property on="Z Velocity SP step/sec" class="DigNum (strict)"() -> ("Maximum"=w1327:dbl)  [unwired: 2 in, 2 out]
        n714 = property on="Z Velocity SP step/sec" class="DigNum (strict)"() -> ("Minimum"=w1326:dbl)  [unwired: 2 in, 2 out]
        n715 = property on="Z Position SP mm" class="DigNum (strict)"() -> ("Value"=w1337:dbl)  [unwired: 2 in, 2 out]
        n716 = property on="Z mm/rev" class="DigNum (strict)"() -> ("Value"=w1343:dbl)  [unwired: 2 in, 2 out]
        n717 = property on="Z Velocity SP mm/sec" class="DigNum (strict)"() -> ("Value"=w1331:dbl)  [unwired: 2 in, 2 out]
        n718 = Subtract(x=w1337, y=w1338) -> (x-y=w1341:dbl)
        n719 = Divide(x=w1331, y=w1343) -> (x/y=w1332:dbl)
        n720 = To Double Precision Float(number=w1340) -> (double precision float=w1344:dbl)
        n721 = Divide(x=w1341, y=w1343) -> (x/y=w1342:dbl)
        n722 = Multiply(x=w1332, y=w1344) -> (x*y=w1329:dbl)
        n723 = Multiply(x=w1342, y=w1344) -> (x*y=w1336:dbl)
        n724 = In Range and Coerce(upper limit=w1327, x=w1329, lower limit=w1326) -> (coerced(x)=w1328:dbl)  [unwired: 1 out]
        n725 = To Long Integer(number=w1328) -> (32bit integer=w1330:i32)
        n726 = In Range and Coerce(upper limit=w1334, x=w1336, lower limit=w1333) -> (coerced(x)=w1335:dbl)  [unwired: 1 out]
        n727 = To Long Integer(number=w1335) -> (32bit integer=w1339:i32)
        n728 = property on="Z Velocity SP step/sec" class="DigNum (strict)"("Val(Sgnl)"=w1330) -> ()  [unwired: 2 in, 2 out]
        n729 = property on="Z Step SP" class="DigNum (strict)"("Val(Sgnl)"=w1339) -> ()  [unwired: 2 in, 2 out]
      }
      event "R Move Set": Mouse Down {
        n730 = event-data() -> ()  [unwired: 1 in, 7 out]
        n731 = property on="R Step SP" class="DigNum (strict)"() -> ("Maximum"=w1356:dbl)  [unwired: 2 in, 2 out]
        n732 = property on="R Step SP" class="DigNum (strict)"() -> ("Minimum"=w1355:dbl)  [unwired: 2 in, 2 out]
        n733 = property on="R steps/rev" class="DigNum (strict)"() -> ("Value"=w1362:u32)  [unwired: 2 in, 2 out]
        n734 = property on="R offset deg" class="DigNum (strict)"() -> ("Value"=w1360:dbl)  [unwired: 2 in, 2 out]
        n735 = property on="R Velocity SP step/sec" class="DigNum (strict)"() -> ("Maximum"=w1349:dbl)  [unwired: 2 in, 2 out]
        n736 = property on="R Velocity SP step/sec" class="DigNum (strict)"() -> ("Minimum"=w1348:dbl)  [unwired: 2 in, 2 out]
        n737 = To Double Precision Float(number=w1362) -> (double precision float=w1347:dbl)
        n738 = property on="R Position SP deg" class="DigNum (strict)"() -> ("Value"=w1359:dbl)  [unwired: 2 in, 2 out]
        n739 = property on="R deg/rev" class="DigNum (strict)"() -> ("Value"=w1346:dbl)  [unwired: 2 in, 2 out]
        n740 = property on="R Velocity SP deg/sec" class="DigNum (strict)"() -> ("Value"=w1353:dbl)  [unwired: 2 in, 2 out]
        n741 = Subtract(x=w1359, y=w1360) -> (x-y=w1363:dbl)
        n742 = Divide(x=w1353, y=w1346) -> (x/y=w1354:dbl)
        n743 = Divide(x=w1363, y=w1346) -> (x/y=w1364:dbl)
        n744 = Multiply(x=w1354, y=w1347) -> (x*y=w1351:dbl)
        n745 = Multiply(x=w1364, y=w1347) -> (x*y=w1358:dbl)
        n746 = Absolute Value(x=w1351) -> (abs(x)=w1345:dbl)
        n747 = In Range and Coerce(upper limit=w1356, x=w1358, lower limit=w1355) -> (coerced(x)=w1357:dbl)  [unwired: 1 out]
        n748 = In Range and Coerce(upper limit=w1349, x=w1345, lower limit=w1348) -> (coerced(x)=w1350:dbl)  [unwired: 1 out]
        n749 = To Long Integer(number=w1357) -> (32bit integer=w1361:i32)
        n750 = To Long Integer(number=w1350) -> (32bit integer=w1352:i32)
        n751 = property on="R Step SP" class="DigNum (strict)"("Val(Sgnl)"=w1361) -> ()  [unwired: 2 in, 2 out]
        n752 = property on="R Velocity SP step/sec" class="DigNum (strict)"("Val(Sgnl)"=w1352) -> ()  [unwired: 2 in, 2 out]
      }
      event "Y Scan set": Mouse Down {
        n753 = event-data() -> ()  [unwired: 1 in, 7 out]
        n754 = property on="Y Step SP" class="DigNum (strict)"() -> ("Maximum"=w1374:dbl)  [unwired: 2 in, 2 out]
        n755 = property on="Y Step SP" class="DigNum (strict)"() -> ("Minimum"=w1375:dbl)  [unwired: 2 in, 2 out]
        n756 = property on="Y steps/rev" class="DigNum (strict)"() -> ("Value"=w1380:u32)  [unwired: 2 in, 2 out]
        n757 = To Double Precision Float(number=w1380) -> (double precision float=w1366:dbl)
        n758 = property on="Y Scan Length SP mm" class="DigNum (strict)"() -> ("Value"=w1378:dbl)  [unwired: 2 in, 2 out]
        n759 = property on="Y mm/rev" class="DigNum (strict)"() -> ("Value"=w1365:dbl)  [unwired: 2 in, 2 out]
        n760 = property on="Y Scan Velocity SP steps/sec" class="DigNum (strict)"() -> ("Maximum"=w1368:dbl)  [unwired: 2 in, 2 out]
        n761 = property on="Y Scan Velocity SP steps/sec" class="DigNum (strict)"() -> ("Minimum"=w1367:dbl)  [unwired: 2 in, 2 out]
        n762 = property on="Y Scan Velocity SP mm/sec" class="DigNum (strict)"() -> ("Value"=w1372:dbl)  [unwired: 2 in, 2 out]
        n763 = Divide(x=w1378, y=w1365) -> (x/y=w1381:dbl)
        n764 = Multiply(x=w1381, y=w1366) -> (x*y=w1377:dbl)
        n765 = Divide(x=w1372, y=w1365) -> (x/y=w1373:dbl)
        n766 = Multiply(x=w1373, y=w1366) -> (x*y=w1370:dbl)
        n767 = In Range and Coerce(upper limit=w1374, x=w1377, lower limit=w1375) -> (coerced(x)=w1376:dbl)  [unwired: 1 out]
        n768 = To Long Integer(number=w1376) -> (32bit integer=w1379:i32)
        n769 = In Range and Coerce(upper limit=w1368, x=w1370, lower limit=w1367) -> (coerced(x)=w1369:dbl)  [unwired: 1 out]
        n770 = To Long Integer(number=w1369) -> (32bit integer=w1371:i32)
        n771 = property on="Y Scan Length SP steps" class="DigNum (strict)"("Val(Sgnl)"=w1379) -> ()  [unwired: 2 in, 2 out]
        n772 = property on="Y Scan Velocity SP steps/sec" class="DigNum (strict)"("Val(Sgnl)"=w1371) -> ()  [unwired: 2 in, 2 out]
      }
      event "X Scan set": Mouse Down {
        n773 = event-data() -> ()  [unwired: 1 in, 7 out]
        n774 = property on="X Step SP" class="DigNum (strict)"() -> ("Maximum"=w1391:dbl)  [unwired: 2 in, 2 out]
        n775 = property on="X Step SP" class="DigNum (strict)"() -> ("Minimum"=w1392:dbl)  [unwired: 2 in, 2 out]
        n776 = property on="X steps/rev" class="DigNum (strict)"() -> ("Value"=w1397:u32)  [unwired: 2 in, 2 out]
        n777 = To Double Precision Float(number=w1397) -> (double precision float=w1383:dbl)
        n778 = property on="X Scan Length SP mm" class="DigNum (strict)"() -> ("Value"=w1395:dbl)  [unwired: 2 in, 2 out]
        n779 = property on="X mm/rev" class="DigNum (strict)"() -> ("Value"=w1382:dbl)  [unwired: 2 in, 2 out]
        n780 = property on="X Scan Velocity SP steps/sec" class="DigNum (strict)"() -> ("Maximum"=w1385:dbl)  [unwired: 2 in, 2 out]
        n781 = property on="X Scan Velocity SP steps/sec" class="DigNum (strict)"() -> ("Minimum"=w1384:dbl)  [unwired: 2 in, 2 out]
        n782 = property on="X Scan Velocity SP mm/sec" class="DigNum (strict)"() -> ("Value"=w1389:dbl)  [unwired: 2 in, 2 out]
        n783 = Divide(x=w1395, y=w1382) -> (x/y=w1398:dbl)
        n784 = Multiply(x=w1398, y=w1383) -> (x*y=w1394:dbl)
        n785 = Divide(x=w1389, y=w1382) -> (x/y=w1390:dbl)
        n786 = Multiply(x=w1390, y=w1383) -> (x*y=w1387:dbl)
        n787 = In Range and Coerce(upper limit=w1391, x=w1394, lower limit=w1392) -> (coerced(x)=w1393:dbl)  [unwired: 1 out]
        n788 = To Long Integer(number=w1393) -> (32bit integer=w1396:i32)
        n789 = In Range and Coerce(upper limit=w1385, x=w1387, lower limit=w1384) -> (coerced(x)=w1386:dbl)  [unwired: 1 out]
        n790 = To Long Integer(number=w1386) -> (32bit integer=w1388:i32)
        n791 = property on="X Scan Length SP steps" class="DigNum (strict)"("Val(Sgnl)"=w1396) -> ()  [unwired: 2 in, 2 out]
        n792 = property on="X Scan Velocity SP steps/sec" class="DigNum (strict)"("Val(Sgnl)"=w1388) -> ()  [unwired: 2 in, 2 out]
      }
      event "Z Scan set": Mouse Down {
        n793 = event-data() -> ()  [unwired: 1 in, 7 out]
        n794 = property on="Z Step SP" class="DigNum (strict)"() -> ("Maximum"=w1408:dbl)  [unwired: 2 in, 2 out]
        n795 = property on="Z Step SP" class="DigNum (strict)"() -> ("Minimum"=w1409:dbl)  [unwired: 2 in, 2 out]
        n796 = property on="Z steps/rev" class="DigNum (strict)"() -> ("Value"=w1414:u32)  [unwired: 2 in, 2 out]
        n797 = To Double Precision Float(number=w1414) -> (double precision float=w1400:dbl)
        n798 = property on="Z Scan Length SP mm" class="DigNum (strict)"() -> ("Value"=w1412:dbl)  [unwired: 2 in, 2 out]
        n799 = property on="Z mm/rev" class="DigNum (strict)"() -> ("Value"=w1399:dbl)  [unwired: 2 in, 2 out]
        n800 = property on="Z Scan Velocity SP steps/sec" class="DigNum (strict)"() -> ("Maximum"=w1402:dbl)  [unwired: 2 in, 2 out]
        n801 = property on="Z Scan Velocity SP steps/sec" class="DigNum (strict)"() -> ("Minimum"=w1401:dbl)  [unwired: 2 in, 2 out]
        n802 = property on="Z Scan Velocity SP mm/sec" class="DigNum (strict)"() -> ("Value"=w1406:dbl)  [unwired: 2 in, 2 out]
        n803 = Divide(x=w1412, y=w1399) -> (x/y=w1415:dbl)
        n804 = Multiply(x=w1415, y=w1400) -> (x*y=w1411:dbl)
        n805 = Divide(x=w1406, y=w1399) -> (x/y=w1407:dbl)
        n806 = Multiply(x=w1407, y=w1400) -> (x*y=w1404:dbl)
        n807 = In Range and Coerce(upper limit=w1408, x=w1411, lower limit=w1409) -> (coerced(x)=w1410:dbl)  [unwired: 1 out]
        n808 = To Long Integer(number=w1410) -> (32bit integer=w1413:i32)
        n809 = In Range and Coerce(upper limit=w1402, x=w1404, lower limit=w1401) -> (coerced(x)=w1403:dbl)  [unwired: 1 out]
        n810 = To Long Integer(number=w1403) -> (32bit integer=w1405:i32)
        n811 = property on="Z Scan Length SP steps" class="DigNum (strict)"("Val(Sgnl)"=w1413) -> ()  [unwired: 2 in, 2 out]
        n812 = property on="Z Scan Velocity SP steps/sec" class="DigNum (strict)"("Val(Sgnl)"=w1405) -> ()  [unwired: 2 in, 2 out]
      }
      event "R Scan set": Mouse Down {
        n813 = event-data() -> ()  [unwired: 1 in, 7 out]
        n814 = property on="R Step SP" class="DigNum (strict)"() -> ("Maximum"=w1426:dbl)  [unwired: 2 in, 2 out]
        n815 = property on="R Step SP" class="DigNum (strict)"() -> ("Minimum"=w1427:dbl)  [unwired: 2 in, 2 out]
        n816 = property on="R steps/rev" class="DigNum (strict)"() -> ("Value"=w1432:u32)  [unwired: 2 in, 2 out]
        n817 = property on="R Velocity SP step/sec" class="DigNum (strict)"() -> ("Maximum"=w1420:dbl)  [unwired: 2 in, 2 out]
        n818 = To Double Precision Float(number=w1432) -> (double precision float=w1418:dbl)
        n819 = property on="R Scan Length SP deg" class="DigNum (strict)"() -> ("Value"=w1430:dbl)  [unwired: 2 in, 2 out]
        n820 = property on="R deg/rev" class="DigNum (strict)"() -> ("Value"=w1417:dbl)  [unwired: 2 in, 2 out]
        n821 = property on="R Scan Velocity SP steps/sec" class="DigNum (strict)"() -> ("Minimum"=w1419:dbl)  [unwired: 2 in, 2 out]
        n822 = property on="R Scan Velocity SP deg/sec" class="DigNum (strict)"() -> ("Value"=w1424:dbl)  [unwired: 2 in, 2 out]
        n823 = Divide(x=w1430, y=w1417) -> (x/y=w1433:dbl)
        n824 = Multiply(x=w1433, y=w1418) -> (x*y=w1429:dbl)
        n825 = Divide(x=w1424, y=w1417) -> (x/y=w1425:dbl)
        n826 = Multiply(x=w1425, y=w1418) -> (x*y=w1422:dbl)
        n827 = In Range and Coerce(upper limit=w1426, x=w1429, lower limit=w1427) -> (coerced(x)=w1428:dbl)  [unwired: 1 out]
        n828 = To Long Integer(number=w1428) -> (32bit integer=w1431:i32)
        n829 = Absolute Value(x=w1422) -> (abs(x)=w1416:dbl)
        n830 = property on="R Scan Length SP steps" class="DigNum (strict)"("Val(Sgnl)"=w1431) -> ()  [unwired: 2 in, 2 out]
        n831 = In Range and Coerce(upper limit=w1420, x=w1416, lower limit=w1419) -> (coerced(x)=w1421:dbl)  [unwired: 1 out]
        n832 = To Long Integer(number=w1421) -> (32bit integer=w1423:i32)
        n833 = property on="R Scan Velocity SP steps/sec" class="DigNum (strict)"("Val(Sgnl)"=w1423) -> ()  [unwired: 2 in, 2 out]
      }
      event "Y Go": Mouse Up {
        n834 = event-data() -> ()  [unwired: 1 in, 7 out]
        n835 = flat-sequence {
          tunnel: w1438 -> [w1448]
          tunnel: w1439 -> [w1449]
          tunnel: [w1449] -> w1435
          tunnel: [w1448] -> w1434
          tunnel: [w1452] -> w1437
          tunnel: [w1451] -> w1436
          tunnel: w1435 -> [w1454]
          tunnel: w1434 -> [w1453]
          tunnel: [w1472] -> w1441
          tunnel: [w1471] -> w1440
          tunnel: w1437 -> [w1470]
          tunnel: w1436 -> [w1469]
          tunnel: [w1479] -> w1443
          tunnel: [w1478] -> w1442
          tunnel: w1441 -> [w1477]
          tunnel: w1440 -> [w1476]
          tunnel: [w1485] -> w1444
          tunnel: [w1486] -> w1445
          tunnel: w1443 -> [w1486]
          tunnel: w1442 -> [w1484]
          frame #0 {
            n836 = property on="Scan Go" class="Bool"("DisabledEnum"=T2."Disabled and Grayed Out" ("Disabled")) -> ()  [unwired: 2 in, 2 out]
            n837 = property on="Y Go" class="Bool"("DisabledEnum"=T2."Disabled and Grayed Out" ("Disabled")) -> ()  [unwired: 2 in, 2 out]
          }
          frame #1 {
            n838 = property on="Y Step SP" class="DigNum (strict)"() -> ("Value"=w1462:i32)  [unwired: 2 in, 2 out]
            n839 = property on="Y Step PV" class="DigNum (strict)"() -> ("Value"=w1461:i32)  [unwired: 2 in, 2 out]
            n840 = property on="Y Backlash" class="DigNum (strict)"() -> ("Value"=w1450:i32)  [unwired: 2 in, 2 out]
            n841 = Subtract(x=w1462, y=w1461) -> (x-y=w1460:i32)
            n842 = Sign(1:w1450) -> (0:w1458:i32)
            n843 = Sign(1:w1460) -> (0:w1459:i32)
            n844 = Multiply(x=w1459, y=w1458) -> (x*y=w1457:i32)
            n845 = Equal?(x=w1457, y=1) -> (x = y?=w1455:bool)
            n846 = case shown="False" w1455 {
              tunnel: w1454 -> [w1465 w1467]
              tunnel: w1453 -> [w1464 w1466]
              tunnel: [w1464 w1466] -> w1452
              tunnel: [w1465 w1467] -> w1451
              frame False {
                n847 = property on="Y Backlash corr" class="Bool (strict)"("Val(Sgnl)"=FALSE ("Value (Signaling)")) -> ()  [unwired: 2 in, 2 out]
              }
              frame True {
                n848 = property on="Y Backlash corr" class="Bool (strict)"("Val(Sgnl)"=TRUE ("Value (Signaling)")) -> ()  [unwired: 2 in, 2 out]
              }
            }
          }
          frame #2 {
            # "Velocity Setting"
            n849 = property on="Y Velocity SP step/sec" class="DigNum (strict)"() -> ("Value"=w1473:i32)  [unwired: 2 in, 2 out]
            n850 = Number To Decimal String(number=w1473) -> (decimal integer string=w1474:string)  [unwired: 1 in]
            n851 = call "mDrive Send Command.vi"("error in (no error)"=w1470, "Extra"=w1474, "Command"=T1."Max Velocity", "VISA resource name"=w1469) -> ("error out"=w1471:errorcluster, "VISA resource name out"=w1472:refnum<visa-resource-name>)  [unwired: 3 in, 1 out]
          }
          frame #3 {
            # "Move to Abs Position"
            n852 = property on="Y Step SP" class="DigNum (strict)"() -> ("Value"=w1482:i32)  [unwired: 2 in, 2 out]
            n853 = Number To Decimal String(number=w1482) -> (decimal integer string=w1481:string)  [unwired: 1 in]
            n854 = call "mDrive Send Command.vi"("error in (no error)"=w1476, "Extra"=w1481, "Command"=T1."Move to Absolute Position", "VISA resource name"=w1477) -> ("error out"=w1478:errorcluster, "VISA resource name out"=w1479:refnum<visa-resource-name>)  [unwired: 3 in, 1 out]
          }
          frame #4 {
            n855 = call "Time Delay"("error in (no error)"=w1484, "Delay Time (s)"=0.1) -> ("error out"=w1485:errorcluster)  [unwired: 9 in]
          }
        }
      }
      event "Z Go": Mouse Up {
        n856 = event-data() -> ()  [unwired: 1 in, 7 out]
        n857 = flat-sequence {
          tunnel: w1489 -> [w1501]
          tunnel: w1490 -> [w1502]
          tunnel: [w1502] -> w1492
          tunnel: [w1501] -> w1491
          tunnel: [w1505] -> w1494
          tunnel: [w1504] -> w1493
          tunnel: w1492 -> [w1507]
          tunnel: w1491 -> [w1506]
          tunnel: [w1525] -> w1496
          tunnel: [w1524] -> w1495
          tunnel: w1494 -> [w1523]
          tunnel: w1493 -> [w1522]
          tunnel: [w1532] -> w1498
          tunnel: [w1531] -> w1497
          tunnel: w1496 -> [w1530]
          tunnel: w1495 -> [w1529]
          tunnel: [w1538] -> w1488
          tunnel: [w1539] -> w1487
          tunnel: w1498 -> [w1539]
          tunnel: w1497 -> [w1537]
          frame #0 {
            n858 = property on="Scan Go" class="Bool"("DisabledEnum"=T2."Disabled and Grayed Out" ("Disabled")) -> ()  [unwired: 2 in, 2 out]
            n859 = property on="Z Go" class="Bool"("DisabledEnum"=T2."Disabled and Grayed Out" ("Disabled")) -> ()  [unwired: 2 in, 2 out]
          }
          frame #1 {
            n860 = property on="Z Step SP" class="DigNum (strict)"() -> ("Value"=w1515:i32)  [unwired: 2 in, 2 out]
            n861 = property on="Z Step PV" class="DigNum (strict)"() -> ("Value"=w1514:i32)  [unwired: 2 in, 2 out]
            n862 = property on="Z Backlash" class="DigNum (strict)"() -> ("Value"=w1503:i32)  [unwired: 2 in, 2 out]
            n863 = Subtract(x=w1515, y=w1514) -> (x-y=w1513:i32)
            n864 = Sign(1:w1503) -> (0:w1511:i32)
            n865 = Sign(1:w1513) -> (0:w1512:i32)
            n866 = Multiply(x=w1512, y=w1511) -> (x*y=w1510:i32)
            n867 = Equal?(x=w1510, y=1) -> (x = y?=w1508:bool)
            n868 = case shown="True" w1508 {
              tunnel: w1507 -> [w1518 w1520]
              tunnel: w1506 -> [w1517 w1519]
              tunnel: [w1517 w1519] -> w1505
              tunnel: [w1518 w1520] -> w1504
              frame False {
                n869 = property on="Z Backlash corr" class="Bool (strict)"("Val(Sgnl)"=FALSE ("Value (Signaling)")) -> ()  [unwired: 2 in, 2 out]
              }
              frame True {
                n870 = property on="Z Backlash corr" class="Bool (strict)"("Val(Sgnl)"=TRUE ("Value (Signaling)")) -> ()  [unwired: 2 in, 2 out]
              }
            }
          }
          frame #2 {
            # "Velocity Setting"
            n871 = property on="Z Velocity SP step/sec" class="DigNum (strict)"() -> ("Value"=w1526:i32)  [unwired: 2 in, 2 out]
            n872 = Number To Decimal String(number=w1526) -> (decimal integer string=w1527:string)  [unwired: 1 in]
            n873 = call "mDrive Send Command.vi"("error in (no error)"=w1523, "Extra"=w1527, "Command"=T1."Max Velocity", "VISA resource name"=w1522) -> ("error out"=w1524:errorcluster, "VISA resource name out"=w1525:refnum<visa-resource-name>)  [unwired: 3 in, 1 out]
          }
          frame #3 {
            # "Move to Abs Position"
            n874 = property on="Z Step SP" class="DigNum (strict)"() -> ("Value"=w1535:i32)  [unwired: 2 in, 2 out]
            n875 = Number To Decimal String(number=w1535) -> (decimal integer string=w1534:string)  [unwired: 1 in]
            n876 = call "mDrive Send Command.vi"("error in (no error)"=w1529, "Extra"=w1534, "Command"=T1."Move to Absolute Position", "VISA resource name"=w1530) -> ("error out"=w1531:errorcluster, "VISA resource name out"=w1532:refnum<visa-resource-name>)  [unwired: 3 in, 1 out]
          }
          frame #4 {
            n877 = call "Time Delay28"("error in (no error)"=w1537, "Delay Time (s)"=0.1) -> ("error out"=w1538:errorcluster)  [unwired: 9 in]
          }
        }
      }
      event "R Go": Mouse Up {
        n878 = event-data() -> ()  [unwired: 1 in, 7 out]
        n879 = flat-sequence {
          tunnel: w1542 -> [w1554]
          tunnel: w1543 -> [w1555]
          tunnel: [w1555] -> w1545
          tunnel: [w1554] -> w1544
          tunnel: [w1558] -> w1547
          tunnel: [w1557] -> w1546
          tunnel: w1545 -> [w1560]
          tunnel: w1544 -> [w1559]
          tunnel: [w1578] -> w1549
          tunnel: [w1577] -> w1548
          tunnel: w1547 -> [w1576]
          tunnel: w1546 -> [w1575]
          tunnel: [w1585] -> w1551
          tunnel: [w1584] -> w1550
          tunnel: w1549 -> [w1583]
          tunnel: w1548 -> [w1582]
          tunnel: [w1591] -> w1541
          tunnel: [w1592] -> w1540
          tunnel: w1551 -> [w1592]
          tunnel: w1550 -> [w1590]
          frame #0 {
            n880 = property on="Scan Go" class="Bool"("DisabledEnum"=T2."Disabled and Grayed Out" ("Disabled")) -> ()  [unwired: 2 in, 2 out]
            n881 = property on="R Go" class="Bool"("DisabledEnum"=T2."Disabled and Grayed Out" ("Disabled")) -> ()  [unwired: 2 in, 2 out]
          }
          frame #1 {
            n882 = property on="R Step SP" class="DigNum (strict)"() -> ("Value"=w1568:i32)  [unwired: 2 in, 2 out]
            n883 = property on="R Step PV" class="DigNum (strict)"() -> ("Value"=w1567:i32)  [unwired: 2 in, 2 out]
            n884 = property on="R Backlash" class="DigNum (strict)"() -> ("Value"=w1556:i32)  [unwired: 2 in, 2 out]
            n885 = Subtract(x=w1568, y=w1567) -> (x-y=w1566:i32)
            n886 = Sign(1:w1556) -> (0:w1564:i32)
            n887 = Sign(1:w1566) -> (0:w1565:i32)
            n888 = Multiply(x=w1565, y=w1564) -> (x*y=w1563:i32)
            n889 = Equal?(x=w1563, y=1) -> (x = y?=w1561:bool)
            n890 = case shown="True" w1561 {
              tunnel: w1560 -> [w1571 w1573]
              tunnel: w1559 -> [w1570 w1572]
              tunnel: [w1570 w1572] -> w1558
              tunnel: [w1571 w1573] -> w1557
              frame False {
                n891 = property on="R Backlash corr" class="Bool (strict)"("Val(Sgnl)"=FALSE ("Value (Signaling)")) -> ()  [unwired: 2 in, 2 out]
              }
              frame True {
                n892 = property on="R Backlash corr" class="Bool (strict)"("Val(Sgnl)"=TRUE ("Value (Signaling)")) -> ()  [unwired: 2 in, 2 out]
              }
            }
          }
          frame #2 {
            # "Velocity Setting"
            n893 = property on="R Velocity SP step/sec" class="DigNum (strict)"() -> ("Value"=w1579:i32)  [unwired: 2 in, 2 out]
            n894 = Number To Decimal String(number=w1579) -> (decimal integer string=w1580:string)  [unwired: 1 in]
            n895 = call "mDrive Send Command.vi"("error in (no error)"=w1576, "Extra"=w1580, "Command"=T1."Max Velocity", "VISA resource name"=w1575) -> ("error out"=w1577:errorcluster, "VISA resource name out"=w1578:refnum<visa-resource-name>)  [unwired: 3 in, 1 out]
          }
          frame #3 {
            # "Move to Abs Position"
            n896 = property on="R Step SP" class="DigNum (strict)"() -> ("Value"=w1588:i32)  [unwired: 2 in, 2 out]
            n897 = Number To Decimal String(number=w1588) -> (decimal integer string=w1587:string)  [unwired: 1 in]
            n898 = call "mDrive Send Command.vi"("error in (no error)"=w1582, "Extra"=w1587, "Command"=T1."Move to Absolute Position", "VISA resource name"=w1583) -> ("error out"=w1584:errorcluster, "VISA resource name out"=w1585:refnum<visa-resource-name>)  [unwired: 3 in, 1 out]
          }
          frame #4 {
            n899 = call "Time Delay29"("error in (no error)"=w1590, "Delay Time (s)"=0.1) -> ("error out"=w1591:errorcluster)  [unwired: 9 in]
          }
        }
      }
      event "X Go": Mouse Up {
        n900 = event-data() -> ()  [unwired: 1 in, 7 out]
        n901 = flat-sequence {
          tunnel: [w1606] -> w1598
          tunnel: [w1605] -> w1597
          tunnel: w1596 -> [w1606]
          tunnel: w1595 -> [w1605]
          tunnel: [w1611] -> w1600
          tunnel: [w1610] -> w1599
          tunnel: w1598 -> [w1613]
          tunnel: w1597 -> [w1612]
          tunnel: [w1631] -> w1602
          tunnel: [w1630] -> w1601
          tunnel: w1600 -> [w1629]
          tunnel: w1599 -> [w1628]
          tunnel: [w1638] -> w1604
          tunnel: [w1637] -> w1603
          tunnel: w1602 -> [w1636]
          tunnel: w1601 -> [w1635]
          tunnel: [w1644] -> w1593
          tunnel: [w1645] -> w1594
          tunnel: w1604 -> [w1645]
          tunnel: w1603 -> [w1643]
          frame #0 {
            n902 = property on="Scan Go" class="Bool"("DisabledEnum"=T2."Disabled and Grayed Out" ("Disabled")) -> ()  [unwired: 2 in, 2 out]
            n903 = property on="X Go" class="Bool"("DisabledEnum"=T2."Disabled and Grayed Out" ("Disabled")) -> ()  [unwired: 2 in, 2 out]
          }
          frame #1 {
            n904 = property on="X Step SP" class="DigNum (strict)"() -> ("Value"=w1621:i32)  [unwired: 2 in, 2 out]
            n905 = property on="X Step PV" class="DigNum (strict)"() -> ("Value"=w1620:i32)  [unwired: 2 in, 2 out]
            n906 = property on="X Backlash" class="DigNum (strict)"() -> ("Value"=w1609:i32)  [unwired: 2 in, 2 out]
            n907 = Subtract(x=w1621, y=w1620) -> (x-y=w1619:i32)
            n908 = Sign(1:w1609) -> (0:w1617:i32)
            n909 = Sign(1:w1619) -> (0:w1618:i32)
            n910 = Multiply(x=w1618, y=w1617) -> (x*y=w1616:i32)
            n911 = Equal?(x=w1616, y=1) -> (x = y?=w1614:bool)
            n912 = case shown="True" w1614 {
              tunnel: w1613 -> [w1624 w1626]
              tunnel: w1612 -> [w1623 w1625]
              tunnel: [w1623 w1625] -> w1611
              tunnel: [w1624 w1626] -> w1610
              frame False {
                n913 = property on="X Backlash corr" class="Bool (strict)"("Val(Sgnl)"=FALSE ("Value (Signaling)")) -> ()  [unwired: 2 in, 2 out]
              }
              frame True {
                n914 = property on="X Backlash corr" class="Bool (strict)"("Val(Sgnl)"=TRUE ("Value (Signaling)")) -> ()  [unwired: 2 in, 2 out]
              }
            }
          }
          frame #2 {
            # "Velocity Setting"
            n915 = property on="X Velocity SP step/sec" class="DigNum (strict)"() -> ("Value"=w1632:i32)  [unwired: 2 in, 2 out]
            n916 = Number To Decimal String(number=w1632) -> (decimal integer string=w1633:string)  [unwired: 1 in]
            n917 = call "mDrive Send Command.vi"("error in (no error)"=w1629, "Extra"=w1633, "Command"=T1."Max Velocity", "VISA resource name"=w1628) -> ("error out"=w1630:errorcluster, "VISA resource name out"=w1631:refnum<visa-resource-name>)  [unwired: 3 in, 1 out]
          }
          frame #3 {
            # "Move to Abs Position"
            n918 = property on="X Step SP" class="DigNum (strict)"() -> ("Value"=w1641:i32)  [unwired: 2 in, 2 out]
            n919 = Number To Decimal String(number=w1641) -> (decimal integer string=w1640:string)  [unwired: 1 in]
            n920 = call "mDrive Send Command.vi"("error in (no error)"=w1635, "Extra"=w1640, "Command"=T1."Move to Absolute Position", "VISA resource name"=w1636) -> ("error out"=w1637:errorcluster, "VISA resource name out"=w1638:refnum<visa-resource-name>)  [unwired: 3 in, 1 out]
          }
          frame #4 {
            n921 = call "Time Delay15"("error in (no error)"=w1643, "Delay Time (s)"=0.1) -> ("error out"=w1644:errorcluster)  [unwired: 9 in]
          }
        }
      }
      event "X Scan OK": Mouse Up {
        n922 = event-data() -> ()  [unwired: 1 in, 7 out]
        n923 = flat-sequence {
          tunnel: [w1661] -> w1653
          tunnel: [w1659] -> w1652
          tunnel: w1651 -> [w1655]
          tunnel: w1650 -> [w1654]
          tunnel: w1653 -> [w1676]
          tunnel: w1652 -> [w1675]
          tunnel: [w1676] -> w1647
          tunnel: [w1675] -> w1646
          tunnel: [w1678] -> w1648
          tunnel: [w1679] -> w1649
          tunnel: w1647 -> [w1679]
          tunnel: w1646 -> [w1678]
          frame #0 {
            # "VELOCITY"
            n924 = property on="X Scan Velocity SP steps/sec" class="DigNum (strict)"() -> ("Value"=w1662:i32)  [unwired: 2 in, 2 out]
            n925 = Number To Decimal String(number=w1662) -> (decimal integer string=w1663:string)  [unwired: 1 in]
            n926 = call "mDrive Send Command.vi"("error in (no error)"=w1654, "Extra"=w1663, "Command"=T1."Max Velocity", "VISA resource name"=w1655) -> ("error out"=w1664:errorcluster, "VISA resource name out"=w1669:refnum<visa-resource-name>)  [unwired: 3 in, 1 out]
            n927 = call "Time Delay9"("error in (no error)"=w1664) -> ("error out"=w1667:errorcluster)  [unwired: 10 in]
            n928 = call "mDrive Send Command.vi"("error in (no error)"=w1667, "Extra"="VM", "Command"=T1."Print Parameter", "VISA resource name"=w1669) -> ("error out"=w1660:errorcluster, "read buffer"=w1665:string, "VISA resource name out"=w1661:refnum<visa-resource-name>)  [unwired: 3 in]
            n929 = call "Time Delay10"("error in (no error)"=w1660) -> ("error out"=w1659:errorcluster)  [unwired: 10 in]
            n930 = Decimal String To Number(string=w1665, offset=0) -> (number=w1668:i32)  [unwired: 1 in, 1 out]
            n931 = property on="X velocity PV step/sec" class="DigNum (strict)"("Val(Sgnl)"=w1668) -> ()  [unwired: 2 in, 2 out]
          }
          frame #1 {
            n932 = property on="X Scan" class="Bool (strict)"("Val(Sgnl)"=TRUE ("Slew Ready 2")) -> ()  [unwired: 2 in, 2 out]
            n933 = property on="Scan Cancel" class="Bool"("DisabledEnum"=T2."Enabled" ("Disabled")) -> ()  [unwired: 2 in, 2 out]
            n934 = property on="Scan Go" class="Bool"("DisabledEnum"=T2."Enabled" ("Disabled")) -> ()  [unwired: 2 in, 2 out]
            n935 = property on="X Scan Length SP steps" class="DigNum (strict)"("DisabledEnum"=T2."Disabled and Grayed Out" ("Disabled")) -> ()  [unwired: 2 in, 2 out]
            n936 = property on="X Scan Velocity SP steps/sec" class="DigNum (strict)"("DisabledEnum"=T2."Disabled and Grayed Out" ("Disabled")) -> ()  [unwired: 2 in, 2 out]
          }
          frame #2 {
            n937 = property on="X Go" class="Bool"("DisabledEnum"=T2."Disabled and Grayed Out" ("Disabled")) -> ()  [unwired: 2 in, 2 out]
          }
        }
      }
      event "Y Scan OK": Mouse Up {
        n938 = event-data() -> ()  [unwired: 1 in, 7 out]
        n939 = flat-sequence {
          tunnel: w1687 -> [w1697]
          tunnel: w1686 -> [w1696]
          tunnel: [w1693] -> w1684
          tunnel: [w1691] -> w1683
          tunnel: w1684 -> [w1710]
          tunnel: w1683 -> [w1709]
          tunnel: [w1710] -> w1681
          tunnel: [w1709] -> w1680
          tunnel: [w1712] -> w1685
          tunnel: [w1713] -> w1682
          tunnel: w1681 -> [w1713]
          tunnel: w1680 -> [w1712]
          frame #0 {
            # "VELOCITY"
            n940 = property on="Y Scan Velocity SP steps/sec" class="DigNum (strict)"() -> ("Value"=w1694:i32)  [unwired: 2 in, 2 out]
            n941 = Number To Decimal String(number=w1694) -> (decimal integer string=w1695:string)  [unwired: 1 in]
            n942 = call "mDrive Send Command.vi"("error in (no error)"=w1697, "Extra"=w1695, "Command"=T1."Max Velocity", "VISA resource name"=w1696) -> ("error out"=w1698:errorcluster, "VISA resource name out"=w1703:refnum<visa-resource-name>)  [unwired: 3 in, 1 out]
            n943 = call "Time Delay5"("error in (no error)"=w1698) -> ("error out"=w1701:errorcluster)  [unwired: 10 in]
            n944 = call "mDrive Send Command.vi"("error in (no error)"=w1701, "Extra"="VM", "Command"=T1."Print Parameter", "VISA resource name"=w1703) -> ("error out"=w1692:errorcluster, "read buffer"=w1699:string, "VISA resource name out"=w1693:refnum<visa-resource-name>)  [unwired: 3 in]
            n945 = Decimal String To Number(string=w1699, offset=0) -> (number=w1702:i32)  [unwired: 1 in, 1 out]
            n946 = property on="Y velocity PV step/sec" class="DigNum (strict)"("Val(Sgnl)"=w1702) -> ()  [unwired: 2 in, 2 out]
            n947 = call "Time Delay6"("error in (no error)"=w1692) -> ("error out"=w1691:errorcluster)  [unwired: 10 in]
          }
          frame #1 {
            n948 = property on="Y Scan" class="Bool (strict)"("Val(Sgnl)"=TRUE ("Slew Ready 2")) -> ()  [unwired: 2 in, 2 out]
            n949 = property on="Scan Cancel" class="Bool"("DisabledEnum"=T2."Enabled" ("Disabled")) -> ()  [unwired: 2 in, 2 out]
            n950 = property on="Scan Go" class="Bool"("DisabledEnum"=T2."Enabled" ("Disabled")) -> ()  [unwired: 2 in, 2 out]
            n951 = property on="Y Scan Length SP steps" class="DigNum (strict)"("DisabledEnum"=T2."Disabled and Grayed Out" ("Disabled")) -> ()  [unwired: 2 in, 2 out]
            n952 = property on="Y Scan Velocity SP steps/sec" class="DigNum (strict)"("DisabledEnum"=T2."Disabled and Grayed Out" ("Disabled")) -> ()  [unwired: 2 in, 2 out]
          }
          frame #2 {
            n953 = property on="Y Go" class="Bool"("DisabledEnum"=T2."Disabled and Grayed Out" ("Disabled")) -> ()  [unwired: 2 in, 2 out]
          }
        }
      }
      event "Z Scan OK": Mouse Up {
        n954 = event-data() -> ()  [unwired: 1 in, 7 out]
        n955 = flat-sequence {
          tunnel: [w1729] -> w1721
          tunnel: [w1727] -> w1720
          tunnel: w1717 -> [w1723]
          tunnel: w1716 -> [w1722]
          tunnel: w1721 -> [w1744]
          tunnel: w1720 -> [w1743]
          tunnel: [w1744] -> w1719
          tunnel: [w1743] -> w1718
          tunnel: [w1746] -> w1715
          tunnel: [w1747] -> w1714
          tunnel: w1719 -> [w1747]
          tunnel: w1718 -> [w1746]
          frame #0 {
            # "VELOCITY"
            n956 = property on="Z Scan Velocity SP steps/sec" class="DigNum (strict)"() -> ("Value"=w1730:i32)  [unwired: 2 in, 2 out]
            n957 = Number To Decimal String(number=w1730) -> (decimal integer string=w1731:string)  [unwired: 1 in]
            n958 = call "mDrive Send Command.vi"("error in (no error)"=w1722, "Extra"=w1731, "Command"=T1."Max Velocity", "VISA resource name"=w1723) -> ("error out"=w1732:errorcluster, "VISA resource name out"=w1737:refnum<visa-resource-name>)  [unwired: 3 in, 1 out]
            n959 = call "Time Delay24"("error in (no error)"=w1732) -> ("error out"=w1735:errorcluster)  [unwired: 10 in]
            n960 = call "mDrive Send Command.vi"("error in (no error)"=w1735, "Extra"="VM", "Command"=T1."Print Parameter", "VISA resource name"=w1737) -> ("error out"=w1728:errorcluster, "read buffer"=w1733:string, "VISA resource name out"=w1729:refnum<visa-resource-name>)  [unwired: 3 in]
            n961 = Decimal String To Number(string=w1733, offset=0) -> (number=w1736:i32)  [unwired: 1 in, 1 out]
            n962 = property on="Z  velocity PV step/sec" class="DigNum (strict)"("Val(Sgnl)"=w1736) -> ()  [unwired: 2 in, 2 out]
            n963 = call "Time Delay25"("error in (no error)"=w1728) -> ("error out"=w1727:errorcluster)  [unwired: 10 in]
          }
          frame #1 {
            n964 = property on="Z Scan" class="Bool (strict)"("Val(Sgnl)"=TRUE ("Slew Ready 2")) -> ()  [unwired: 2 in, 2 out]
            n965 = property on="Scan Cancel" class="Bool"("DisabledEnum"=T2."Enabled" ("Disabled")) -> ()  [unwired: 2 in, 2 out]
            n966 = property on="Scan Go" class="Bool"("DisabledEnum"=T2."Enabled" ("Disabled")) -> ()  [unwired: 2 in, 2 out]
            n967 = property on="Z Scan Length SP steps" class="DigNum (strict)"("DisabledEnum"=T2."Disabled and Grayed Out" ("Disabled")) -> ()  [unwired: 2 in, 2 out]
            n968 = property on="Z Scan Velocity SP steps/sec" class="DigNum (strict)"("DisabledEnum"=T2."Disabled and Grayed Out" ("Disabled")) -> ()  [unwired: 2 in, 2 out]
          }
          frame #2 {
            n969 = property on="Z Go" class="Bool"("DisabledEnum"=T2."Disabled and Grayed Out" ("Disabled")) -> ()  [unwired: 2 in, 2 out]
          }
        }
      }
      event "R Scan OK": Mouse Up {
        n970 = event-data() -> ()  [unwired: 1 in, 7 out]
        n971 = flat-sequence {
          tunnel: [w1763] -> w1755
          tunnel: [w1761] -> w1754
          tunnel: w1751 -> [w1757]
          tunnel: w1750 -> [w1756]
          tunnel: w1755 -> [w1778]
          tunnel: w1754 -> [w1777]
          tunnel: [w1778] -> w1753
          tunnel: [w1777] -> w1752
          tunnel: [w1780] -> w1748
          tunnel: [w1781] -> w1749
          tunnel: w1753 -> [w1781]
          tunnel: w1752 -> [w1780]
          frame #0 {
            # "VELOCITY"
            n972 = property on="R Scan Velocity SP steps/sec" class="DigNum (strict)"() -> ("Value"=w1764:i32)  [unwired: 2 in, 2 out]
            n973 = Number To Decimal String(number=w1764) -> (decimal integer string=w1765:string)  [unwired: 1 in]
            n974 = call "mDrive Send Command.vi"("error in (no error)"=w1756, "Extra"=w1765, "Command"=T1."Max Velocity", "VISA resource name"=w1757) -> ("error out"=w1766:errorcluster, "VISA resource name out"=w1771:refnum<visa-resource-name>)  [unwired: 3 in, 1 out]
            n975 = call "Time Delay26"("error in (no error)"=w1766) -> ("error out"=w1769:errorcluster)  [unwired: 10 in]
            n976 = call "mDrive Send Command.vi"("error in (no error)"=w1769, "Extra"="VM", "Command"=T1."Print Parameter", "VISA resource name"=w1771) -> ("error out"=w1762:errorcluster, "read buffer"=w1767:string, "VISA resource name out"=w1763:refnum<visa-resource-name>)  [unwired: 3 in]
            n977 = Decimal String To Number(string=w1767, offset=0) -> (number=w1770:i32)  [unwired: 1 in, 1 out]
            n978 = property on="R velocity PV step/sec" class="DigNum (strict)"("Val(Sgnl)"=w1770) -> ()  [unwired: 2 in, 2 out]
            n979 = call "Time Delay27"("error in (no error)"=w1762) -> ("error out"=w1761:errorcluster)  [unwired: 10 in]
          }
          frame #1 {
            n980 = property on="R Scan" class="Bool (strict)"("Val(Sgnl)"=TRUE ("Slew Ready 2")) -> ()  [unwired: 2 in, 2 out]
            n981 = property on="Scan Cancel" class="Bool"("DisabledEnum"=T2."Enabled" ("Disabled")) -> ()  [unwired: 2 in, 2 out]
            n982 = property on="Scan Go" class="Bool"("DisabledEnum"=T2."Enabled" ("Disabled")) -> ()  [unwired: 2 in, 2 out]
            n983 = property on="R Scan Length SP steps" class="DigNum (strict)"("DisabledEnum"=T2."Disabled and Grayed Out" ("Disabled")) -> ()  [unwired: 2 in, 2 out]
            n984 = property on="R Scan Velocity SP steps/sec" class="DigNum (strict)"("DisabledEnum"=T2."Disabled and Grayed Out" ("Disabled")) -> ()  [unwired: 2 in, 2 out]
          }
          frame #2 {
            n985 = property on="R Go" class="Bool"("DisabledEnum"=T2."Disabled and Grayed Out" ("Disabled")) -> ()  [unwired: 2 in, 2 out]
          }
        }
      }
      event Application Instance Close? {
        n986 = event-data() -> ()  [unwired: 1 in, 4 out]
        n987 = event-data() -> ()  [unwired: 3 in, 1 out]
      }
      event "Stop": Mouse Down {
        n988 = event-data() -> ()  [unwired: 1 in, 7 out]
        n989 = flat-sequence {
          tunnel: [w1813] -> w1795
          tunnel: [w1812] -> w1794
          tunnel: w1793 -> [w1811]
          tunnel: w1792 -> [w1810]
          frame #0 {
            n990 = call "mDrive Send Command.vi"("error in (no error)"=w1810, "Command"=T1."Stop", "VISA resource name"=w1811) -> ("error out"=w1812:errorcluster, "VISA resource name out"=w1813:refnum<visa-resource-name>)  [unwired: 4 in, 1 out]
          }
        }
        n991 = flat-sequence {
          tunnel: w1799 -> [w1819]
          tunnel: w1798 -> [w1818]
          tunnel: [w1817] -> w1797
          tunnel: [w1816] -> w1796
          frame #0 {
            n992 = call "mDrive Send Command.vi"("error in (no error)"=w1818, "Command"=T1."Stop", "VISA resource name"=w1819) -> ("error out"=w1816:errorcluster, "VISA resource name out"=w1817:refnum<visa-resource-name>)  [unwired: 4 in, 1 out]
          }
        }
        n993 = flat-sequence {
          tunnel: [w1808] -> w1789
          tunnel: [w1807] -> w1788
          tunnel: w1791 -> [w1806]
          tunnel: w1790 -> [w1805]
          frame #0 {
            n994 = call "mDrive Send Command.vi"("error in (no error)"=w1805, "Command"=T1."Stop", "VISA resource name"=w1806) -> ("error out"=w1807:errorcluster, "VISA resource name out"=w1808:refnum<visa-resource-name>)  [unwired: 4 in, 1 out]
          }
        }
        n995 = flat-sequence {
          tunnel: w1787 -> [w1804]
          tunnel: w1786 -> [w1803]
          tunnel: [w1802] -> w1785
          tunnel: [w1800] -> _
          tunnel: [w1800] -> w1784
          frame #0 {
            n996 = call "mDrive Send Command.vi"("error in (no error)"=w1803, "Command"=T1."Stop", "VISA resource name"=w1804) -> ("error out"=w1800:errorcluster, "VISA resource name out"=w1802:refnum<visa-resource-name>)  [unwired: 4 in, 1 out]
          }
        }
      }
      event "Scan Cancel": Mouse Down {
        n997 = event-data() -> ()  [unwired: 1 in, 7 out]
        n998 = flat-sequence {
          tunnel: w1835 -> [w1874]
          tunnel: w1834 -> [w1873]
          tunnel: [w1876] -> w1837
          tunnel: [w1875] -> w1836
          tunnel: [w1883] -> w1832
          tunnel: [w1884] -> w1833
          tunnel: w1837 -> [w1884]
          tunnel: w1836 -> [w1883]
          frame #0 {
            n999 = call "mDrive Send Command.vi"("error in (no error)"=w1873, "Command"=T1."Stop", "VISA resource name"=w1874) -> ("error out"=w1875:errorcluster, "VISA resource name out"=w1876:refnum<visa-resource-name>)  [unwired: 4 in, 1 out]
          }
          frame #1 {
            n1000 = property on="X Scan" class="Bool (strict)"("Value"=FALSE ("Slew Ready")) -> ()  [unwired: 2 in, 2 out]
            n1001 = property on="X Scan set" class="Bool"("DisabledEnum"=T2."Enabled" ("Disabled")) -> ()  [unwired: 2 in, 2 out]
            n1002 = property on="X Scan Velocity SP steps/sec" class="DigNum (strict)"("DisabledEnum"=T2."Enabled" ("Disabled")) -> ()  [unwired: 2 in, 2 out]
            n1003 = property on="X Scan Length SP steps" class="DigNum (strict)"("DisabledEnum"=T2."Enabled" ("Disabled")) -> ()  [unwired: 2 in, 2 out]
            n1004 = property on="X Go" class="Bool"("DisabledEnum"=T2."Enabled" ("Disabled")) -> ()  [unwired: 2 in, 2 out]
            n1005 = property on="X Scan OK" class="Bool"("DisabledEnum"=T2."Enabled" ("Disabled")) -> ()  [unwired: 2 in, 2 out]
          }
        }
        n1006 = flat-sequence {
          tunnel: w1843 -> [w1887]
          tunnel: w1842 -> [w1886]
          tunnel: [w1889] -> w1839
          tunnel: [w1888] -> w1838
          tunnel: [w1896] -> w1844
          tunnel: [w1897] -> w1845
          tunnel: w1839 -> [w1897]
          tunnel: w1838 -> [w1896]
          frame #0 {
            n1007 = call "mDrive Send Command.vi"("error in (no error)"=w1886, "Command"=T1."Stop", "VISA resource name"=w1887) -> ("error out"=w1888:errorcluster, "VISA resource name out"=w1889:refnum<visa-resource-name>)  [unwired: 4 in, 1 out]
          }
          frame #1 {
            n1008 = property on="Y Scan" class="Bool (strict)"("Value"=FALSE ("Slew Ready")) -> ()  [unwired: 2 in, 2 out]
            n1009 = property on="Y Go" class="Bool"("DisabledEnum"=T2."Enabled" ("Disabled")) -> ()  [unwired: 2 in, 2 out]
            n1010 = property on="Y Scan Velocity SP steps/sec" class="DigNum (strict)"("DisabledEnum"=T2."Enabled" ("Disabled")) -> ()  [unwired: 2 in, 2 out]
            n1011 = property on="Y Scan set" class="Bool"("DisabledEnum"=T2."Enabled" ("Disabled")) -> ()  [unwired: 2 in, 2 out]
            n1012 = property on="Y Scan OK" class="Bool"("DisabledEnum"=T2."Enabled" ("Disabled")) -> ()  [unwired: 2 in, 2 out]
            n1013 = property on="Y Scan Length SP steps" class="DigNum (strict)"("DisabledEnum"=T2."Enabled" ("Disabled")) -> ()  [unwired: 2 in, 2 out]
          }
        }
        n1014 = flat-sequence {
          tunnel: [w1863] -> w1831
          tunnel: [w1862] -> w1830
          tunnel: w1829 -> [w1860]
          tunnel: w1828 -> [w1859]
          tunnel: [w1870] -> w1826
          tunnel: [w1871] -> w1827
          tunnel: w1831 -> [w1871]
          tunnel: w1830 -> [w1870]
          frame #0 {
            n1015 = call "mDrive Send Command.vi"("error in (no error)"=w1859, "Command"=T1."Stop", "VISA resource name"=w1860) -> ("error out"=w1862:errorcluster, "VISA resource name out"=w1863:refnum<visa-resource-name>)  [unwired: 4 in, 1 out]
          }
          frame #1 {
            n1016 = property on="Z Scan" class="Bool (strict)"("Value"=FALSE ("Slew Ready")) -> ()  [unwired: 2 in, 2 out]
            n1017 = property on="Z Scan set" class="Bool"("DisabledEnum"=T2."Enabled" ("Disabled")) -> ()  [unwired: 2 in, 2 out]
            n1018 = property on="Z Scan Velocity SP steps/sec" class="DigNum (strict)"("DisabledEnum"=T2."Enabled" ("Disabled")) -> ()  [unwired: 2 in, 2 out]
            n1019 = property on="Z Scan Length SP steps" class="DigNum (strict)"("DisabledEnum"=T2."Enabled" ("Disabled")) -> ()  [unwired: 2 in, 2 out]
            n1020 = property on="Z Go" class="Bool"("DisabledEnum"=T2."Enabled" ("Disabled")) -> ()  [unwired: 2 in, 2 out]
            n1021 = property on="Z Scan OK" class="Bool"("DisabledEnum"=T2."Enabled" ("Disabled")) -> ()  [unwired: 2 in, 2 out]
          }
        }
        n1022 = flat-sequence {
          tunnel: [w1850] -> w1825
          tunnel: [w1849] -> w1824
          tunnel: w1823 -> [w1847]
          tunnel: w1822 -> [w1846]
          tunnel: [w1857] -> w1820
          tunnel: [w1858] -> w1821
          tunnel: w1825 -> [w1858]
          tunnel: w1824 -> [w1857]
          frame #0 {
            n1023 = call "mDrive Send Command.vi"("error in (no error)"=w1846, "Command"=T1."Stop", "VISA resource name"=w1847) -> ("error out"=w1849:errorcluster, "VISA resource name out"=w1850:refnum<visa-resource-name>)  [unwired: 4 in, 1 out]
          }
          frame #1 {
            n1024 = property on="R Scan" class="Bool (strict)"("Value"=FALSE ("Slew Ready")) -> ()  [unwired: 2 in, 2 out]
            n1025 = property on="R Scan Velocity SP steps/sec" class="DigNum (strict)"("DisabledEnum"=T2."Enabled" ("Disabled")) -> ()  [unwired: 2 in, 2 out]
            n1026 = property on="R Go" class="Bool"("DisabledEnum"=T2."Enabled" ("Disabled")) -> ()  [unwired: 2 in, 2 out]
            n1027 = property on="R Scan OK" class="Bool"("DisabledEnum"=T2."Enabled" ("Disabled")) -> ()  [unwired: 2 in, 2 out]
            n1028 = property on="R Scan Length SP steps" class="DigNum (strict)"("DisabledEnum"=T2."Enabled" ("Disabled")) -> ()  [unwired: 2 in, 2 out]
            n1029 = property on="R Scan set" class="Bool"("DisabledEnum"=T2."Enabled" ("Disabled")) -> ()  [unwired: 2 in, 2 out]
          }
        }
        n1030 = property on="Scan Go" class="Bool"("DisabledEnum"=T2."Disabled and Grayed Out" ("Disabled")) -> ()  [unwired: 2 in, 2 out]
        n1031 = property on="Scan Cancel" class="Bool"("DisabledEnum"=T2."Disabled and Grayed Out" ("Disabled")) -> ()  [unwired: 2 in, 2 out]
      }
      event "Scan Go": Mouse Up {
        n1032 = event-data() -> ()  [unwired: 1 in, 7 out]
        n1033 = flat-sequence {
          tunnel: [w1977] -> w1961
          tunnel: [w1975] -> w1954
          tunnel: [w1976] -> w1951
          tunnel: [w1970] -> w1950
          tunnel: [w1974] -> w1949
          tunnel: [w1973] -> w1948
          tunnel: [w1972] -> w1947
          tunnel: [w1971] -> w1946
          tunnel: w1925 -> [w1969]
          tunnel: [w1969] -> w1924
          tunnel: w1923 -> [w1968]
          tunnel: [w1968] -> w1922
          tunnel: w1921 -> [w1967]
          tunnel: [w1967] -> w1920
          tunnel: w1919 -> [w1966]
          tunnel: [w1966] -> w1918
          tunnel: w1917 -> [w1965]
          tunnel: [w1965] -> w1916
          tunnel: w1915 -> [w1964]
          tunnel: [w1964] -> w1914
          tunnel: [w1963] -> w1913
          tunnel: w1912 -> [w1963]
          tunnel: [w1962] -> w1911
          tunnel: w1910 -> [w1962]
          tunnel: [w2029] -> w1958
          tunnel: [w2028] -> w1956
          tunnel: w1961 -> [w2027]
          tunnel: w1954 -> [w2026]
          tunnel: [w2026] -> w1952
          tunnel: w1951 -> [w2025]
          tunnel: w1950 -> [w2014]
          tunnel: w1949 -> [w2024]
          tunnel: w1948 -> [w2020]
          tunnel: w1947 -> [w2017]
          tunnel: w1946 -> [w2023]
          tunnel: [w2022] -> w1944
          tunnel: [w2021] -> w1942
          tunnel: [w2020] -> w1939
          tunnel: [w2019] -> w1937
          tunnel: [w2018] -> w1935
          tunnel: [w2017] -> w1933
          tunnel: [w2016] -> w1931
          tunnel: [w2015] -> w1929
          tunnel: [w2014] -> w1928
          tunnel: w1924 -> [w2013]
          tunnel: w1922 -> [w2012]
          tunnel: w1920 -> [w2011]
          tunnel: w1918 -> [w2010]
          tunnel: w1916 -> [w2009]
          tunnel: w1914 -> [w2008]
          tunnel: w1913 -> [w2007]
          tunnel: w1911 -> [w2006]
          tunnel: w1958 -> [w2070]
          tunnel: [w2070] -> w1957
          tunnel: w1956 -> [w2069]
          tunnel: [w2069] -> w1955
          tunnel: [w2067] -> w1953
          tunnel: w1952 -> [w2067]
          tunnel: [w2066] -> w1945
          tunnel: w1944 -> [w2066]
          tunnel: [w2065] -> w1943
          tunnel: w1942 -> [w2065]
          tunnel: [w2064] -> w1941
          tunnel: [w2063] -> w1940
          tunnel: w1939 -> [w2063]
          tunnel: [w2062] -> w1938
          tunnel: w1937 -> [w2062]
          tunnel: [w2061] -> w1936
          tunnel: w1935 -> [w2061]
          tunnel: [w2060] -> w1934
          tunnel: w1933 -> [w2060]
          tunnel: [w2059] -> w1932
          tunnel: w1931 -> [w2059]
          tunnel: [w2058] -> w1930
          tunnel: w1929 -> [w2058]
          tunnel: w1928 -> [w2064]
          tunnel: w1957 -> [w2090]
          tunnel: [w2088] -> w1960
          tunnel: w1955 -> [w2089]
          tunnel: [w2087] -> w1959
          tunnel: w1953 -> [w2086]
          tunnel: w1945 -> [w2085]
          tunnel: w1943 -> [w2084]
          tunnel: w1941 -> [w2083]
          tunnel: w1940 -> [w2082]
          tunnel: w1938 -> [w2081]
          tunnel: w1936 -> [w2080]
          tunnel: w1934 -> [w2079]
          tunnel: w1932 -> [w2078]
          tunnel: w1930 -> [w2077]
          tunnel: [w2076] -> w1927
          tunnel: [w2075] -> w1926
          tunnel: [w2074] -> w1905
          tunnel: [w2073] -> w1902
          tunnel: [w2072] -> w1900
          tunnel: [w2071] -> w1898
          tunnel: w1960 -> [w2148]
          tunnel: w1959 -> [w2147]
          tunnel: [w2148] -> w1909
          tunnel: [w2147] -> w1908
          tunnel: [w2141] -> w1907
          tunnel: w1927 -> [w2141]
          tunnel: [w2140] -> w1906
          tunnel: w1926 -> [w2140]
          tunnel: w1905 -> [w2130]
          tunnel: [w2130] -> w1904
          tunnel: [w2129] -> w1903
          tunnel: w1902 -> [w2129]
          tunnel: [w2128] -> w1901
          tunnel: w1900 -> [w2128]
          tunnel: [w2127] -> w1899
          tunnel: w1898 -> [w2127]
          frame #0 {
            n1034 = property on="X Scan" class="Bool (strict)"() -> ("Value"=w1970:bool)  [unwired: 2 in, 2 out]
            n1035 = property on="Y Scan" class="Bool (strict)"() -> ("Value"=w1975:bool)  [unwired: 2 in, 2 out]
            n1036 = property on="Z Scan" class="Bool (strict)"() -> ("Value"=w1972:bool)  [unwired: 2 in, 2 out]
            n1037 = property on="R Scan" class="Bool (strict)"() -> ("Value"=w1973:bool)  [unwired: 2 in, 2 out]
            n1038 = case shown="True" w1970 {
              tunnel: ["" w1993] -> w1976
              frame False {
              }
              frame True {
                n1039 = property on="X Scan Length SP steps" class="DigNum (strict)"() -> ("Value"=w1998:i32)  [unwired: 2 in, 2 out]
                n1040 = Number To Decimal String(number=w1998) -> (decimal integer string=w1995:string)  [unwired: 1 in]
                n1041 = call <vilib>:"Space Constant.vi"() -> ("String"=w1996:string)
                n1042 = Concatenate Strings("MR", w1996, w1995, "\r") -> (w1993:string)
              }
            }
            n1043 = case shown="True" w1975 {
              tunnel: ["" w2000] -> w1977
              frame False {
              }
              frame True {
                n1044 = property on="Y Scan Length SP steps" class="DigNum (strict)"() -> ("Value"=w2005:i32)  [unwired: 2 in, 2 out]
                n1045 = Number To Decimal String(number=w2005) -> (decimal integer string=w2002:string)  [unwired: 1 in]
                n1046 = call <vilib>:"Space Constant.vi"() -> ("String"=w2003:string)
                n1047 = Concatenate Strings("MR", w2003, w2002, "\r") -> (w2000:string)
              }
            }
            n1048 = case shown="True" w1972 {
              tunnel: ["" w1986] -> w1974
              frame False {
              }
              frame True {
                n1049 = property on="Z Scan Length SP steps" class="DigNum (strict)"() -> ("Value"=w1991:i32)  [unwired: 2 in, 2 out]
                n1050 = Number To Decimal String(number=w1991) -> (decimal integer string=w1988:string)  [unwired: 1 in]
                n1051 = call <vilib>:"Space Constant.vi"() -> ("String"=w1989:string)
                n1052 = Concatenate Strings("MR", w1989, w1988, "\r") -> (w1986:string)
              }
            }
            n1053 = case shown="True" w1973 {
              tunnel: ["" w1979] -> w1971
              frame False {
              }
              frame True {
                n1054 = property on="R Scan Length SP steps" class="DigNum (strict)"() -> ("Value"=w1984:i32)  [unwired: 2 in, 2 out]
                n1055 = Number To Decimal String(number=w1984) -> (decimal integer string=w1981:string)  [unwired: 1 in]
                n1056 = call <vilib>:"Space Constant.vi"() -> ("String"=w1982:string)
                n1057 = Concatenate Strings("MR", w1982, w1981, "\r") -> (w1979:string)
              }
            }
          }
          frame #1 {
            n1058 = case shown="False" w2014 {
              tunnel: [w2045 w2050] -> w2022
              tunnel: [w2044 w2049] -> w2021
              tunnel: w2025 -> [_ w2048]
              tunnel: w2013 -> [w2045 w2047]
              tunnel: w2012 -> [w2044 w2046]
              frame False {
              }
              frame True {
                n1059 = VISA Write(VISA resource name=w2047, write buffer=w2048, error in (no error)=w2046) -> (VISA resource name out=w2050:refnum<visa-resource-name>, error out=w2049:errorcluster)  [unwired: 1 out]
              }
            }
            n1060 = case shown="False" w2026 {
              tunnel: [w2052 w2057] -> w2029
              tunnel: [w2051 w2056] -> w2028
              tunnel: w2027 -> [_ w2055]
              tunnel: w2011 -> [w2052 w2054]
              tunnel: w2010 -> [w2051 w2053]
              frame False {
              }
              frame True {
                n1061 = VISA Write(VISA resource name=w2054, write buffer=w2055, error in (no error)=w2053) -> (VISA resource name out=w2057:refnum<visa-resource-name>, error out=w2056:errorcluster)  [unwired: 1 out]
              }
            }
            n1062 = case shown="False" w2017 {
              tunnel: [w2038 w2043] -> w2016
              tunnel: [w2037 w2042] -> w2015
              tunnel: w2024 -> [_ w2041]
              tunnel: w2009 -> [w2038 w2040]
              tunnel: w2008 -> [w2037 w2039]
              frame False {
              }
              frame True {
                n1063 = VISA Write(VISA resource name=w2040, write buffer=w2041, error in (no error)=w2039) -> (VISA resource name out=w2043:refnum<visa-resource-name>, error out=w2042:errorcluster)  [unwired: 1 out]
              }
            }
            n1064 = case shown="False" w2020 {
              tunnel: [w2031 w2036] -> w2019
              tunnel: [w2030 w2035] -> w2018
              tunnel: w2023 -> [_ w2034]
              tunnel: w2007 -> [w2031 w2033]
              tunnel: w2006 -> [w2030 w2032]
              frame False {
              }
              frame True {
                n1065 = VISA Write(VISA resource name=w2033, write buffer=w2034, error in (no error)=w2032) -> (VISA resource name out=w2036:refnum<visa-resource-name>, error out=w2035:errorcluster)  [unwired: 1 out]
              }
            }
          }
          frame #2 {
            n1066 = call "Time Delay7"("Delay Time (s)"=0.1) -> ()  [unwired: 10 in, 1 out]
          }
          frame #3 {
            n1067 = case shown="True" w2083 {
              tunnel: w2085 -> [w2110 w2114]
              tunnel: w2084 -> [w2109 w2113]
              tunnel: [w2110 w2112] -> w2072
              tunnel: [w2109 w2111] -> w2071
              frame False {
              }
              frame True {
                n1068 = property class="Instr"(reference=w2114, error in=w2113) -> (reference out=w2116:refnum<visa-resource-name>, error out=w2115:errorcluster, "Serial Settings:Number of Bytes at Serial Port"=w2117:u32)
                n1069 = VISA Read(VISA resource name=w2116, byte count=w2117, error in (no error)=w2115) -> (VISA resource name out=w2112:refnum<visa-resource-name>, error out=w2111:errorcluster)  [unwired: 2 out]
              }
            }
            n1070 = case shown="True" w2086 {
              tunnel: w2090 -> [w2119 w2123]
              tunnel: w2089 -> [w2118 w2122]
              tunnel: [w2119 w2121] -> w2088
              tunnel: [w2118 w2120] -> w2087
              frame False {
              }
              frame True {
                n1071 = property class="Instr"(reference=w2123, error in=w2122) -> (reference out=w2125:refnum<visa-resource-name>, error out=w2124:errorcluster, "Serial Settings:Number of Bytes at Serial Port"=w2126:u32)
                n1072 = VISA Read(VISA resource name=w2125, byte count=w2126, error in (no error)=w2124) -> (VISA resource name out=w2121:refnum<visa-resource-name>, error out=w2120:errorcluster)  [unwired: 2 out]
              }
            }
            n1073 = case shown="True" w2079 {
              tunnel: w2078 -> [w2092 w2096]
              tunnel: w2077 -> [w2091 w2095]
              tunnel: [w2092 w2094] -> w2076
              tunnel: [w2091 w2093] -> w2075
              frame False {
              }
              frame True {
                n1074 = property class="Instr"(reference=w2096, error in=w2095) -> (reference out=w2098:refnum<visa-resource-name>, error out=w2097:errorcluster, "Serial Settings:Number of Bytes at Serial Port"=w2099:u32)
                n1075 = VISA Read(VISA resource name=w2098, byte count=w2099, error in (no error)=w2097) -> (VISA resource name out=w2094:refnum<visa-resource-name>, error out=w2093:errorcluster)  [unwired: 2 out]
              }
            }
            n1076 = case shown="True" w2082 {
              tunnel: w2081 -> [w2101 w2105]
              tunnel: w2080 -> [w2100 w2104]
              tunnel: [w2101 w2103] -> w2074
              tunnel: [w2100 w2102] -> w2073
              frame False {
              }
              frame True {
                n1077 = property class="Instr"(reference=w2105, error in=w2104) -> (reference out=w2107:refnum<visa-resource-name>, error out=w2106:errorcluster, "Serial Settings:Number of Bytes at Serial Port"=w2108:u32)
                n1078 = VISA Read(VISA resource name=w2107, byte count=w2108, error in (no error)=w2106) -> (VISA resource name out=w2103:refnum<visa-resource-name>, error out=w2102:errorcluster)  [unwired: 2 out]
              }
            }
          }
          frame #4 {
            n1079 = property on="R Scan" class="Bool (strict)"("Val(Sgnl)"=FALSE ("Slew Ready 2")) -> ()  [unwired: 2 in, 2 out]
            n1080 = property on="Z Scan" class="Bool (strict)"("Val(Sgnl)"=FALSE ("Slew Ready 2")) -> ()  [unwired: 2 in, 2 out]
            n1081 = property on="X Scan" class="Bool (strict)"("Val(Sgnl)"=FALSE ("Slew Ready 2")) -> ()  [unwired: 2 in, 2 out]
            n1082 = property on="Y Scan" class="Bool (strict)"("Val(Sgnl)"=FALSE ("Slew Ready 2")) -> ()  [unwired: 2 in, 2 out]
            n1083 = property on="Z Scan Velocity SP steps/sec" class="DigNum (strict)"("DisabledEnum"=T2."Enabled" ("Disabled")) -> ()  [unwired: 2 in, 2 out]
            n1084 = property on="X Scan Length SP steps" class="DigNum (strict)"("DisabledEnum"=T2."Enabled" ("Disabled")) -> ()  [unwired: 2 in, 2 out]
            n1085 = property on="Y Scan Selocity SP steps/sec" class="DigNum (strict)"("DisabledEnum"=T2."Enabled" ("Disabled")) -> ()  [unwired: 2 in, 2 out]
            n1086 = property on="Z Scan Length SP steps" class="DigNum (strict)"("DisabledEnum"=T2."Enabled" ("Disabled")) -> ()  [unwired: 2 in, 2 out]
            n1087 = property on="Y Scan Length SP steps" class="DigNum (strict)"("DisabledEnum"=T2."Enabled" ("Disabled")) -> ()  [unwired: 2 in, 2 out]
            n1088 = property on="X Scan Velocity SP steps/sec" class="DigNum (strict)"("DisabledEnum"=T2."Enabled" ("Disabled")) -> ()  [unwired: 2 in, 2 out]
            n1089 = property on="R Scan Velocity SP steps/sec" class="DigNum (strict)"("DisabledEnum"=T2."Enabled" ("Disabled")) -> ()  [unwired: 2 in, 2 out]
            n1090 = property on="R Scan Length SP steps" class="DigNum (strict)"("DisabledEnum"=T2."Enabled" ("Disabled")) -> ()  [unwired: 2 in, 2 out]
            n1091 = property on="Scan Go" class="Bool"("DisabledEnum"=T2."Disabled and Grayed Out" ("Disabled")) -> ()  [unwired: 2 in, 2 out]
            n1092 = property on="Scan Cancel" class="Bool"("DisabledEnum"=T2."Disabled and Grayed Out" ("Disabled")) -> ()  [unwired: 2 in, 2 out]
          }
        }
      }
      event "Reset": Mouse Down {
        n1093 = event-data() -> ()  [unwired: 1 in, 7 out]
        n1094 = flat-sequence {
          tunnel: [w2179] -> w2158
          tunnel: w2159 -> [w2182]
          tunnel: [w2181] -> w2157
          tunnel: w2160 -> [w2180]
          frame #0 {
            n1095 = property on="Reset X Motor Steps" class="DigNum (strict)"() -> ("Value"=w2183:i32)  [unwired: 2 in, 2 out]
            n1096 = Number To Decimal String(number=w2183) -> (decimal integer string=w2184:string)  [unwired: 1 in]
            n1097 = call "mDrive Send Command.vi"("error in (no error)"=w2182, "Extra"=w2184, "Command"=T1."Set Current Position", "VISA resource name"=w2180) -> ("error out"=w2181:errorcluster, "VISA resource name out"=w2179:refnum<visa-resource-name>)  [unwired: 3 in, 1 out]
          }
        }
        n1098 = flat-sequence {
          tunnel: w2164 -> [w2189]
          tunnel: w2163 -> [w2188]
          tunnel: [w2187] -> w2162
          tunnel: [w2186] -> w2161
          frame #0 {
            n1099 = property on="Reset Y Motor Steps" class="DigNum (strict)"() -> ("Value"=w2190:i32)  [unwired: 2 in, 2 out]
            n1100 = Number To Decimal String(number=w2190) -> (decimal integer string=w2191:string)  [unwired: 1 in]
            n1101 = call "mDrive Send Command.vi"("error in (no error)"=w2188, "Extra"=w2191, "Command"=T1."Set Current Position", "VISA resource name"=w2189) -> ("error out"=w2186:errorcluster, "VISA resource name out"=w2187:refnum<visa-resource-name>)  [unwired: 3 in, 1 out]
          }
        }
        n1102 = flat-sequence {
          tunnel: [w2166] -> w2152
          tunnel: [w2168] -> w2151
          tunnel: w2154 -> [w2167]
          tunnel: w2153 -> [w2165]
          frame #0 {
            n1103 = property on="Reset R Motor Steps" class="DigNum (strict)"() -> ("Value"=w2169:i32)  [unwired: 2 in, 2 out]
            n1104 = Number To Decimal String(number=w2169) -> (decimal integer string=w2170:string)  [unwired: 1 in]
            n1105 = call "mDrive Send Command.vi"("error in (no error)"=w2165, "Extra"=w2170, "Command"=T1."Set Current Position", "VISA resource name"=w2167) -> ("error out"=w2168:errorcluster, "VISA resource name out"=w2166:refnum<visa-resource-name>)  [unwired: 3 in, 1 out]
          }
        }
        n1106 = flat-sequence {
          tunnel: [w2175] -> w2150
          tunnel: [w2174] -> w2149
          tunnel: w2156 -> [w2173]
          tunnel: w2155 -> [w2172]
          frame #0 {
            n1107 = property on="Reset Z Motor Steps" class="DigNum (strict)"() -> ("Value"=w2176:i32)  [unwired: 2 in, 2 out]
            n1108 = Number To Decimal String(number=w2176) -> (decimal integer string=w2177:string)  [unwired: 1 in]
            n1109 = call "mDrive Send Command.vi"("error in (no error)"=w2172, "Extra"=w2177, "Command"=T1."Set Current Position", "VISA resource name"=w2173) -> ("error out"=w2174:errorcluster, "VISA resource name out"=w2175:refnum<visa-resource-name>)  [unwired: 3 in, 1 out]
          }
        }
      }
    }
    n1110 = case shown="True" "Set Button" {
      tunnel: "Preset positions" -> [_ w516]
      frame False {
      }
      frame True {
        n1111 = property on="Presets" class="Arr (strict)"() -> ("Value"=w513:i32[][])  [unwired: 2 in, 2 out]
        n1112 = Index Array(array=w513, index (row)=w516) -> (element=w515:i32[])  [unwired: 1 in]
        n1113 = Array To Cluster(array=w515) -> (cluster=w514:T5)
        n1114 = Unbundle(w514) -> ("Value[0]"=w512:i32, "Value[1]"=w511:i32, "Value[2]"=w510:i32, "Value[3]"=w509:i32)  [unwired: 5 out]
        n1115 = property on="X Step SP" class="DigNum (strict)"("Val(Sgnl)"=w512) -> ()  [unwired: 2 in, 2 out]
        n1116 = property on="Y Step SP" class="DigNum (strict)"("Val(Sgnl)"=w511) -> ()  [unwired: 2 in, 2 out]
        n1117 = property on="Z Step SP" class="DigNum (strict)"("Val(Sgnl)"=w510) -> ()  [unwired: 2 in, 2 out]
        n1118 = property on="R Step SP" class="DigNum (strict)"("Val(Sgnl)"=w509) -> ()  [unwired: 2 in, 2 out]
      }
    }
    n1119 = case shown="True" "Add Button" {
      tunnel: w450 -> [_ w508]
      frame False {
      }
      frame True {
        n1120 = property on="X Step PV" class="DigNum (strict)"() -> ("Value"=w503:i32)  [unwired: 2 in, 2 out]
        n1121 = property on="Y Step PV" class="DigNum (strict)"() -> ("Value"=w502:i32)  [unwired: 2 in, 2 out]
        n1122 = property on="Z Step PV" class="DigNum (strict)"() -> ("Value"=w501:i32)  [unwired: 2 in, 2 out]
        n1123 = property on="R Step PV" class="DigNum (strict)"() -> ("Value"=w500:i32)  [unwired: 2 in, 2 out]
        n1124 = Build Array(w503, w502, w501, w500) -> (w506:i32[])
        n1125 = Build Array (concatenate)(w508, "String") -> (w507:string[])
        n1126 = property on="Preset positions" class="Ring (strict)"("Strings []"=w507) -> ()  [unwired: 2 in, 2 out]
        n1127 = property on="Presets" class="Arr (strict)"() -> ("Value"=w505:i32[][])  [unwired: 2 in, 2 out]
        n1128 = Build Array (concatenate)(w505, w506) -> (w499:i32[][])
        n1129 = property on="Presets" class="Arr (strict)"("Val(Sgnl)"=w499) -> ()  [unwired: 2 in, 2 out]
      }
    }
    n1130 = case shown="True" "Delete Button" {
      tunnel: w450 -> [_ w498]
      frame False {
      }
      frame True {
        n1131 = property on="Preset positions" class="Ring (strict)"() -> ("Value"=w496:i32)  [unwired: 2 in, 2 out]
        n1132 = property on="Presets" class="Arr (strict)"() -> ("Value"=w495:i32[][])  [unwired: 2 in, 2 out]
        n1133 = Delete From Array(array=w498, index=w496) -> (array with subset deleted=w497:string[])  [unwired: 1 in, 1 out]
        n1134 = property on="Preset positions" class="Ring (strict)"("Strings []"=w497) -> ()  [unwired: 2 in, 2 out]
        n1135 = Delete From Array(array=w495, index (row)=w496) -> (array with subset deleted=w494:i32[][])  [unwired: 2 in, 1 out]
        n1136 = property on="Presets" class="Arr (strict)"("Val(Sgnl)"=w494) -> ()  [unwired: 2 in, 2 out]
      }
    }
  }
  n1137 = flat-sequence {
    tunnel: w88 -> [w2198]
    tunnel: w87 -> [w2196]
    tunnel: [w2193] -> w24
    frame #0 {
      n1138 = call "mDrive Send Command.vi"("error in (no error)"=w2196, "Extra"="P", "Command"=T1."Print Parameter", "VISA resource name"=w2198) -> ("error out"=w2195:errorcluster, "read buffer"=w2202:string, "VISA resource name out"=w2197:refnum<visa-resource-name>)  [unwired: 3 in]
      n1139 = call "mDrive Send Command.vi"("error in (no error)"=w2195, "Command"=T1."Stop", "VISA resource name"=w2197) -> ("error out"=w2204:errorcluster, "VISA resource name out"=w2205:refnum<visa-resource-name>)  [unwired: 4 in, 1 out]
      n1140 = Decimal String To Number(string=w2202, offset=0) -> (number=w2194:i32)  [unwired: 1 in, 1 out]
      n1141 = To Long Integer(number=w2194) -> (32bit integer=w2193:i32)
      n1142 = VISA Close(VISA resource name=w2205, error in (no error)=w2204) -> ()  [unwired: 1 out]
    }
  }
  n1143 = flat-sequence {
    tunnel: w28 -> [w2211]
    tunnel: w27 -> [w2209]
    tunnel: [w2206] -> w23
    frame #0 {
      n1144 = call "mDrive Send Command.vi"("error in (no error)"=w2209, "Extra"="P", "Command"=T1."Print Parameter", "VISA resource name"=w2211) -> ("error out"=w2208:errorcluster, "read buffer"=w2215:string, "VISA resource name out"=w2210:refnum<visa-resource-name>)  [unwired: 3 in]
      n1145 = call "mDrive Send Command.vi"("error in (no error)"=w2208, "Command"=T1."Stop", "VISA resource name"=w2210) -> ("error out"=w2217:errorcluster, "VISA resource name out"=w2218:refnum<visa-resource-name>)  [unwired: 4 in, 1 out]
      n1146 = Decimal String To Number(string=w2215, offset=0) -> (number=w2207:i32)  [unwired: 1 in, 1 out]
      n1147 = To Long Integer(number=w2207) -> (32bit integer=w2206:i32)
      n1148 = VISA Close(VISA resource name=w2218, error in (no error)=w2217) -> ()  [unwired: 1 out]
    }
  }
  n1149 = flat-sequence {
    tunnel: w30 -> [w2224]
    tunnel: w29 -> [w2222]
    tunnel: [w2219] -> w22
    frame #0 {
      n1150 = call "mDrive Send Command.vi"("error in (no error)"=w2222, "Extra"="P", "Command"=T1."Print Parameter", "VISA resource name"=w2224) -> ("error out"=w2221:errorcluster, "read buffer"=w2228:string, "VISA resource name out"=w2223:refnum<visa-resource-name>)  [unwired: 3 in]
      n1151 = call "mDrive Send Command.vi"("error in (no error)"=w2221, "Command"=T1."Stop", "VISA resource name"=w2223) -> ("error out"=w2230:errorcluster, "VISA resource name out"=w2231:refnum<visa-resource-name>)  [unwired: 4 in, 1 out]
      n1152 = Decimal String To Number(string=w2228, offset=0) -> (number=w2220:i32)  [unwired: 1 in, 1 out]
      n1153 = To Long Integer(number=w2220) -> (32bit integer=w2219:i32)
      n1154 = VISA Close(VISA resource name=w2231, error in (no error)=w2230) -> ()  [unwired: 1 out]
    }
  }
  n1155 = flat-sequence {
    tunnel: w26 -> [w2237]
    tunnel: w25 -> [w2235]
    tunnel: [w2232] -> w21
    frame #0 {
      n1156 = call "mDrive Send Command.vi"("error in (no error)"=w2235, "Extra"="P", "Command"=T1."Print Parameter", "VISA resource name"=w2237) -> ("error out"=w2234:errorcluster, "read buffer"=w2241:string, "VISA resource name out"=w2236:refnum<visa-resource-name>)  [unwired: 3 in]
      n1157 = call "mDrive Send Command.vi"("error in (no error)"=w2234, "Command"=T1."Stop", "VISA resource name"=w2236) -> ("error out"=w2243:errorcluster, "VISA resource name out"=w2244:refnum<visa-resource-name>)  [unwired: 4 in, 1 out]
      n1158 = Decimal String To Number(string=w2241, offset=0) -> (number=w2233:i32)  [unwired: 1 in, 1 out]
      n1159 = To Long Integer(number=w2233) -> (32bit integer=w2232:i32)
      n1160 = VISA Close(VISA resource name=w2244, error in (no error)=w2243) -> ()  [unwired: 1 out]
    }
  }
  n1161 = flat-sequence {
    tunnel: w24 -> [w2250]
    tunnel: w23 -> [w2249]
    tunnel: w22 -> [w2248]
    tunnel: w21 -> [w2247]
    frame #0 {
      n1162 = Build Array(w2250, w2249, w2248, w2247) -> (w2245:i32[])
      n1163 = call-poly <vilib>:"Write To Spreadsheet File.vi"("1D data"=w2245, "file path (dialog if empty)"=path "S:/SSE/IMS/POS.TXT") -> ()  [unwired: 6 in, 1 out]
    }
    frame #1 {
      n1164 = property on="Presets" class="Arr (strict)"() -> ("Value"=w2257:i32[][])  [unwired: 2 in, 2 out]
      n1165 = property on="Preset positions" class="Ring (strict)"() -> ("Strings []"=w2253:string[])  [unwired: 2 in, 2 out]
      n1166 = Number To Decimal String(number=w2257) -> (decimal integer string=w2251:string[][])  [unwired: 1 in]
      n1167 = Transpose 2D Array(2D array=w2251) -> (transposed array=w2252:string[][])
      n1168 = Build Array (concatenate)(w2253, w2252) -> (w2254:string[][])
      n1169 = Transpose 2D Array(2D array=w2254) -> (transposed array=w2255:string[][])
      n1170 = call-poly <vilib>:"Write To Spreadsheet File.vi"("2D data"=w2255, "file path (dialog if empty)"=path "S:/SSE/IMS/PRESET.TXT") -> ()  [unwired: 6 in, 1 out]
    }
  }
